vi "AgingControl.vi"(0 "IP adress":string="10.0.0.2", 2 "First Channel":u8(ring) items=["1", "2", "3", "4", "5", "6", "7", "8", "9", "10", "11", "12", "13", "14", "15", "16"], 4 "Exit":bool, 6 "Draw 2":enum16{"J(V)", "P(V)", "V(t)", "I(t)"}(ring) caption="Draw") -> (7 "XY Graph":T8(graph)={"ExchangeJVData"=[0.6447156, 0.5940376, 0.5406553, 0.48496604, 0.43833676, 0.39644372, 0.35270205, 0.30110732, 0.2324926, 0.19632894, 0.14613982, 0.08873936, 0.043943465, -0.010401342, -0.04554136, -0.10945036, -0.15922697, -0.20972164, -0.14604181, -0.097304136, -0.048933137, 0.00041567357, 0.047228295, 0.0906797, 0.15038718, 0.20405975, 0.25212517, 0.29427794, 0.3574383, 0.4079635, 0.45813736, 0.5003818, 0.55277103, 0.6010656, 0.64738935, 0.0833232, 0.032125723, -0.00891171, -0.06629689, -0.11847218, -0.16681261, -0.2017693, -0.1451022, -0.09281997, -0.05254645, 0.0022414266, 0.055532034, 0.08567607, 0.35597858, 0.3490164, 0.33783153, 0.32564417, 0.31237674, 0.30614087, 0.2953826, 0.28514028, 0.27568892, 0.2651622, 0.25504795, 0.24763331, 0.23487948, 0.22360058, 0.21352632, 0.20324053, 0.195364, 0.18436247, 0.1724654, 0.1645395, 0.15484014, 0.14352247, 0.13540854, 0.12296967, 0.24092051, 0.2318652, 0.22103643, 0.20964117, 0.20214543, 0.19041994, 0.18028222, 0.1693994, 0.15982696, 0.14702262, 0.14099239, 0.90037847, 0.8003987, 0.700059, 0.6002757, 0.4998595, 0.39971617, 0.299911, 0.19984399, 0.09990792, -0.00039909285, -0.100826114, -0.199933, -0.10054245, -0.0001699818, 0.10008249, 0.19999674, 0.30009645, 0.400098, 0.5005905, 0.59995925, 0.7005827, 0.79998416, 0.9002584, 1.1008824, 1.0004772, 0.9002902, 0.80020136, 0.6998943, 0.59989285, 0.49989128, 0.3998461, 0.2995609, 0.19967936, 0.09944872, -0.00043280495, -0.100914374, -0.1998249, -0.10005248, 3.5971088e-06, 0.100179695, 0.20012668, 0.30028096, 0.40050068, 0.5003604, 0.6004274, 0.700669, 0.8007905, 0.90092295, 1.0009027, 1.1013625], "ExchangeJVData"=[-0.0006814758307882585, -0.0016850824977154844, -0.003464073233772069, -0.004132507456233725, -0.006865448813186958, -0.009688151476439089, -0.010450167610542849, -0.012205285020172596, -0.01281928998650983, -0.01538607757538557, -0.01734554534777999, -0.01874734734883532, -0.02091021160595119, -0.023065433197189122, -0.025690472102724016, -0.027107552159577608, -0.029473809991031885, -0.030340865487232804, -0.02554819220677018, -0.020245595078449696, -0.017617693811189383, -0.014932497288100421, -0.011915947106899694, -0.010568575089564547, -0.00908369620447047, -0.008211866952478886, -0.007987464050529525, -0.005277439777273685, -0.005400622831075452, -0.004535477637546137, -0.0030124019758659415, -0.0015179738511506002, -0.0005382399194786558, 0.0027600066459854133, 0.0038887061236891896, 0.00010727677590693929, -0.00026513666853134055, -0.0005678420166077558, -0.0004885847829427803, -0.0005115025942359352, -0.0008065685506153386, -0.0004981338861398399, -0.0009154278814094141, -0.00034630377285793656, 0.0002839344460880966, -0.00023266989046533126, -0.0003959589321311796, 0.0006277007742028218, 0.0003016369646502426, 0.00021885389287490398, -0.0001957958147613681, 0.00045596452764584683, 0.00025638905754021835, 3.7788979057040706e-05, 0.0003583436637200066, -0.00014885848713674932, 0.00024169821699615568, -4.7932229563230067e-05, 5.387545911617053e-05, 0.000101914599781594, -0.00013739961559622316, 0.0004619877927325433, 3.73482350823906e-05, 7.290014423233515e-05, 3.338896092941468e-06, -0.0003274994242019602, 0.00024382839001191314, -0.0002237818989669904, -4.403914317663293e-05, 4.748494859541097e-05, -0.0005247977696853923, 0.00014040466567166732, 0.0003158870640618261, -0.00019440019514149753, -2.9047253491398806e-06, 0.00012850507573602954, -0.00042629549170669634, 0.000347986610904627, -0.0001858060272752482, 0.00010815821269716253, 9.662588809078443e-05, -0.0001724373305478366, 0.00013225123893789714, 0.028723286231979728, 0.013472377031575888, 0.0038900074287084863, 0.0005599445103143808, -0.00025432843813177897, -0.001567121762491297, -0.00263713354797801, -0.0038046669942559674, -0.004844672366743907, -0.005407297794590704, -0.0060606253100559115, -0.006378423859132454, -0.00500084352097474, -0.004116327909287065, -0.0034220814995933324, -0.002759206108748913, -0.0017260208551306278, -0.0011736246960936114, 0.00019440819869487314, 0.0023596650862600654, 0.005811800292576663, 0.011875201016664505, 0.02630160888656974, 0.25784142781049013, 0.1455090008676052, 0.06033926038071513, 0.018355286738369614, 0.0047029163397382945, 0.0004249142875778489, -0.0016735091776354238, -0.0026023530153906904, -0.003679184737848118, -0.004129284570808522, -0.004831714613828808, -0.0055211869039339945, -0.006160193879622966, -0.006821022543590516, -0.005202024840400554, -0.004168157101958059, -0.0032911433663684875, -0.002357525590923615, -0.0013100188880343921, -0.00010838676871571806, 0.0008879723282007035, 0.0023180647986009717, 0.0050629969337023795, 0.01595134090166539, 0.0550459953956306, 0.13187992153689265, 0.2366785192862153]}, 8 "Number of points":i32=133)   [LabVIEW 2020]
doc: "The VSCAN ( Potentiodynamic Technique) consists of scanning linearly the potential of a stationary working electrode with different scan rates.\nIn general, in this VI, the first thing to do is to start by establishing the connection with the instrument defined by its IP adress, then load the firmware in the channel selected, get the information on the plugged channels, load protocol on a channel, start/stop the protocol, retreive data and draw the graph."
uses:
  ActiveArray.vi
  <vilib>/Utility/file.llb/Write Delimited Spreadsheet (DBL).vi
  <vilib>/Utility/file.llb/Write Delimited Spreadsheet (string).vi
  AgingStatus.vi
  IntensityTemperature.vi
  StartStopPause.vi
panel:
  out "Array 2":string[](array[string])
  out "Array":string[](array[string])
  out "JVData 2":sgl[][](array[numeric])
  in  "DataForAnalysisE":T1 {"Eff" scale=0.0..30.0}
  out "AllPaused":bool
  out "WriteConfigTable":bool
  out "Boolean":bool=TRUE
  out "WriteAll":i32=-1
  out "output array":cluster{"JVData":sgl[][], "AgingData":sgl[][]}[](array[cluster])=[{"JVData"=array133x5[665 elements], "AgingData"=[[0.0, 0.25132346, 0.0, 1.0]]}, {"JVData"=array89x5[445 elements], "AgingData"=array682x3[2046 elements]}, {"JVData"=[[3.07914, 1.0002275, 9.958126e-09, 0.9997951, 1.0], [3.2463598, 0.95003825, 2.1757216e-08, 0.9520022, 1.0], [3.4136999, 0.89984906, 3.7805787e-08, 0.90010446, 1.0], [3.5809798, 0.8496599, -3.234939e-08, 0.8519322, 1.0], [3.74826, 0.7994708, 9.835428e-09, 0.79722506, 1.0], [3.91554, 0.74928164, -5.833279e-08, 0.7560611, 1.0], [4.08288, 0.6990925, -1.44667e-08, 0.6984071, 1.0], [4.2501597, 0.6489033, 1.3045136e-08, 0.64890647, 1.0], [4.41744, 0.5987142, 3.444323e-08, 0.6010701, 1.0], [4.5847797, 0.54852504, -3.4030673e-08, 0.5464241, 1.0], [4.75206, 0.49833587, 5.2020237e-08, 0.49976334, 1.0], [4.9193397, 0.44814673, 5.7064067e-08, 0.4450562, 1.0], [5.08662, 0.39795756, -9.57571e-09, 0.40031934, 1.0], [5.2539597, 0.34776843, 3.5207446e-08, 0.34518468, 1.0], [5.42124, 0.29757926, -2.0274754e-08, 0.30434132, 1.0], [5.58852, 0.2473901, -7.58874e-09, 0.24774085, 1.0], [5.75586, 0.19720097, 4.972759e-08, 0.19575147, 1.0], [5.92314, 0.14701182, -5.5581605e-08, 0.15440427, 1.0], [6.09042, 0.096822664, -3.1738015e-08, 0.099987194, 1.0], [6.2577, 0.046633508, -1.24797355e-08, 0.049051344, 1.0], [6.42504, -0.0035556422, -3.69347e-08, -0.0022356801, 1.0], [6.59232, -0.05374479, -2.699987e-08, -0.04924751, 1.0], [6.7595997, -0.10393394, -3.4336352e-08, -0.100366585, 1.0], [6.92694, -0.15412308, 2.7259583e-08, -0.15919624, 1.0], [7.0798197, -0.20000151, -7.9578044e-08, -0.1976577, 1.0], [7.2471, -0.14981236, -6.108396e-08, -0.1461722, 1.0], [7.4144397, -0.09962321, 4.926905e-08, -0.10051926, 1.0], [7.58172, -0.049434066, -4.2131372e-08, -0.046911426, 1.0], [7.7489996, 0.0007550822, -3.510057e-08, -0.00041872347, 1.0], [7.91628, 0.050944235, 1.0643253e-07, 0.044424977, 1.0], [8.08362, 0.101133384, -2.8528309e-08, 0.10162093, 1.0], [8.250899, 0.15132254, -2.2414564e-08, 0.15435848, 1.0], [8.4181795, 0.20151168, -4.0602938e-08, 0.20494314, 1.0], [8.58552, 0.25170085, -3.418351e-08, 0.25502396, 1.0], [8.7528, 0.30189, -1.1715516e-08, 0.30941048, 1.0], [8.92008, 0.35207915, 4.3308155e-08, 0.3432456, 1.0], [9.087359, 0.4022683, 2.2062904e-08, 0.39781532, 1.0], [9.2547, 0.45245743, -2.3178778e-08, 0.45491967, 1.0], [9.42198, 0.5026466, -6.016691e-08, 0.5006184, 1.0], [9.58926, 0.55283576, -1.1442636e-07, 0.56295985, 1.0]], "AgingData"=array326x3[978 elements]}, {"JVData"=[[3.0790799, 1.0001799, 5.3355116e-09, 0.9998571, 1.0], [3.2463, 0.9499914, -9.22995e-12, 0.9462215, 1.0], [3.41358, 0.8998029, -5.361627e-09, 0.9083466, 1.0], [3.58092, 0.8496145, -2.2642176e-08, 0.84980154, 1.0], [3.7482, 0.799426, 1.0688549e-07, 0.7932258, 1.0], [3.91548, 0.74923754, -1.759565e-08, 0.75158024, 1.0], [4.08276, 0.6990491, -2.914825e-09, 0.70146203, 1.0], [4.2500997, 0.64886063, 4.785635e-08, 0.6504126, 1.0], [4.41738, 0.59867215, 9.625048e-09, 0.5979435, 1.0], [4.58466, 0.54848367, -1.2396183e-08, 0.5513975, 1.0], [4.75194, 0.49829522, 6.345473e-08, 0.491906, 1.0], [4.91928, 0.44810674, 2.2011998e-08, 0.4528098, 1.0], [5.08656, 0.39791828, 4.0515943e-08, 0.3955777, 1.0], [5.25384, 0.3477298, 5.6878946e-08, 0.34668076, 1.0], [5.4211197, 0.29754135, -9.604628e-08, 0.30590534, 1.0], [5.58846, 0.24735287, 9.013345e-09, 0.24722293, 1.0], [5.7557397, 0.1971644, 5.9325743e-08, 0.19342564, 1.0], [5.92302, 0.14697593, -3.028844e-08, 0.15090989, 1.0], [6.0903, 0.09678746, -4.9251167e-08, 0.10161606, 1.0], [6.25764, 0.046598993, 1.4369164e-10, 0.04584945, 1.0], [6.4249196, -0.0035894734, -4.435756e-08, -0.00521524, 1.0], [6.5922, -0.053777937, 2.1317061e-09, -0.05450907, 1.0], [0.5082, -0.6647468, -1.2796141e-08, -0.6640006, 1.0], [1.0162799, -0.6545854, 3.784564e-08, -0.6567539, 1.0]], "AgingData"=array474x3[1422 elements]}, {"JVData"=[[3.0792599, 1.0001653, 5.946803e-09, 1.0001053, 1.0], [3.24648, 0.949974, -6.6066896e-08, 0.95460665, 1.0], [3.41382, 0.89978266, -6.530285e-08, 0.90336657, 1.0], [3.5811, 0.8495914, 8.6590035e-08, 0.84367305, 1.0], [3.7484398, 0.79940003, -2.1140826e-08, 0.7968202, 1.0], [3.91572, 0.7492087, -2.1446452e-08, 0.7541558, 1.0], [4.0829997, 0.6990174, -4.8188134e-08, 0.7052545, 1.0], [4.25034, 0.64882606, 1.1254829e-08, 0.65178263, 1.0], [4.4176197, 0.5986348, -5.8884844e-08, 0.6038444, 1.0], [4.58496, 0.54844344, 4.594265e-08, 0.54645914, 1.0], [4.7522397, 0.4982521, 2.1645896e-08, 0.5013795, 1.0], [4.91952, 0.44806078, 1.5046452e-07, 0.43668732, 1.0], [5.0868597, 0.39786944, -1.6707412e-07, 0.40697056, 1.0], [5.25414, 0.34767812, -4.331764e-09, 0.3509611, 1.0], [5.4214797, 0.2974868, 2.3938037e-08, 0.29353002, 1.0], [5.58876, 0.24729547, -2.5419501e-08, 0.2470593, 1.0], [5.7560396, 0.19710416, 6.9761557e-09, 0.19588034, 1.0], [5.92338, 0.14691283, -6.912309e-08, 0.15127456, 1.0], [6.0906596, 0.0967215, -1.7473404e-08, 0.09949945, 1.0], [6.258, 0.04653018, 1.4005404e-08, 0.04480463, 1.0], [6.4252796, -0.0036611457, -3.703305e-08, -0.0013145087, 1.0], [6.59256, -0.053852465, -5.5675827e-08, -0.051820844, 1.0], [6.7598996, -0.10404379, 5.2207838e-08, -0.10769272, 1.0], [6.92718, -0.15423511, -9.0688665e-09, -0.15569209, 1.0], [7.0801196, -0.20011552, -1.8868072e-09, -0.20259082, 1.0], [7.2474, -0.14992419, 3.1731343e-08, -0.151259, 1.0], [7.4147396, -0.099732876, -1.5792498e-08, -0.098383285, 1.0], [7.58202, -0.049541555, 8.9646235e-08, -0.056819506, 1.0], [7.7493596, 0.00064976525, 2.2409939e-08, -0.0017731013, 1.0], [7.91664, 0.05084109, -3.1073473e-08, 0.055077106, 1.0], [8.08392, 0.10103241, 7.497649e-08, 0.09262056, 1.0], [8.25126, 0.15122373, 2.7147042e-08, 0.15106057, 1.0], [8.41854, 0.20141506, -4.085329e-08, 0.206856, 1.0], [8.585879, 0.2516064, -2.7558846e-08, 0.25670502, 1.0], [8.7531595, 0.30179772, 2.5466141e-08, 0.30317575, 1.0], [8.92044, 0.35198903, -5.1702784e-08, 0.36140174, 1.0], [9.08778, 0.40218034, -4.6354437e-08, 0.40365338, 1.0], [9.25506, 0.4523717, -9.374485e-09, 0.4568654, 1.0], [9.4223995, 0.502563, 9.0104656e-08, 0.49687, 1.0], [9.58968, 0.55275434, 6.764162e-08, 0.5450987, 1.0], [9.75696, 0.6029457, 5.2952487e-09, 0.60003805, 1.0], [9.9243, 0.65313697, -2.9239741e-08, 0.65580297, 1.0], [10.091579, 0.7033283, 9.971579e-11, 0.70409274, 1.0], [3.0948598, -0.5967237, 1.23362565e-08, -0.5965496, 1.0]], "AgingData"=array342x3[1026 elements]}, {"JVData"=[[0.16746, 0.9498421, -3.7238106e-08, 0.9521123, 1.0], [0.3348, 0.899643, -6.0527117e-09, 0.9032217, 1.0], [0.50207996, 0.849444, -6.093289e-08, 0.85836333, 1.0], [0.66942, 0.79924494, -7.89715e-08, 0.80652505, 1.0], [0.83676, 0.7490459, 3.30819e-08, 0.752304, 1.0], [1.0041, 0.6988469, 7.552681e-09, 0.6958531, 1.0]], "AgingData"=[[0.0, -0.27385262, -0.00088946975], [0.0, -0.5112182, 0.0004154984], [2.0, -0.06918946, 7.042664e-05], [4.0, -0.093550734, -8.228485e-05], [0.0, -0.61836976, 5.6613615e-05], [2.0, -0.5800316, -0.00027317417], [4.0, -0.5014493, -4.4106928e-05], [6.0, -0.36604953, -0.00019681842], [8.0, -0.23225343, 3.224882e-05], [10.0, -0.2007136, -4.4106928e-05], [12.0, -0.2059066, 0.00010860457], [14.0, -0.20323373, 0.00010860457], [16.0, -0.21033593, -0.00027317417], [18.0, -0.21904184, 3.224882e-05], [20.0, -0.23691186, 0.00010860457], [22.0, -0.2476797, 3.224882e-05], [0.0, -0.27289036, 7.493925e-05], [2.0, -0.28011072, -2.5781526e-05], [4.0, -0.28629652, -0.000102137274], [6.0, -0.2959952, -2.5781526e-05], [8.0, -0.3174545, -0.000102137274], [10.0, -0.33226982, 0.00020328572], [12.0, -0.37259194, 0.00012692997], [14.0, -0.51142824, 0.00020328572]]}, {"JVData"=[[0.50838, -0.7533297, 3.3713125e-08, -0.754186, 1.0], [1.01658, -0.74316514, -1.8526524e-08, -0.7415677, 1.0], [1.52484, -0.7330006, -1.3213221e-08, -0.730666, 1.0], [2.03304, -0.7228361, -2.0536646e-08, -0.7224946, 1.0], [2.54124, -0.7126715, -4.6319983e-09, -0.7157485, 1.0], [3.0495, -0.70250696, 2.0711987e-08, -0.70280004, 1.0], [3.5577, -0.69234246, -1.360114e-08, -0.69154114, 1.0], [4.06596, -0.6821779, 1.00148485e-08, -0.68209034, 1.0]], "AgingData"=[[0.0, -0.10874961, -0.0005815154], [2.0, -0.37434164, -4.2873908e-05], [4.0, -0.5594564, -0.00011923032], [0.0, -1.571388, -0.0021865703], [2.0, -0.9579511, 0.00010831172], [4.0, -0.8996827, -0.00019711393], [0.0, -0.81472254, -0.0005532635], [2.0, -0.7945132, -0.00024369123], [4.0, -0.7643481, -9.0978414e-05], [6.0, -0.67538, -1.46220045e-05], [8.0, -0.58190614, -9.0978414e-05], [10.0, -0.5370021, -9.0978414e-05], [12.0, -0.53486377, 0.00021444722], [14.0, -0.5418896, -0.00032004766], [16.0, -0.5460135, -9.0978414e-05], [18.0, -0.5487627, -1.46220045e-05], [20.0, -0.5612869, 6.1734405e-05], [22.0, -0.5698401, -1.46220045e-05], [0.0, -0.7470461, -0.0005593721], [2.0, -0.81696755, 0.0001319822], [4.0, -0.88157445, -9.708702e-05], [6.0, -0.9173908, 5.5625802e-05], [8.0, -0.94289756, -0.00017344343], [10.0, -0.9694734, -2.0730608e-05], [12.0, -0.9618367, -9.708702e-05], [14.0, -0.94824326, 0.000284695]]}, {"JVData"=[[0.1674, 0.94984764, -2.53673e-08, 0.95032424, 1.0], [0.33468, 0.89965886, 2.5059206e-08, 0.90274954, 1.0], [0.50202, 0.84947014, 4.599384e-08, 0.8470317, 1.0], [0.66929996, 0.7992814, 2.8115352e-08, 0.80051106, 1.0], [0.83658, 0.7490927, 7.716658e-08, 0.74543494, 1.0], [1.00392, 0.698904, 1.527952e-08, 0.69605744, 1.0], [1.1711999, 0.64871526, -8.1294864e-08, 0.65673256, 1.0], [1.33848, 0.59852654, -2.446165e-09, 0.5987537, 1.0], [1.50576, 0.5483378, 1.2223366e-08, 0.54815394, 1.0], [1.6731, 0.49814907, -1.2237014e-09, 0.4994944, 1.0], [1.84038, 0.44796032, -4.5385075e-08, 0.45431826, 1.0], [2.00766, 0.3977716, 7.518008e-08, 0.39097688, 1.0], [2.1749399, 0.34758288, -7.029272e-08, 0.3521104, 1.0], [2.34228, 0.29739416, -8.037802e-08, 0.30120507, 1.0], [2.5095599, 0.2472054, 1.1764944e-08, 0.25023863, 1.0], [2.6768398, 0.19701669, -3.5605403e-08, 0.2051541, 1.0], [2.84412, 0.14682795, -6.295796e-08, 0.14795439, 1.0], [3.0114598, 0.09663922, -1.0708939e-09, 0.095765725, 1.0], [3.17874, 0.046450496, 3.590854e-08, 0.046586785, 1.0], [3.34602, -0.003738234, 2.9490622e-08, -0.0043338123, 1.0], [3.5133, -0.05392696, -3.8355942e-08, -0.042894743, 1.0], [3.68064, -0.10411569, 2.4600778e-08, -0.10817639, 1.0], [3.84792, -0.15430441, -1.6821268e-09, -0.15341367, 1.0], [3.9998398, -0.19987454, -4.4315435e-08, -0.19512181, 1.0], [4.16712, -0.14968581, -1.1920225e-08, -0.1442165, 1.0], [4.3343997, -0.09949709, 1.1827183e-07, -0.11188886, 1.0], [4.50174, -0.049308363, 3.207719e-09, -0.047019724, 1.0], [4.6690197, 0.00088036037, 1.2209202e-07, -0.00674769, 1.0], [4.8363, 0.05106909, 6.569485e-09, 0.054225642, 1.0], [5.0036397, 0.101257816, 3.5133425e-09, 0.10215181, 1.0], [5.17092, 0.15144655, 1.0848095e-08, 0.15154463, 1.0], [5.3382, 0.20163527, 1.1459326e-08, 0.20368746, 1.0], [5.50548, 0.25182402, -1.7115688e-08, 0.25315666, 1.0], [5.67282, 0.30201274, 6.264987e-08, 0.29463565, 1.0], [5.8401, 0.35220146, 1.7877248e-08, 0.350934, 1.0], [6.00738, 0.40239018, -3.224364e-08, 0.40428376, 1.0], [6.1746597, 0.45257893, 4.8886095e-09, 0.4554946, 1.0], [6.342, 0.5027677, -4.0648054e-08, 0.5062319, 1.0], [6.5092797, 0.5529564, 1.4821096e-08, 0.55712193, 1.0], [6.67656, 0.6031451, -1.3448305e-08, 0.60238975, 1.0], [6.8438396, 0.65333384, -1.1920232e-08, 0.6556937, 1.0], [7.01118, 0.70352256, 1.1764944e-08, 0.7035129, 1.0], [7.1784596, 0.7537113, 7.73194e-08, 0.74700856, 1.0]], "AgingData"=array258x4[1032 elements]}, {"JVData"=[[1.0013499, 1.210579e-05, 1.1001669, 1.0], [2.00265, 5.280055e-06, 1.0000192, 1.0], [3.0038998, 7.4926476e-07, 0.8999563, 1.0], [4.00515, 5.459907e-08, 0.7997196, 1.0], [5.0064, -1.6849775e-07, 0.6995634, 1.0], [6.0077, -3.4968886e-07, 0.5993691, 1.0], [7.0089498, -5.469176e-07, 0.49931043, 1.0], [8.0102, -7.4393e-07, 0.39910764, 1.0], [9.01145, -9.556986e-07, 0.29895997, 1.0], [10.01275, -1.2210978e-06, 0.19898194, 1.0], [11.014, -1.4915547e-06, 0.098842725, 1.0], [12.015249, -1.7013582e-06, -0.0013897662, 1.0], [13.0164995, -1.8637089e-06, -0.101503514, 1.0]], "AgingData"=[[0.2513, 5.4381195e-05, 1.0503782, 1.0], [0.5025, 2.778111e-05, 1.0002986, 1.0], [0.75369996, 3.9110714e-06, 0.94982845, 1.0], [1.0049, -2.2766604e-05, 0.8997149, 1.0], [1.2560999, -5.2547082e-05, 0.8493892, 1.0], [1.5073, -8.9432746e-05, 0.7991992, 1.0], [1.7585, -0.00013286466, 0.74895835, 1.0], [2.0097, -0.00018626524, 0.6987514, 1.0], [2.2609, -0.00024645546, 0.6484681, 1.0], [2.5121, -0.0003150903, 0.5982187, 1.0], [2.7633, -0.0003903196, 0.5479184, 1.0], [3.0144498, -0.00046932563, 0.49767745, 1.0], [3.26565, -0.0005563859, 0.44752148, 1.0], [3.51685, -0.00064487197, 0.397323, 1.0], [3.76805, -0.00073117693, 0.34696326, 1.0], [4.01925, -0.0008170999, 0.29672235, 1.0], [4.27045, -0.0009031756, 0.24646449, 1.0], [4.52165, -0.0009820798, 0.19614716, 1.0], [4.77285, -0.0010612556, 0.14594024, 1.0], [5.0240498, -0.0011366602, 0.0958352, 1.0], [5.27525, -0.0012121152, 0.04556884, 1.0], [5.5264497, -0.0012991133, -0.0047399844, 1.0], [5.77765, -0.0013793214, -0.05493842, 1.0], [6.02885, -0.0014648766, -0.10519629, 1.0], [6.28005, -0.001559259, -0.15536925, 1.0], [6.53125, -0.001651095, -0.20566109, 1.0], [6.7824497, -0.0017487028, -0.255885, 1.0]]}, {"JVData"=[[1.0013499, 1.210579e-05, 1.1001669, 1.0], [2.00265, 5.280055e-06, 1.0000192, 1.0], [3.0038998, 7.4926476e-07, 0.8999563, 1.0], [4.00515, 5.459907e-08, 0.7997196, 1.0], [5.0064, -1.6849775e-07, 0.6995634, 1.0], [6.0077, -3.4968886e-07, 0.5993691, 1.0], [7.0089498, -5.469176e-07, 0.49931043, 1.0], [8.0102, -7.4393e-07, 0.39910764, 1.0], [9.01145, -9.556986e-07, 0.29895997, 1.0], [10.01275, -1.2210978e-06, 0.19898194, 1.0], [11.014, -1.4915547e-06, 0.098842725, 1.0], [12.015249, -1.7013582e-06, -0.0013897662, 1.0], [13.0164995, -1.8637089e-06, -0.101503514, 1.0]], "AgingData"=[[0.2513, 5.4381195e-05, 1.0503782, 1.0], [0.5025, 2.778111e-05, 1.0002986, 1.0], [0.75369996, 3.9110714e-06, 0.94982845, 1.0], [1.0049, -2.2766604e-05, 0.8997149, 1.0], [1.2560999, -5.2547082e-05, 0.8493892, 1.0], [1.5073, -8.9432746e-05, 0.7991992, 1.0], [1.7585, -0.00013286466, 0.74895835, 1.0], [2.0097, -0.00018626524, 0.6987514, 1.0], [2.2609, -0.00024645546, 0.6484681, 1.0], [2.5121, -0.0003150903, 0.5982187, 1.0], [2.7633, -0.0003903196, 0.5479184, 1.0], [3.0144498, -0.00046932563, 0.49767745, 1.0], [3.26565, -0.0005563859, 0.44752148, 1.0], [3.51685, -0.00064487197, 0.397323, 1.0], [3.76805, -0.00073117693, 0.34696326, 1.0], [4.01925, -0.0008170999, 0.29672235, 1.0], [4.27045, -0.0009031756, 0.24646449, 1.0], [4.52165, -0.0009820798, 0.19614716, 1.0], [4.77285, -0.0010612556, 0.14594024, 1.0], [5.0240498, -0.0011366602, 0.0958352, 1.0], [5.27525, -0.0012121152, 0.04556884, 1.0], [5.5264497, -0.0012991133, -0.0047399844, 1.0], [5.77765, -0.0013793214, -0.05493842, 1.0], [6.02885, -0.0014648766, -0.10519629, 1.0], [6.28005, -0.001559259, -0.15536925, 1.0], [6.53125, -0.001651095, -0.20566109, 1.0], [6.7824497, -0.0017487028, -0.255885, 1.0]]}, {"JVData"=[[1.0013499, 1.210579e-05, 1.1001669, 1.0], [2.00265, 5.280055e-06, 1.0000192, 1.0], [3.0038998, 7.4926476e-07, 0.8999563, 1.0], [4.00515, 5.459907e-08, 0.7997196, 1.0], [5.0064, -1.6849775e-07, 0.6995634, 1.0], [6.0077, -3.4968886e-07, 0.5993691, 1.0], [7.0089498, -5.469176e-07, 0.49931043, 1.0], [8.0102, -7.4393e-07, 0.39910764, 1.0], [9.01145, -9.556986e-07, 0.29895997, 1.0], [10.01275, -1.2210978e-06, 0.19898194, 1.0], [11.014, -1.4915547e-06, 0.098842725, 1.0], [12.015249, -1.7013582e-06, -0.0013897662, 1.0], [13.0164995, -1.8637089e-06, -0.101503514, 1.0]], "AgingData"=[[0.2513, 5.4381195e-05, 1.0503782, 1.0], [0.5025, 2.778111e-05, 1.0002986, 1.0], [0.75369996, 3.9110714e-06, 0.94982845, 1.0], [1.0049, -2.2766604e-05, 0.8997149, 1.0], [1.2560999, -5.2547082e-05, 0.8493892, 1.0], [1.5073, -8.9432746e-05, 0.7991992, 1.0], [1.7585, -0.00013286466, 0.74895835, 1.0], [2.0097, -0.00018626524, 0.6987514, 1.0], [2.2609, -0.00024645546, 0.6484681, 1.0], [2.5121, -0.0003150903, 0.5982187, 1.0], [2.7633, -0.0003903196, 0.5479184, 1.0], [3.0144498, -0.00046932563, 0.49767745, 1.0], [3.26565, -0.0005563859, 0.44752148, 1.0], [3.51685, -0.00064487197, 0.397323, 1.0], [3.76805, -0.00073117693, 0.34696326, 1.0], [4.01925, -0.0008170999, 0.29672235, 1.0], [4.27045, -0.0009031756, 0.24646449, 1.0], [4.52165, -0.0009820798, 0.19614716, 1.0], [4.77285, -0.0010612556, 0.14594024, 1.0], [5.0240498, -0.0011366602, 0.0958352, 1.0], [5.27525, -0.0012121152, 0.04556884, 1.0], [5.5264497, -0.0012991133, -0.0047399844, 1.0], [5.77765, -0.0013793214, -0.05493842, 1.0], [6.02885, -0.0014648766, -0.10519629, 1.0], [6.28005, -0.001559259, -0.15536925, 1.0], [6.53125, -0.001651095, -0.20566109, 1.0], [6.7824497, -0.0017487028, -0.255885, 1.0]]}, {"JVData"=[[1.0013499, 1.210579e-05, 1.1001669, 1.0], [2.00265, 5.280055e-06, 1.0000192, 1.0], [3.0038998, 7.4926476e-07, 0.8999563, 1.0], [4.00515, 5.459907e-08, 0.7997196, 1.0], [5.0064, -1.6849775e-07, 0.6995634, 1.0], [6.0077, -3.4968886e-07, 0.5993691, 1.0], [7.0089498, -5.469176e-07, 0.49931043, 1.0], [8.0102, -7.4393e-07, 0.39910764, 1.0], [9.01145, -9.556986e-07, 0.29895997, 1.0], [10.01275, -1.2210978e-06, 0.19898194, 1.0], [11.014, -1.4915547e-06, 0.098842725, 1.0], [12.015249, -1.7013582e-06, -0.0013897662, 1.0], [13.0164995, -1.8637089e-06, -0.101503514, 1.0]], "AgingData"=[[0.2513, 5.4381195e-05, 1.0503782, 1.0], [0.5025, 2.778111e-05, 1.0002986, 1.0], [0.75369996, 3.9110714e-06, 0.94982845, 1.0], [1.0049, -2.2766604e-05, 0.8997149, 1.0], [1.2560999, -5.2547082e-05, 0.8493892, 1.0], [1.5073, -8.9432746e-05, 0.7991992, 1.0], [1.7585, -0.00013286466, 0.74895835, 1.0], [2.0097, -0.00018626524, 0.6987514, 1.0], [2.2609, -0.00024645546, 0.6484681, 1.0], [2.5121, -0.0003150903, 0.5982187, 1.0], [2.7633, -0.0003903196, 0.5479184, 1.0], [3.0144498, -0.00046932563, 0.49767745, 1.0], [3.26565, -0.0005563859, 0.44752148, 1.0], [3.51685, -0.00064487197, 0.397323, 1.0], [3.76805, -0.00073117693, 0.34696326, 1.0], [4.01925, -0.0008170999, 0.29672235, 1.0], [4.27045, -0.0009031756, 0.24646449, 1.0], [4.52165, -0.0009820798, 0.19614716, 1.0], [4.77285, -0.0010612556, 0.14594024, 1.0], [5.0240498, -0.0011366602, 0.0958352, 1.0], [5.27525, -0.0012121152, 0.04556884, 1.0], [5.5264497, -0.0012991133, -0.0047399844, 1.0], [5.77765, -0.0013793214, -0.05493842, 1.0], [6.02885, -0.0014648766, -0.10519629, 1.0], [6.28005, -0.001559259, -0.15536925, 1.0], [6.53125, -0.001651095, -0.20566109, 1.0], [6.7824497, -0.0017487028, -0.255885, 1.0]]}, {"JVData"=[[1.0013499, 1.210579e-05, 1.1001669, 1.0], [2.00265, 5.280055e-06, 1.0000192, 1.0], [3.0038998, 7.4926476e-07, 0.8999563, 1.0], [4.00515, 5.459907e-08, 0.7997196, 1.0], [5.0064, -1.6849775e-07, 0.6995634, 1.0], [6.0077, -3.4968886e-07, 0.5993691, 1.0], [7.0089498, -5.469176e-07, 0.49931043, 1.0], [8.0102, -7.4393e-07, 0.39910764, 1.0], [9.01145, -9.556986e-07, 0.29895997, 1.0], [10.01275, -1.2210978e-06, 0.19898194, 1.0], [11.014, -1.4915547e-06, 0.098842725, 1.0], [12.015249, -1.7013582e-06, -0.0013897662, 1.0], [13.0164995, -1.8637089e-06, -0.101503514, 1.0]], "AgingData"=[[0.2513, 5.4381195e-05, 1.0503782, 1.0], [0.5025, 2.778111e-05, 1.0002986, 1.0], [0.75369996, 3.9110714e-06, 0.94982845, 1.0], [1.0049, -2.2766604e-05, 0.8997149, 1.0], [1.2560999, -5.2547082e-05, 0.8493892, 1.0], [1.5073, -8.9432746e-05, 0.7991992, 1.0], [1.7585, -0.00013286466, 0.74895835, 1.0], [2.0097, -0.00018626524, 0.6987514, 1.0], [2.2609, -0.00024645546, 0.6484681, 1.0], [2.5121, -0.0003150903, 0.5982187, 1.0], [2.7633, -0.0003903196, 0.5479184, 1.0], [3.0144498, -0.00046932563, 0.49767745, 1.0], [3.26565, -0.0005563859, 0.44752148, 1.0], [3.51685, -0.00064487197, 0.397323, 1.0], [3.76805, -0.00073117693, 0.34696326, 1.0], [4.01925, -0.0008170999, 0.29672235, 1.0], [4.27045, -0.0009031756, 0.24646449, 1.0], [4.52165, -0.0009820798, 0.19614716, 1.0], [4.77285, -0.0010612556, 0.14594024, 1.0], [5.0240498, -0.0011366602, 0.0958352, 1.0], [5.27525, -0.0012121152, 0.04556884, 1.0], [5.5264497, -0.0012991133, -0.0047399844, 1.0], [5.77765, -0.0013793214, -0.05493842, 1.0], [6.02885, -0.0014648766, -0.10519629, 1.0], [6.28005, -0.001559259, -0.15536925, 1.0], [6.53125, -0.001651095, -0.20566109, 1.0], [6.7824497, -0.0017487028, -0.255885, 1.0]]}, {"JVData"=[[1.0013499, 1.210579e-05, 1.1001669, 1.0], [2.00265, 5.280055e-06, 1.0000192, 1.0], [3.0038998, 7.4926476e-07, 0.8999563, 1.0], [4.00515, 5.459907e-08, 0.7997196, 1.0], [5.0064, -1.6849775e-07, 0.6995634, 1.0], [6.0077, -3.4968886e-07, 0.5993691, 1.0], [7.0089498, -5.469176e-07, 0.49931043, 1.0], [8.0102, -7.4393e-07, 0.39910764, 1.0], [9.01145, -9.556986e-07, 0.29895997, 1.0], [10.01275, -1.2210978e-06, 0.19898194, 1.0], [11.014, -1.4915547e-06, 0.098842725, 1.0], [12.015249, -1.7013582e-06, -0.0013897662, 1.0], [13.0164995, -1.8637089e-06, -0.101503514, 1.0]], "AgingData"=[[0.2513, 5.4381195e-05, 1.0503782, 1.0], [0.5025, 2.778111e-05, 1.0002986, 1.0], [0.75369996, 3.9110714e-06, 0.94982845, 1.0], [1.0049, -2.2766604e-05, 0.8997149, 1.0], [1.2560999, -5.2547082e-05, 0.8493892, 1.0], [1.5073, -8.9432746e-05, 0.7991992, 1.0], [1.7585, -0.00013286466, 0.74895835, 1.0], [2.0097, -0.00018626524, 0.6987514, 1.0], [2.2609, -0.00024645546, 0.6484681, 1.0], [2.5121, -0.0003150903, 0.5982187, 1.0], [2.7633, -0.0003903196, 0.5479184, 1.0], [3.0144498, -0.00046932563, 0.49767745, 1.0], [3.26565, -0.0005563859, 0.44752148, 1.0], [3.51685, -0.00064487197, 0.397323, 1.0], [3.76805, -0.00073117693, 0.34696326, 1.0], [4.01925, -0.0008170999, 0.29672235, 1.0], [4.27045, -0.0009031756, 0.24646449, 1.0], [4.52165, -0.0009820798, 0.19614716, 1.0], [4.77285, -0.0010612556, 0.14594024, 1.0], [5.0240498, -0.0011366602, 0.0958352, 1.0], [5.27525, -0.0012121152, 0.04556884, 1.0], [5.5264497, -0.0012991133, -0.0047399844, 1.0], [5.77765, -0.0013793214, -0.05493842, 1.0], [6.02885, -0.0014648766, -0.10519629, 1.0], [6.28005, -0.001559259, -0.15536925, 1.0], [6.53125, -0.001651095, -0.20566109, 1.0], [6.7824497, -0.0017487028, -0.255885, 1.0]]}, {"JVData"=[[1.0013499, 1.210579e-05, 1.1001669, 1.0], [2.00265, 5.280055e-06, 1.0000192, 1.0], [3.0038998, 7.4926476e-07, 0.8999563, 1.0], [4.00515, 5.459907e-08, 0.7997196, 1.0], [5.0064, -1.6849775e-07, 0.6995634, 1.0], [6.0077, -3.4968886e-07, 0.5993691, 1.0], [7.0089498, -5.469176e-07, 0.49931043, 1.0], [8.0102, -7.4393e-07, 0.39910764, 1.0], [9.01145, -9.556986e-07, 0.29895997, 1.0], [10.01275, -1.2210978e-06, 0.19898194, 1.0], [11.014, -1.4915547e-06, 0.098842725, 1.0], [12.015249, -1.7013582e-06, -0.0013897662, 1.0], [13.0164995, -1.8637089e-06, -0.101503514, 1.0]], "AgingData"=[[0.2513, 5.4381195e-05, 1.0503782, 1.0], [0.5025, 2.778111e-05, 1.0002986, 1.0], [0.75369996, 3.9110714e-06, 0.94982845, 1.0], [1.0049, -2.2766604e-05, 0.8997149, 1.0], [1.2560999, -5.2547082e-05, 0.8493892, 1.0], [1.5073, -8.9432746e-05, 0.7991992, 1.0], [1.7585, -0.00013286466, 0.74895835, 1.0], [2.0097, -0.00018626524, 0.6987514, 1.0], [2.2609, -0.00024645546, 0.6484681, 1.0], [2.5121, -0.0003150903, 0.5982187, 1.0], [2.7633, -0.0003903196, 0.5479184, 1.0], [3.0144498, -0.00046932563, 0.49767745, 1.0], [3.26565, -0.0005563859, 0.44752148, 1.0], [3.51685, -0.00064487197, 0.397323, 1.0], [3.76805, -0.00073117693, 0.34696326, 1.0], [4.01925, -0.0008170999, 0.29672235, 1.0], [4.27045, -0.0009031756, 0.24646449, 1.0], [4.52165, -0.0009820798, 0.19614716, 1.0], [4.77285, -0.0010612556, 0.14594024, 1.0], [5.0240498, -0.0011366602, 0.0958352, 1.0], [5.27525, -0.0012121152, 0.04556884, 1.0], [5.5264497, -0.0012991133, -0.0047399844, 1.0], [5.77765, -0.0013793214, -0.05493842, 1.0], [6.02885, -0.0014648766, -0.10519629, 1.0], [6.28005, -0.001559259, -0.15536925, 1.0], [6.53125, -0.001651095, -0.20566109, 1.0], [6.7824497, -0.0017487028, -0.255885, 1.0]]}, {"JVData"=[[1.0013499, 1.210579e-05, 1.1001669, 1.0], [2.00265, 5.280055e-06, 1.0000192, 1.0], [3.0038998, 7.4926476e-07, 0.8999563, 1.0], [4.00515, 5.459907e-08, 0.7997196, 1.0], [5.0064, -1.6849775e-07, 0.6995634, 1.0], [6.0077, -3.4968886e-07, 0.5993691, 1.0], [7.0089498, -5.469176e-07, 0.49931043, 1.0], [8.0102, -7.4393e-07, 0.39910764, 1.0], [9.01145, -9.556986e-07, 0.29895997, 1.0], [10.01275, -1.2210978e-06, 0.19898194, 1.0], [11.014, -1.4915547e-06, 0.098842725, 1.0], [12.015249, -1.7013582e-06, -0.0013897662, 1.0], [13.0164995, -1.8637089e-06, -0.101503514, 1.0]], "AgingData"=[[0.2513, 5.4381195e-05, 1.0503782, 1.0], [0.5025, 2.778111e-05, 1.0002986, 1.0], [0.75369996, 3.9110714e-06, 0.94982845, 1.0], [1.0049, -2.2766604e-05, 0.8997149, 1.0], [1.2560999, -5.2547082e-05, 0.8493892, 1.0], [1.5073, -8.9432746e-05, 0.7991992, 1.0], [1.7585, -0.00013286466, 0.74895835, 1.0], [2.0097, -0.00018626524, 0.6987514, 1.0], [2.2609, -0.00024645546, 0.6484681, 1.0], [2.5121, -0.0003150903, 0.5982187, 1.0], [2.7633, -0.0003903196, 0.5479184, 1.0], [3.0144498, -0.00046932563, 0.49767745, 1.0], [3.26565, -0.0005563859, 0.44752148, 1.0], [3.51685, -0.00064487197, 0.397323, 1.0], [3.76805, -0.00073117693, 0.34696326, 1.0], [4.01925, -0.0008170999, 0.29672235, 1.0], [4.27045, -0.0009031756, 0.24646449, 1.0], [4.52165, -0.0009820798, 0.19614716, 1.0], [4.77285, -0.0010612556, 0.14594024, 1.0], [5.0240498, -0.0011366602, 0.0958352, 1.0], [5.27525, -0.0012121152, 0.04556884, 1.0], [5.5264497, -0.0012991133, -0.0047399844, 1.0], [5.77765, -0.0013793214, -0.05493842, 1.0], [6.02885, -0.0014648766, -0.10519629, 1.0], [6.28005, -0.001559259, -0.15536925, 1.0], [6.53125, -0.001651095, -0.20566109, 1.0], [6.7824497, -0.0017487028, -0.255885, 1.0]]}]
  in  "Channel Names":string[](array[string])=["Ch2_Device1", "Ch2_Device2", "Ch3_Device3", "Ch4_Device4", "Ch5_Device5", "Ch6_Device6", "Ch7_Device7", "Ch8_Device8", "", "", "", "", "", "", "", "", " "]
  in  "ChannelAgingData":cluster{"AgingData":sgl[][]}[](array[cluster])=[{"AgingData"=[]}, {"AgingData"=[]}, {"AgingData"=[]}, {"AgingData"=[]}, {"AgingData"=[]}, {"AgingData"=[]}, {"AgingData"=[]}, {"AgingData"=[]}, {"AgingData"=[]}, {"AgingData"=[]}, {"AgingData"=[]}, {"AgingData"=[]}, {"AgingData"=[]}, {"AgingData"=[]}, {"AgingData"=[]}, {"AgingData"=[[0.0, 0.0, 0.0, 0.0, 0.0, 0.0]]}]
  in  "ChannelData":T2(array[cluster])=[{"JV metrics"=[[0.0001389722, 0.5796433, 0.0055181994, 0.34457082, 0.0011021399, 0.2995609, 0.0036791847, 0.41136372, 0.0041681943, 0.2751614, 0.00047180377, 0.20012668, 0.0023575255, 2.3360133, 200.0, 100.0, -300.0]], "JVData"=[[0.50064, 1.1008824, 0.25784144], [1.00104, 1.0004772, 0.145509], [1.5015, 0.9002902, 0.06033926], [2.00196, 0.80020136, 0.018355288], [2.50242, 0.6998943, 0.0047029164], [3.0028799, 0.59989285, 0.0004249143], [3.50334, 0.49989128, -0.0016735091], [4.0038, 0.3998461, -0.002602353], [4.50426, 0.2995609, -0.0036791847], [5.0047197, 0.19967936, -0.0041292845], [5.50518, 0.09944872, -0.004831715], [6.00558, -0.00043280495, -0.005521187], [6.5060396, -0.100914374, -0.006160194], [7.00032, -0.1998249, -0.006821023], [7.5008397, -0.10005248, -0.0052020247], [8.00124, 3.5971088e-06, -0.004168157], [8.501699, 0.100179695, -0.0032911433], [9.00216, 0.20012668, -0.0023575255], [9.50262, 0.30028096, -0.0013100188], [10.003079, 0.40050068, -0.00010838677], [10.50354, 0.5003604, 0.00088797236], [11.004, 0.6004274, 0.002318065], [11.504459, 0.700669, 0.005062997], [12.00492, 0.8007905, 0.015951341], [12.50538, 0.90092295, 0.055045996], [13.005779, 1.0009027, 0.13187993], [13.50624, 1.1013625, 0.23667851]]}, {"JV metrics"=[], "JVData"=[]}, {"JV metrics"=[], "JVData"=[]}, {"JV metrics"=[], "JVData"=[]}, {"JV metrics"=[], "JVData"=[]}, {"JV metrics"=[], "JVData"=[]}, {"JV metrics"=[], "JVData"=[]}, {"JV metrics"=[], "JVData"=[]}, {"JV metrics"=[[0.0, 0.0], [0.0, 0.0]], "JVData"=[[0.2513, 5.4381195e-05, 1.0503782, 1.0], [0.5025, 2.778111e-05, 1.0002986, 1.0], [0.75369996, 3.9110714e-06, 0.94982845, 1.0], [1.0049, -2.2766604e-05, 0.8997149, 1.0], [1.2560999, -5.2547082e-05, 0.8493892, 1.0], [1.5073, -8.9432746e-05, 0.7991992, 1.0], [1.7585, -0.00013286466, 0.74895835, 1.0], [2.0097, -0.00018626524, 0.6987514, 1.0], [2.2609, -0.00024645546, 0.6484681, 1.0], [2.5121, -0.0003150903, 0.5982187, 1.0], [2.7633, -0.0003903196, 0.5479184, 1.0], [3.0144498, -0.00046932563, 0.49767745, 1.0], [3.26565, -0.0005563859, 0.44752148, 1.0], [3.51685, -0.00064487197, 0.397323, 1.0], [3.76805, -0.00073117693, 0.34696326, 1.0], [4.01925, -0.0008170999, 0.29672235, 1.0], [4.27045, -0.0009031756, 0.24646449, 1.0], [4.52165, -0.0009820798, 0.19614716, 1.0], [4.77285, -0.0010612556, 0.14594024, 1.0], [5.0240498, -0.0011366602, 0.0958352, 1.0], [5.27525, -0.0012121152, 0.04556884, 1.0], [5.5264497, -0.0012991133, -0.0047399844, 1.0], [5.77765, -0.0013793214, -0.05493842, 1.0], [6.02885, -0.0014648766, -0.10519629, 1.0], [6.28005, -0.001559259, -0.15536925, 1.0], [6.53125, -0.001651095, -0.20566109, 1.0], [6.7824497, -0.0017487028, -0.255885, 1.0]]}, {"JV metrics"=[[0.0, 0.0], [0.0, 0.0]], "JVData"=[[0.2513, 5.4381195e-05, 1.0503782, 1.0], [0.5025, 2.778111e-05, 1.0002986, 1.0], [0.75369996, 3.9110714e-06, 0.94982845, 1.0], [1.0049, -2.2766604e-05, 0.8997149, 1.0], [1.2560999, -5.2547082e-05, 0.8493892, 1.0], [1.5073, -8.9432746e-05, 0.7991992, 1.0], [1.7585, -0.00013286466, 0.74895835, 1.0], [2.0097, -0.00018626524, 0.6987514, 1.0], [2.2609, -0.00024645546, 0.6484681, 1.0], [2.5121, -0.0003150903, 0.5982187, 1.0], [2.7633, -0.0003903196, 0.5479184, 1.0], [3.0144498, -0.00046932563, 0.49767745, 1.0], [3.26565, -0.0005563859, 0.44752148, 1.0], [3.51685, -0.00064487197, 0.397323, 1.0], [3.76805, -0.00073117693, 0.34696326, 1.0], [4.01925, -0.0008170999, 0.29672235, 1.0], [4.27045, -0.0009031756, 0.24646449, 1.0], [4.52165, -0.0009820798, 0.19614716, 1.0], [4.77285, -0.0010612556, 0.14594024, 1.0], [5.0240498, -0.0011366602, 0.0958352, 1.0], [5.27525, -0.0012121152, 0.04556884, 1.0], [5.5264497, -0.0012991133, -0.0047399844, 1.0], [5.77765, -0.0013793214, -0.05493842, 1.0], [6.02885, -0.0014648766, -0.10519629, 1.0], [6.28005, -0.001559259, -0.15536925, 1.0], [6.53125, -0.001651095, -0.20566109, 1.0], [6.7824497, -0.0017487028, -0.255885, 1.0]]}, {"JV metrics"=[[0.0, 0.0], [0.0, 0.0]], "JVData"=[[0.2513, 5.4381195e-05, 1.0503782, 1.0], [0.5025, 2.778111e-05, 1.0002986, 1.0], [0.75369996, 3.9110714e-06, 0.94982845, 1.0], [1.0049, -2.2766604e-05, 0.8997149, 1.0], [1.2560999, -5.2547082e-05, 0.8493892, 1.0], [1.5073, -8.9432746e-05, 0.7991992, 1.0], [1.7585, -0.00013286466, 0.74895835, 1.0], [2.0097, -0.00018626524, 0.6987514, 1.0], [2.2609, -0.00024645546, 0.6484681, 1.0], [2.5121, -0.0003150903, 0.5982187, 1.0], [2.7633, -0.0003903196, 0.5479184, 1.0], [3.0144498, -0.00046932563, 0.49767745, 1.0], [3.26565, -0.0005563859, 0.44752148, 1.0], [3.51685, -0.00064487197, 0.397323, 1.0], [3.76805, -0.00073117693, 0.34696326, 1.0], [4.01925, -0.0008170999, 0.29672235, 1.0], [4.27045, -0.0009031756, 0.24646449, 1.0], [4.52165, -0.0009820798, 0.19614716, 1.0], [4.77285, -0.0010612556, 0.14594024, 1.0], [5.0240498, -0.0011366602, 0.0958352, 1.0], [5.27525, -0.0012121152, 0.04556884, 1.0], [5.5264497, -0.0012991133, -0.0047399844, 1.0], [5.77765, -0.0013793214, -0.05493842, 1.0], [6.02885, -0.0014648766, -0.10519629, 1.0], [6.28005, -0.001559259, -0.15536925, 1.0], [6.53125, -0.001651095, -0.20566109, 1.0], [6.7824497, -0.0017487028, -0.255885, 1.0]]}, {"JV metrics"=[[0.0, 0.0], [0.0, 0.0]], "JVData"=[[0.2513, 5.4381195e-05, 1.0503782, 1.0], [0.5025, 2.778111e-05, 1.0002986, 1.0], [0.75369996, 3.9110714e-06, 0.94982845, 1.0], [1.0049, -2.2766604e-05, 0.8997149, 1.0], [1.2560999, -5.2547082e-05, 0.8493892, 1.0], [1.5073, -8.9432746e-05, 0.7991992, 1.0], [1.7585, -0.00013286466, 0.74895835, 1.0], [2.0097, -0.00018626524, 0.6987514, 1.0], [2.2609, -0.00024645546, 0.6484681, 1.0], [2.5121, -0.0003150903, 0.5982187, 1.0], [2.7633, -0.0003903196, 0.5479184, 1.0], [3.0144498, -0.00046932563, 0.49767745, 1.0], [3.26565, -0.0005563859, 0.44752148, 1.0], [3.51685, -0.00064487197, 0.397323, 1.0], [3.76805, -0.00073117693, 0.34696326, 1.0], [4.01925, -0.0008170999, 0.29672235, 1.0], [4.27045, -0.0009031756, 0.24646449, 1.0], [4.52165, -0.0009820798, 0.19614716, 1.0], [4.77285, -0.0010612556, 0.14594024, 1.0], [5.0240498, -0.0011366602, 0.0958352, 1.0], [5.27525, -0.0012121152, 0.04556884, 1.0], [5.5264497, -0.0012991133, -0.0047399844, 1.0], [5.77765, -0.0013793214, -0.05493842, 1.0], [6.02885, -0.0014648766, -0.10519629, 1.0], [6.28005, -0.001559259, -0.15536925, 1.0], [6.53125, -0.001651095, -0.20566109, 1.0], [6.7824497, -0.0017487028, -0.255885, 1.0]]}, {"JV metrics"=[[0.0, 0.0], [0.0, 0.0]], "JVData"=[[0.2513, 5.4381195e-05, 1.0503782, 1.0], [0.5025, 2.778111e-05, 1.0002986, 1.0], [0.75369996, 3.9110714e-06, 0.94982845, 1.0], [1.0049, -2.2766604e-05, 0.8997149, 1.0], [1.2560999, -5.2547082e-05, 0.8493892, 1.0], [1.5073, -8.9432746e-05, 0.7991992, 1.0], [1.7585, -0.00013286466, 0.74895835, 1.0], [2.0097, -0.00018626524, 0.6987514, 1.0], [2.2609, -0.00024645546, 0.6484681, 1.0], [2.5121, -0.0003150903, 0.5982187, 1.0], [2.7633, -0.0003903196, 0.5479184, 1.0], [3.0144498, -0.00046932563, 0.49767745, 1.0], [3.26565, -0.0005563859, 0.44752148, 1.0], [3.51685, -0.00064487197, 0.397323, 1.0], [3.76805, -0.00073117693, 0.34696326, 1.0], [4.01925, -0.0008170999, 0.29672235, 1.0], [4.27045, -0.0009031756, 0.24646449, 1.0], [4.52165, -0.0009820798, 0.19614716, 1.0], [4.77285, -0.0010612556, 0.14594024, 1.0], [5.0240498, -0.0011366602, 0.0958352, 1.0], [5.27525, -0.0012121152, 0.04556884, 1.0], [5.5264497, -0.0012991133, -0.0047399844, 1.0], [5.77765, -0.0013793214, -0.05493842, 1.0], [6.02885, -0.0014648766, -0.10519629, 1.0], [6.28005, -0.001559259, -0.15536925, 1.0], [6.53125, -0.001651095, -0.20566109, 1.0], [6.7824497, -0.0017487028, -0.255885, 1.0]]}, {"JV metrics"=[[0.0, 0.0], [0.0, 0.0]], "JVData"=[[0.2513, 5.4381195e-05, 1.0503782, 1.0], [0.5025, 2.778111e-05, 1.0002986, 1.0], [0.75369996, 3.9110714e-06, 0.94982845, 1.0], [1.0049, -2.2766604e-05, 0.8997149, 1.0], [1.2560999, -5.2547082e-05, 0.8493892, 1.0], [1.5073, -8.9432746e-05, 0.7991992, 1.0], [1.7585, -0.00013286466, 0.74895835, 1.0], [2.0097, -0.00018626524, 0.6987514, 1.0], [2.2609, -0.00024645546, 0.6484681, 1.0], [2.5121, -0.0003150903, 0.5982187, 1.0], [2.7633, -0.0003903196, 0.5479184, 1.0], [3.0144498, -0.00046932563, 0.49767745, 1.0], [3.26565, -0.0005563859, 0.44752148, 1.0], [3.51685, -0.00064487197, 0.397323, 1.0], [3.76805, -0.00073117693, 0.34696326, 1.0], [4.01925, -0.0008170999, 0.29672235, 1.0], [4.27045, -0.0009031756, 0.24646449, 1.0], [4.52165, -0.0009820798, 0.19614716, 1.0], [4.77285, -0.0010612556, 0.14594024, 1.0], [5.0240498, -0.0011366602, 0.0958352, 1.0], [5.27525, -0.0012121152, 0.04556884, 1.0], [5.5264497, -0.0012991133, -0.0047399844, 1.0], [5.77765, -0.0013793214, -0.05493842, 1.0], [6.02885, -0.0014648766, -0.10519629, 1.0], [6.28005, -0.001559259, -0.15536925, 1.0], [6.53125, -0.001651095, -0.20566109, 1.0], [6.7824497, -0.0017487028, -0.255885, 1.0]]}, {"JV metrics"=[[0.0, 0.0], [0.0, 0.0]], "JVData"=[[0.2513, 5.4381195e-05, 1.0503782, 1.0], [0.5025, 2.778111e-05, 1.0002986, 1.0], [0.75369996, 3.9110714e-06, 0.94982845, 1.0], [1.0049, -2.2766604e-05, 0.8997149, 1.0], [1.2560999, -5.2547082e-05, 0.8493892, 1.0], [1.5073, -8.9432746e-05, 0.7991992, 1.0], [1.7585, -0.00013286466, 0.74895835, 1.0], [2.0097, -0.00018626524, 0.6987514, 1.0], [2.2609, -0.00024645546, 0.6484681, 1.0], [2.5121, -0.0003150903, 0.5982187, 1.0], [2.7633, -0.0003903196, 0.5479184, 1.0], [3.0144498, -0.00046932563, 0.49767745, 1.0], [3.26565, -0.0005563859, 0.44752148, 1.0], [3.51685, -0.00064487197, 0.397323, 1.0], [3.76805, -0.00073117693, 0.34696326, 1.0], [4.01925, -0.0008170999, 0.29672235, 1.0], [4.27045, -0.0009031756, 0.24646449, 1.0], [4.52165, -0.0009820798, 0.19614716, 1.0], [4.77285, -0.0010612556, 0.14594024, 1.0], [5.0240498, -0.0011366602, 0.0958352, 1.0], [5.27525, -0.0012121152, 0.04556884, 1.0], [5.5264497, -0.0012991133, -0.0047399844, 1.0], [5.77765, -0.0013793214, -0.05493842, 1.0], [6.02885, -0.0014648766, -0.10519629, 1.0], [6.28005, -0.001559259, -0.15536925, 1.0], [6.53125, -0.001651095, -0.20566109, 1.0], [6.7824497, -0.0017487028, -0.255885, 1.0]]}, {"JV metrics"=[[0.0, 0.0], [0.0, 0.0]], "JVData"=[[0.2513, 5.4381195e-05, 1.0503782, 1.0], [0.5025, 2.778111e-05, 1.0002986, 1.0], [0.75369996, 3.9110714e-06, 0.94982845, 1.0], [1.0049, -2.2766604e-05, 0.8997149, 1.0], [1.2560999, -5.2547082e-05, 0.8493892, 1.0], [1.5073, -8.9432746e-05, 0.7991992, 1.0], [1.7585, -0.00013286466, 0.74895835, 1.0], [2.0097, -0.00018626524, 0.6987514, 1.0], [2.2609, -0.00024645546, 0.6484681, 1.0], [2.5121, -0.0003150903, 0.5982187, 1.0], [2.7633, -0.0003903196, 0.5479184, 1.0], [3.0144498, -0.00046932563, 0.49767745, 1.0], [3.26565, -0.0005563859, 0.44752148, 1.0], [3.51685, -0.00064487197, 0.397323, 1.0], [3.76805, -0.00073117693, 0.34696326, 1.0], [4.01925, -0.0008170999, 0.29672235, 1.0], [4.27045, -0.0009031756, 0.24646449, 1.0], [4.52165, -0.0009820798, 0.19614716, 1.0], [4.77285, -0.0010612556, 0.14594024, 1.0], [5.0240498, -0.0011366602, 0.0958352, 1.0], [5.27525, -0.0012121152, 0.04556884, 1.0], [5.5264497, -0.0012991133, -0.0047399844, 1.0], [5.77765, -0.0013793214, -0.05493842, 1.0], [6.02885, -0.0014648766, -0.10519629, 1.0], [6.28005, -0.001559259, -0.15536925, 1.0], [6.53125, -0.001651095, -0.20566109, 1.0], [6.7824497, -0.0017487028, -0.255885, 1.0]]}] {"JVData" format="%.2f"}
  out "ResetJVLiveView":bool[](array[boolean])
  out "ResetAgingLiveView":bool[](array[boolean])
  out "ExchangeJVData":sgl[][](array[numeric])=[[0.16746, 0.64255065, -1.0903614e-07, 0.6447156, 1.0], [0.33473998, 0.59235585, -2.696132e-07, 0.5940376, 1.0], [0.50207996, 0.542161, -5.542517e-07, 0.5406553, 1.0], [0.66936, 0.49196616, -6.6120117e-07, 0.48496604, 1.0], [0.83669996, 0.44177133, -1.0984718e-06, 0.43833676, 1.0], [1.00404, 0.3915765, -1.5501042e-06, 0.39644372, 1.0], [1.17132, 0.34138167, -1.6720268e-06, 0.35270205, 1.0], [1.33866, 0.29118684, -1.9528457e-06, 0.30110732, 1.0], [1.50594, 0.240992, -2.0510863e-06, 0.2324926, 1.0], [1.67328, 0.19079718, -2.4617725e-06, 0.19632894, 1.0], [1.8406199, 0.14060235, -2.7752872e-06, 0.14613982, 1.0], [2.0079, 0.09040751, -2.9995756e-06, 0.08873936, 1.0], [2.17524, 0.040212683, -3.3456338e-06, 0.043943465, 1.0], [2.34252, -0.009982145, -3.6904694e-06, -0.010401342, 1.0], [2.50986, -0.060176972, -4.1104754e-06, -0.04554136, 1.0], [2.6771998, -0.1103718, -4.3372083e-06, -0.10945036, 1.0], [2.84448, -0.16056663, -4.7158096e-06, -0.15922697, 1.0], [2.97588, -0.19998342, -4.8545385e-06, -0.20972164, 1.0], [3.14322, -0.14978859, -4.0877107e-06, -0.14604181, 1.0], [3.3105, -0.099593766, -3.2392952e-06, -0.097304136, 1.0], [3.47784, -0.04939894, -2.818831e-06, -0.048933137, 1.0], [3.64512, 0.00079588447, -2.3891996e-06, 0.00041567357, 1.0], [3.81246, 0.050990716, -1.9065516e-06, 0.047228295, 1.0], [3.9798, 0.101185545, -1.690972e-06, 0.0906797, 1.0], [4.14708, 0.15138038, -1.4533914e-06, 0.15038718, 1.0], [4.3144197, 0.2015752, -1.3138987e-06, 0.20405975, 1.0], [4.4817, 0.25177005, -1.2779942e-06, 0.25212517, 1.0], [4.6490397, 0.30196488, -8.4439034e-07, 0.29427794, 1.0], [4.81638, 0.3521597, -8.6409966e-07, 0.3574383, 1.0], [4.9836597, 0.4023545, -7.2567644e-07, 0.4079635, 1.0], [5.151, 0.45254934, -4.8198433e-07, 0.45813736, 1.0], [5.3182797, 0.5027442, -2.428758e-07, 0.5003818, 1.0], [5.48562, 0.552939, -8.611839e-08, 0.55277103, 1.0], [5.65296, 0.60313386, 4.4160106e-07, 0.6010656, 1.0], [5.82024, 0.65332866, 6.22193e-07, 0.64738935, 1.0], [0.16746, 0.08287942, 1.7164284e-08, 0.0833232, 1.0], [0.33473998, 0.032685004, -4.2421867e-08, 0.032125723, 1.0], [0.50207996, -0.017509406, -9.085472e-08, -0.00891171, 1.0], [0.66936, -0.06770381, -7.8173564e-08, -0.06629689, 1.0], [0.83669996, -0.117898226, -8.184041e-08, -0.11847218, 1.0], [1.0039799, -0.16809264, -1.2905097e-07, -0.16681261, 1.0], [1.11078, -0.20011851, -7.970142e-08, -0.2017693, 1.0], [1.2781199, -0.1499241, -1.4646847e-07, -0.1451022, 1.0], [1.4454, -0.099729694, -5.5408602e-08, -0.09281997, 1.0], [1.6127399, -0.04953529, 4.5429513e-08, -0.05254645, 1.0], [1.78002, 0.0006591209, -3.722718e-08, 0.0022414266, 1.0], [1.9473599, 0.05085353, -6.3353426e-08, 0.055532034, 1.0], [2.11464, 0.10104795, 1.00432125e-07, 0.08567607, 1.0], [0.50826, 0.35650185, 4.8261914e-08, 0.35597858, 1.0], [1.01634, 0.34633976, 3.5016622e-08, 0.3490164, 1.0], [1.5244199, 0.33617768, -3.1327332e-08, 0.33783153, 1.0], [2.0325599, 0.3260156, 7.295432e-08, 0.32564417, 1.0], [2.5406399, 0.3158535, 4.102225e-08, 0.31237674, 1.0], [3.04878, 0.30569142, 6.046237e-09, 0.30614087, 1.0], [3.55686, 0.2955293, 5.7334987e-08, 0.2953826, 1.0], [4.06494, 0.28536722, -2.3817359e-08, 0.28514028, 1.0], [4.57308, 0.27520514, 3.8671715e-08, 0.27568892, 1.0], [5.08116, 0.26504305, -7.669157e-09, 0.2651622, 1.0], [5.5892997, 0.25488096, 8.6200735e-09, 0.25504795, 1.0], [6.0973797, 0.24471886, 1.6306336e-08, 0.24763331, 1.0], [6.6054597, 0.23455678, -2.1983938e-08, 0.23487948, 1.0], [7.1136, 0.22439468, 7.3918045e-08, 0.22360058, 1.0], [7.62168, 0.2142326, 5.9757177e-09, 0.21352632, 1.0], [8.12982, 0.20407051, 1.1664023e-08, 0.20324053, 1.0], [8.637899, 0.19390842, 5.342234e-10, 0.195364, 1.0], [9.14604, 0.18374632, -5.239991e-08, 0.18436247, 1.0], [9.6541195, 0.17358424, 3.901254e-08, 0.1724654, 1.0], [10.1622, 0.16342215, -3.5805105e-08, 0.1645395, 1.0], [10.67034, 0.15326007, -7.046263e-09, 0.15484014, 1.0], [11.17842, 0.14309797, 7.597592e-09, 0.14352247, 1.0], [11.68656, 0.13293588, -8.396764e-08, 0.13540854, 1.0], [12.19464, 0.12277379, 2.2464747e-08, 0.12296967, 1.0], [0.50826, 0.24064891, 5.054193e-08, 0.24092051, 1.0], [1.01634, 0.23048687, -3.110403e-08, 0.2318652, 1.0], [1.5244199, 0.22032481, -4.6475607e-10, 0.22103643, 1.0], [2.0325599, 0.21016277, 2.0560812e-08, 0.20964117, 1.0], [2.5406399, 0.20000072, -6.820728e-08, 0.20214543, 1.0], [3.04872, 0.18983868, 5.567786e-08, 0.19041994, 1.0], [3.55686, 0.17967662, -2.9728964e-08, 0.18028222, 1.0], [4.06494, 0.16951458, 1.7305315e-08, 0.1693994, 1.0], [4.57308, 0.15935254, 1.5460142e-08, 0.15982696, 1.0], [5.08116, 0.14919049, -2.7589973e-08, 0.14702262, 1.0], [5.58924, 0.13902844, 2.1160199e-08, 0.14099239, 1.0], [0.50064, 0.8999383, 4.595726e-06, 0.90037847, 1.0], [1.00104, 0.7998477, 2.1555804e-06, 0.8003987, 1.0], [1.5015, 0.6997571, 6.2240116e-07, 0.700059, 1.0], [2.00196, 0.5996665, 8.959112e-08, 0.6002757, 1.0], [2.50242, 0.49957585, -4.069255e-08, 0.4998595, 1.0], [3.0028799, 0.39948523, -2.5073948e-07, 0.39971617, 1.0], [3.50334, 0.2993946, -4.2194137e-07, 0.299911, 1.0], [4.0038, 0.199304, -6.0874675e-07, 0.19984399, 1.0], [4.50426, 0.099213384, -7.7514756e-07, 0.09990792, 1.0], [5.0047197, -0.000877235, -8.6516764e-07, -0.00039909285, 1.0], [5.50512, -0.10096785, -9.697001e-07, -0.100826114, 1.0], [6.00096, -0.20013455, -1.0205479e-06, -0.199933, 1.0], [6.5014796, -0.10004393, -8.0013496e-07, -0.10054245, 1.0], [7.0018797, 4.6678295e-05, -6.5861246e-07, -0.0001699818, 1.0], [7.50234, 0.10013729, -5.4753303e-07, 0.10008249, 1.0], [8.0028, 0.20022792, -4.41473e-07, 0.19999674, 1.0], [8.50326, 0.30031854, -2.7616335e-07, 0.30009645, 1.0], [9.003719, 0.40040913, -1.8777995e-07, 0.400098, 1.0], [9.50418, 0.5004998, 3.1105312e-08, 0.5005905, 1.0], [10.00464, 0.6005904, 3.775464e-07, 0.59995925, 1.0], [10.505099, 0.700681, 9.298881e-07, 0.7005827, 1.0], [11.00556, 0.8007716, 1.9000322e-06, 0.79998416, 1.0], [11.5059595, 0.9008622, 4.2082575e-06, 0.9002584, 1.0], [0.50064, 1.0999515, 4.125463e-05, 1.1008824, 1.0], [1.00104, 0.9998607, 2.328144e-05, 1.0004772, 1.0], [1.5015, 0.8997699, 9.654282e-06, 0.9002902, 1.0], [2.00196, 0.79967904, 2.936846e-06, 0.80020136, 1.0], [2.50242, 0.69958824, 7.5246663e-07, 0.6998943, 1.0], [3.0028799, 0.59949744, 6.7986285e-08, 0.59989285, 1.0], [3.50334, 0.4994066, -2.6776146e-07, 0.49989128, 1.0], [4.0038, 0.39931577, -4.1637648e-07, 0.3998461, 1.0], [4.50426, 0.29922494, -5.8866954e-07, 0.2995609, 1.0], [5.0047197, 0.19913413, -6.6068554e-07, 0.19967936, 1.0], [5.50518, 0.099043295, -7.7307436e-07, 0.09944872, 1.0], [6.00558, -0.0010475283, -8.8338993e-07, -0.00043280495, 1.0], [6.5060396, -0.101138346, -9.85631e-07, -0.100914374, 1.0], [7.00032, -0.19999728, -1.0913636e-06, -0.1998249, 1.0], [7.5008397, -0.09990646, -8.3232396e-07, -0.10005248, 1.0], [8.00124, 0.00018435865, -6.669051e-07, 3.5971088e-06, 1.0], [8.501699, 0.10027518, -5.2658294e-07, 0.100179695, 1.0], [9.00216, 0.200366, -3.772041e-07, 0.20012668, 1.0], [9.50262, 0.30045682, -2.0960302e-07, 0.30028096, 1.0], [10.003079, 0.40054765, -1.7341883e-08, 0.40050068, 1.0], [10.50354, 0.5006385, 1.4207558e-07, 0.5003604, 1.0], [11.004, 0.6007293, 3.7089038e-07, 0.6004274, 1.0], [11.504459, 0.70082015, 8.100795e-07, 0.700669, 1.0], [12.00492, 0.80091095, 2.5522145e-06, 0.8007905, 1.0], [12.50538, 0.90100175, 8.807359e-06, 0.90092295, 1.0], [13.005779, 1.0010927, 2.1100788e-05, 1.0009027, 1.0], [13.50624, 1.1011834, 3.786856e-05, 1.1013625, 1.0]]
  in  "Tab Control":T3(tab)=enum."Advanced Settings"
  out "IntBar A 2":dbl(slide) scale=0.001..1.0
  out "IntBar A 1":dbl(slide) scale=0.001..1.0
  out "Tank 16":dbl(slide) max=-0.4994445741176605 scale=0.0..12.796661376953125 scale format="%#_3g"
  out "Tank 15":dbl(slide) max=-0.4994445741176605 scale=0.0..15.633349418640137 scale format="%#_3g"
  out "Tank 14":dbl(slide) max=-0.4994445741176605 scale=0.0..10.464171409606934 scale format="%#_3g"
  out "Tank 13":dbl(slide) max=-0.4994445741176605 scale=0.0..0.0034484637435525656 scale format="%#_3g"
  out "Tank 12":dbl(slide) max=-0.4994445741176605 scale=0.0..13.11457347869873 scale format="%#_3g"
  out "Tank 11":dbl(slide) max=-0.4994445741176605 scale=0.0..11.280762672424316 scale format="%#_3g"
  out "Tank 10":dbl(slide) max=-0.4994445741176605 scale=0.0..0.6310564875602722 scale format="%#_3g"
  out "Tank 9":dbl(slide)=0.0011021399404853582 max=-0.4994445741176605 scale=0.0..15.408804893493652 scale format="%#_3g"
  out "IntA":dbl caption="suns" format="%#_3g"
  in  "stop":bool
  in  "Activate Magic Control":bool
  out "Tab Control Buttons":enum32{"Page 1"}(tab)
  in  "JVMPPst":bool
  in  "JVstandard":bool
  in  "Agingstandard":bool
  in  "Save As Button":bool
  in  "Open Button":bool
  in  "Monitor OC of non active channels":bool
  out "Tank 8":dbl(slide) max=-0.4994445741176605 scale=0.0..0.0014319480396807194 scale format="%#_3g"
  out "Tank 7":dbl(slide) max=-0.4994445741176605 scale=0.0..26.805625915527344 scale format="%#_3g"
  out "Tank 6":dbl(slide) max=-0.4994445741176605 scale=0.0..1.215698480606079 scale format="%#_3g"
  out "Tank 5":dbl(slide) max=-0.4994445741176605 scale=0.0..0.001173172378912568 scale format="%#_3g"
  out "Tank 4":dbl(slide) max=-0.4994445741176605 scale=0.0..19.24797248840332 scale format="%#_3g"
  out "Tank 3":dbl(slide) max=-0.4994445741176605 scale=0.0..1.1456093788146973 scale format="%#_3g"
  out "Tank 2":dbl(slide) max=-0.4994445741176605 scale=0.0..20.232755661010742 scale format="%#_3g"
  out "Tank 1":dbl(slide)=0.0011021399404853582 max=-0.4994445741176605 scale=0.0..19.442453384399414 scale format="%#_3g"
  in  "RestoreLastAutoSave":bool
  out "Active 8":bool
  out "Active 7":bool
  out "Active 6":bool
  out "Active 5":bool
  out "Active 4":bool
  out "Active 3":bool
  out "Active 2":bool
  out "Active 1":bool
  out "T78":dbl format="%#_3g"
  out "T56":dbl format="%#_3g"
  out "T34":dbl format="%#_3g"
  out "T12":dbl format="%#_3g"
  out "Voc 8":dbl=-0.7008459568023682 format="%#_4g"
  out "Voc 7":dbl=-0.948243260383606 format="%#_4g"
  out "Voc 6":dbl=-0.5114282369613647 format="%#_4g"
  out "Voc 5":dbl=-0.7734385132789612 format="%#_4g"
  out "Voc 4":dbl=-0.6023858189582825 format="%#_4g"
  out "Voc 3":dbl=-0.5110825896263123 format="%#_4g"
  out "Voc 2":dbl=0.19164180755615234 format="%#_4g"
  out "Voc 1":dbl=0.2513234615325928 format="%#_4g"
  in  "StopCh":bool
  in  "PauseCh":bool
  in  "StartCh":bool
  in  "ConfigTable":T4(array[cluster])=[{"name"="Device1", "Channel"=0, "StartCh"=FALSE, "PauseCh"=FALSE, "StopCh"=FALSE, "ActiveArea cm2"=0.16, "AgingMode"=enum."MPP", "JVParameters"={"Hyst"=TRUE, "Start"=1.2, "End"=0.0, "rate"=100.0, "record dE"=10.0, "equ t1"=3.0, "equ t2"=0.0, "vsInitEnd 2"=FALSE, "vsInitSt 3"=FALSE}, "AgingParams"={"Time"=15.0, "StepV"=0.01, "timetocheck"=1.0, "average over"=10.0}, "start time"=timestamp(3545987186.527957 s since 1904-01-01), "AgingFile"=path "C:/EC-Lab Development Package/Examples/Labview/V12/DefaultAging/Ch1_Device1_160513_14h_26m26s_aging.txt", "JVFile"=path "C:/EC-Lab Development Package/Examples/Labview/V12/DefaultAging/Ch1_Device1_160513_14h_26m26s_JVs.txt", "JVMetricsFile"=path "C:/EC-Lab Development Package/Examples/Labview/V12/DefaultAging/Ch1_Device1_160513_14h_26m26s_JVmetrics.txt", "Status"=0.0, "ColorInd"=FALSE, "RunCont"=TRUE, "StatusStr"="stopped", "CopyToAll"=FALSE}, {"name"="Device2", "Channel"=1, "StartCh"=FALSE, "PauseCh"=FALSE, "StopCh"=FALSE, "ActiveArea cm2"=0.16, "AgingMode"=enum."MPP", "JVParameters"={"Hyst"=TRUE, "Start"=1.2, "End"=0.0, "rate"=100.0, "record dE"=10.0, "equ t1"=3.0, "equ t2"=0.0, "vsInitEnd 2"=FALSE, "vsInitSt 3"=FALSE}, "AgingParams"={"Time"=15.0, "StepV"=0.01, "timetocheck"=1.0, "average over"=10.0}, "start time"=timestamp(3545987186.527957 s since 1904-01-01), "AgingFile"=path "C:/EC-Lab Development Package/Examples/Labview/V12/DefaultAging/Ch1_Device1_160513_14h_26m26s_aging.txt", "JVFile"=path "C:/EC-Lab Development Package/Examples/Labview/V12/DefaultAging/Ch1_Device1_160513_14h_26m26s_JVs.txt", "JVMetricsFile"=path "C:/EC-Lab Development Package/Examples/Labview/V12/DefaultAging/Ch1_Device1_160513_14h_26m26s_JVmetrics.txt", "Status"=0.0, "ColorInd"=FALSE, "RunCont"=TRUE, "StatusStr"="stopped", "CopyToAll"=FALSE}, {"name"="Device3", "Channel"=2, "StartCh"=FALSE, "PauseCh"=FALSE, "StopCh"=FALSE, "ActiveArea cm2"=0.16, "AgingMode"=enum."MPP", "JVParameters"={"Hyst"=TRUE, "Start"=1.2, "End"=0.0, "rate"=100.0, "record dE"=10.0, "equ t1"=3.0, "equ t2"=0.0, "vsInitEnd 2"=FALSE, "vsInitSt 3"=FALSE}, "AgingParams"={"Time"=15.0, "StepV"=0.01, "timetocheck"=1.0, "average over"=10.0}, "start time"=timestamp(3545987186.527957 s since 1904-01-01), "AgingFile"=path "C:/EC-Lab Development Package/Examples/Labview/V12/DefaultAging/Ch1_Device1_160513_14h_26m26s_aging.txt", "JVFile"=path "C:/EC-Lab Development Package/Examples/Labview/V12/DefaultAging/Ch1_Device1_160513_14h_26m26s_JVs.txt", "JVMetricsFile"=path "C:/EC-Lab Development Package/Examples/Labview/V12/DefaultAging/Ch1_Device1_160513_14h_26m26s_JVmetrics.txt", "Status"=0.0, "ColorInd"=FALSE, "RunCont"=TRUE, "StatusStr"="stopped", "CopyToAll"=FALSE}, {"name"="Device4", "Channel"=3, "StartCh"=FALSE, "PauseCh"=FALSE, "StopCh"=FALSE, "ActiveArea cm2"=0.16, "AgingMode"=enum."MPP", "JVParameters"={"Hyst"=TRUE, "Start"=1.2, "End"=0.0, "rate"=100.0, "record dE"=10.0, "equ t1"=3.0, "equ t2"=0.0, "vsInitEnd 2"=FALSE, "vsInitSt 3"=FALSE}, "AgingParams"={"Time"=15.0, "StepV"=0.01, "timetocheck"=1.0, "average over"=10.0}, "start time"=timestamp(3545987186.527957 s since 1904-01-01), "AgingFile"=path "C:/EC-Lab Development Package/Examples/Labview/V12/DefaultAging/Ch1_Device1_160513_14h_26m26s_aging.txt", "JVFile"=path "C:/EC-Lab Development Package/Examples/Labview/V12/DefaultAging/Ch1_Device1_160513_14h_26m26s_JVs.txt", "JVMetricsFile"=path "C:/EC-Lab Development Package/Examples/Labview/V12/DefaultAging/Ch1_Device1_160513_14h_26m26s_JVmetrics.txt", "Status"=0.0, "ColorInd"=FALSE, "RunCont"=TRUE, "StatusStr"="stopped", "CopyToAll"=FALSE}, {"name"="Device5", "Channel"=4, "StartCh"=FALSE, "PauseCh"=FALSE, "StopCh"=FALSE, "ActiveArea cm2"=0.16, "AgingMode"=enum."MPP", "JVParameters"={"Hyst"=TRUE, "Start"=1.2, "End"=0.0, "rate"=100.0, "record dE"=10.0, "equ t1"=3.0, "equ t2"=0.0, "vsInitEnd 2"=FALSE, "vsInitSt 3"=FALSE}, "AgingParams"={"Time"=15.0, "StepV"=0.01, "timetocheck"=1.0, "average over"=10.0}, "start time"=timestamp(3545987186.527957 s since 1904-01-01), "AgingFile"=path "C:/EC-Lab Development Package/Examples/Labview/V12/DefaultAging/Ch1_Device1_160513_14h_26m26s_aging.txt", "JVFile"=path "C:/EC-Lab Development Package/Examples/Labview/V12/DefaultAging/Ch1_Device1_160513_14h_26m26s_JVs.txt", "JVMetricsFile"=path "C:/EC-Lab Development Package/Examples/Labview/V12/DefaultAging/Ch1_Device1_160513_14h_26m26s_JVmetrics.txt", "Status"=0.0, "ColorInd"=FALSE, "RunCont"=TRUE, "StatusStr"="stopped", "CopyToAll"=FALSE}, {"name"="Device6", "Channel"=5, "StartCh"=FALSE, "PauseCh"=FALSE, "StopCh"=FALSE, "ActiveArea cm2"=0.16, "AgingMode"=enum."MPP", "JVParameters"={"Hyst"=TRUE, "Start"=1.2, "End"=0.0, "rate"=100.0, "record dE"=10.0, "equ t1"=3.0, "equ t2"=0.0, "vsInitEnd 2"=FALSE, "vsInitSt 3"=FALSE}, "AgingParams"={"Time"=15.0, "StepV"=0.01, "timetocheck"=1.0, "average over"=10.0}, "start time"=timestamp(3545987186.527957 s since 1904-01-01), "AgingFile"=path "C:/EC-Lab Development Package/Examples/Labview/V12/DefaultAging/Ch1_Device1_160513_14h_26m26s_aging.txt", "JVFile"=path "C:/EC-Lab Development Package/Examples/Labview/V12/DefaultAging/Ch1_Device1_160513_14h_26m26s_JVs.txt", "JVMetricsFile"=path "C:/EC-Lab Development Package/Examples/Labview/V12/DefaultAging/Ch1_Device1_160513_14h_26m26s_JVmetrics.txt", "Status"=0.0, "ColorInd"=FALSE, "RunCont"=TRUE, "StatusStr"="stopped", "CopyToAll"=FALSE}, {"name"="Device7", "Channel"=6, "StartCh"=FALSE, "PauseCh"=FALSE, "StopCh"=FALSE, "ActiveArea cm2"=0.16, "AgingMode"=enum."MPP", "JVParameters"={"Hyst"=TRUE, "Start"=1.2, "End"=0.0, "rate"=100.0, "record dE"=10.0, "equ t1"=3.0, "equ t2"=0.0, "vsInitEnd 2"=FALSE, "vsInitSt 3"=FALSE}, "AgingParams"={"Time"=15.0, "StepV"=0.01, "timetocheck"=1.0, "average over"=10.0}, "start time"=timestamp(3545987186.527957 s since 1904-01-01), "AgingFile"=path "C:/EC-Lab Development Package/Examples/Labview/V12/DefaultAging/Ch1_Device1_160513_14h_26m26s_aging.txt", "JVFile"=path "C:/EC-Lab Development Package/Examples/Labview/V12/DefaultAging/Ch1_Device1_160513_14h_26m26s_JVs.txt", "JVMetricsFile"=path "C:/EC-Lab Development Package/Examples/Labview/V12/DefaultAging/Ch1_Device1_160513_14h_26m26s_JVmetrics.txt", "Status"=0.0, "ColorInd"=FALSE, "RunCont"=TRUE, "StatusStr"="stopped", "CopyToAll"=FALSE}, {"name"="Device8", "Channel"=7, "StartCh"=FALSE, "PauseCh"=FALSE, "StopCh"=FALSE, "ActiveArea cm2"=0.16, "AgingMode"=enum."MPP", "JVParameters"={"Hyst"=TRUE, "Start"=1.2, "End"=0.0, "rate"=100.0, "record dE"=10.0, "equ t1"=3.0, "equ t2"=0.0, "vsInitEnd 2"=FALSE, "vsInitSt 3"=FALSE}, "AgingParams"={"Time"=15.0, "StepV"=0.01, "timetocheck"=1.0, "average over"=10.0}, "start time"=timestamp(3545987186.527957 s since 1904-01-01), "AgingFile"=path "C:/EC-Lab Development Package/Examples/Labview/V12/DefaultAging/Ch1_Device1_160513_14h_26m26s_aging.txt", "JVFile"=path "C:/EC-Lab Development Package/Examples/Labview/V12/DefaultAging/Ch1_Device1_160513_14h_26m26s_JVs.txt", "JVMetricsFile"=path "C:/EC-Lab Development Package/Examples/Labview/V12/DefaultAging/Ch1_Device1_160513_14h_26m26s_JVmetrics.txt", "Status"=0.0, "ColorInd"=FALSE, "RunCont"=TRUE, "StatusStr"="stopped", "CopyToAll"=FALSE}, {"name"="Device9", "Channel"=8, "StartCh"=FALSE, "PauseCh"=FALSE, "StopCh"=FALSE, "ActiveArea cm2"=0.16, "AgingMode"=enum."MPP", "JVParameters"={"Hyst"=TRUE, "Start"=1.2, "End"=0.0, "rate"=100.0, "record dE"=10.0, "equ t1"=3.0, "equ t2"=0.0, "vsInitEnd 2"=FALSE, "vsInitSt 3"=FALSE}, "AgingParams"={"Time"=15.0, "StepV"=0.01, "timetocheck"=1.0, "average over"=10.0}, "start time"=timestamp(3545987186.527957 s since 1904-01-01), "AgingFile"=path "C:/EC-Lab Development Package/Examples/Labview/V12/DefaultAging/Ch1_Device1_160513_14h_26m26s_aging.txt", "JVFile"=path "C:/EC-Lab Development Package/Examples/Labview/V12/DefaultAging/Ch1_Device1_160513_14h_26m26s_JVs.txt", "JVMetricsFile"=path "C:/EC-Lab Development Package/Examples/Labview/V12/DefaultAging/Ch1_Device1_160513_14h_26m26s_JVmetrics.txt", "Status"=0.0, "ColorInd"=FALSE, "RunCont"=TRUE, "StatusStr"="stopped", "CopyToAll"=FALSE}, {"name"="Device10", "Channel"=9, "StartCh"=FALSE, "PauseCh"=FALSE, "StopCh"=FALSE, "ActiveArea cm2"=0.16, "AgingMode"=enum."MPP", "JVParameters"={"Hyst"=TRUE, "Start"=1.2, "End"=0.0, "rate"=100.0, "record dE"=10.0, "equ t1"=3.0, "equ t2"=0.0, "vsInitEnd 2"=FALSE, "vsInitSt 3"=FALSE}, "AgingParams"={"Time"=15.0, "StepV"=0.01, "timetocheck"=1.0, "average over"=10.0}, "start time"=timestamp(3545987186.527957 s since 1904-01-01), "AgingFile"=path "C:/EC-Lab Development Package/Examples/Labview/V12/DefaultAging/Ch1_Device1_160513_14h_26m26s_aging.txt", "JVFile"=path "C:/EC-Lab Development Package/Examples/Labview/V12/DefaultAging/Ch1_Device1_160513_14h_26m26s_JVs.txt", "JVMetricsFile"=path "C:/EC-Lab Development Package/Examples/Labview/V12/DefaultAging/Ch1_Device1_160513_14h_26m26s_JVmetrics.txt", "Status"=0.0, "ColorInd"=FALSE, "RunCont"=TRUE, "StatusStr"="stopped", "CopyToAll"=FALSE}, {"name"="Device11", "Channel"=10, "StartCh"=FALSE, "PauseCh"=FALSE, "StopCh"=FALSE, "ActiveArea cm2"=0.16, "AgingMode"=enum."MPP", "JVParameters"={"Hyst"=TRUE, "Start"=1.2, "End"=0.0, "rate"=100.0, "record dE"=10.0, "equ t1"=3.0, "equ t2"=0.0, "vsInitEnd 2"=FALSE, "vsInitSt 3"=FALSE}, "AgingParams"={"Time"=15.0, "StepV"=0.01, "timetocheck"=1.0, "average over"=10.0}, "start time"=timestamp(3545987186.527957 s since 1904-01-01), "AgingFile"=path "C:/EC-Lab Development Package/Examples/Labview/V12/DefaultAging/Ch1_Device1_160513_14h_26m26s_aging.txt", "JVFile"=path "C:/EC-Lab Development Package/Examples/Labview/V12/DefaultAging/Ch1_Device1_160513_14h_26m26s_JVs.txt", "JVMetricsFile"=path "C:/EC-Lab Development Package/Examples/Labview/V12/DefaultAging/Ch1_Device1_160513_14h_26m26s_JVmetrics.txt", "Status"=0.0, "ColorInd"=FALSE, "RunCont"=TRUE, "StatusStr"="stopped", "CopyToAll"=FALSE}, {"name"="Device12", "Channel"=11, "StartCh"=FALSE, "PauseCh"=FALSE, "StopCh"=FALSE, "ActiveArea cm2"=0.16, "AgingMode"=enum."MPP", "JVParameters"={"Hyst"=TRUE, "Start"=1.2, "End"=0.0, "rate"=100.0, "record dE"=10.0, "equ t1"=3.0, "equ t2"=0.0, "vsInitEnd 2"=FALSE, "vsInitSt 3"=FALSE}, "AgingParams"={"Time"=15.0, "StepV"=0.01, "timetocheck"=1.0, "average over"=10.0}, "start time"=timestamp(3545987186.527957 s since 1904-01-01), "AgingFile"=path "C:/EC-Lab Development Package/Examples/Labview/V12/DefaultAging/Ch1_Device1_160513_14h_26m26s_aging.txt", "JVFile"=path "C:/EC-Lab Development Package/Examples/Labview/V12/DefaultAging/Ch1_Device1_160513_14h_26m26s_JVs.txt", "JVMetricsFile"=path "C:/EC-Lab Development Package/Examples/Labview/V12/DefaultAging/Ch1_Device1_160513_14h_26m26s_JVmetrics.txt", "Status"=0.0, "ColorInd"=FALSE, "RunCont"=TRUE, "StatusStr"="stopped", "CopyToAll"=FALSE}, {"name"="Device13", "Channel"=12, "StartCh"=FALSE, "PauseCh"=FALSE, "StopCh"=FALSE, "ActiveArea cm2"=0.16, "AgingMode"=enum."MPP", "JVParameters"={"Hyst"=TRUE, "Start"=1.2, "End"=0.0, "rate"=100.0, "record dE"=10.0, "equ t1"=3.0, "equ t2"=0.0, "vsInitEnd 2"=FALSE, "vsInitSt 3"=FALSE}, "AgingParams"={"Time"=15.0, "StepV"=0.01, "timetocheck"=1.0, "average over"=10.0}, "start time"=timestamp(3545987186.527957 s since 1904-01-01), "AgingFile"=path "C:/EC-Lab Development Package/Examples/Labview/V12/DefaultAging/Ch1_Device1_160513_14h_26m26s_aging.txt", "JVFile"=path "C:/EC-Lab Development Package/Examples/Labview/V12/DefaultAging/Ch1_Device1_160513_14h_26m26s_JVs.txt", "JVMetricsFile"=path "C:/EC-Lab Development Package/Examples/Labview/V12/DefaultAging/Ch1_Device1_160513_14h_26m26s_JVmetrics.txt", "Status"=0.0, "ColorInd"=FALSE, "RunCont"=TRUE, "StatusStr"="stopped", "CopyToAll"=FALSE}, {"name"="Device14", "Channel"=13, "StartCh"=FALSE, "PauseCh"=FALSE, "StopCh"=FALSE, "ActiveArea cm2"=0.16, "AgingMode"=enum."MPP", "JVParameters"={"Hyst"=TRUE, "Start"=1.2, "End"=0.0, "rate"=100.0, "record dE"=10.0, "equ t1"=3.0, "equ t2"=0.0, "vsInitEnd 2"=FALSE, "vsInitSt 3"=FALSE}, "AgingParams"={"Time"=15.0, "StepV"=0.01, "timetocheck"=1.0, "average over"=10.0}, "start time"=timestamp(3545987186.527957 s since 1904-01-01), "AgingFile"=path "C:/EC-Lab Development Package/Examples/Labview/V12/DefaultAging/Ch1_Device1_160513_14h_26m26s_aging.txt", "JVFile"=path "C:/EC-Lab Development Package/Examples/Labview/V12/DefaultAging/Ch1_Device1_160513_14h_26m26s_JVs.txt", "JVMetricsFile"=path "C:/EC-Lab Development Package/Examples/Labview/V12/DefaultAging/Ch1_Device1_160513_14h_26m26s_JVmetrics.txt", "Status"=0.0, "ColorInd"=FALSE, "RunCont"=TRUE, "StatusStr"="stopped", "CopyToAll"=FALSE}, {"name"="Device15", "Channel"=14, "StartCh"=FALSE, "PauseCh"=FALSE, "StopCh"=FALSE, "ActiveArea cm2"=0.16, "AgingMode"=enum."MPP", "JVParameters"={"Hyst"=TRUE, "Start"=1.2, "End"=0.0, "rate"=100.0, "record dE"=10.0, "equ t1"=3.0, "equ t2"=0.0, "vsInitEnd 2"=FALSE, "vsInitSt 3"=FALSE}, "AgingParams"={"Time"=15.0, "StepV"=0.01, "timetocheck"=1.0, "average over"=10.0}, "start time"=timestamp(3545987186.527957 s since 1904-01-01), "AgingFile"=path "C:/EC-Lab Development Package/Examples/Labview/V12/DefaultAging/Ch1_Device1_160513_14h_26m26s_aging.txt", "JVFile"=path "C:/EC-Lab Development Package/Examples/Labview/V12/DefaultAging/Ch1_Device1_160513_14h_26m26s_JVs.txt", "JVMetricsFile"=path "C:/EC-Lab Development Package/Examples/Labview/V12/DefaultAging/Ch1_Device1_160513_14h_26m26s_JVmetrics.txt", "Status"=0.0, "ColorInd"=FALSE, "RunCont"=TRUE, "StatusStr"="stopped", "CopyToAll"=FALSE}, {"name"="Device16", "Channel"=15, "StartCh"=FALSE, "PauseCh"=FALSE, "StopCh"=FALSE, "ActiveArea cm2"=0.16, "AgingMode"=enum."MPP", "JVParameters"={"Hyst"=TRUE, "Start"=1.2, "End"=0.0, "rate"=100.0, "record dE"=10.0, "equ t1"=3.0, "equ t2"=0.0, "vsInitEnd 2"=FALSE, "vsInitSt 3"=FALSE}, "AgingParams"={"Time"=15.0, "StepV"=0.01, "timetocheck"=1.0, "average over"=10.0}, "start time"=timestamp(3545987186.527957 s since 1904-01-01), "AgingFile"=path "C:/EC-Lab Development Package/Examples/Labview/V12/DefaultAging/Ch1_Device1_160513_14h_26m26s_aging.txt", "JVFile"=path "C:/EC-Lab Development Package/Examples/Labview/V12/DefaultAging/Ch1_Device1_160513_14h_26m26s_JVs.txt", "JVMetricsFile"=path "C:/EC-Lab Development Package/Examples/Labview/V12/DefaultAging/Ch1_Device1_160513_14h_26m26s_JVmetrics.txt", "Status"=0.0, "ColorInd"=FALSE, "RunCont"=TRUE, "StatusStr"="stopped", "CopyToAll"=FALSE}] {"AgingParams"."timetocheck" min=1.0; "JVParameters"."End" min=-2.0 max=2.0; "JVParameters"."Start" min=-2.0 max=2.0; "Channel" items=["1", "2", "3", "4", "5", "6", "7", "8", "9", "10", "11", "12", "13", "14", "15", "16"]}
  in  "Directory to save files":path=path "C:/EC-Lab Development Package/Examples/Labview/V12/DefaultAging"
  in  "Autosave":bool
  out "Active 9":bool
  out "Active 10":bool
  out "Active 11":bool
  out "Active 12":bool
  out "Active 13":bool
  out "Active 14":bool
  out "Active 15":bool
  out "Active 16":bool
  out "IntA 2":dbl caption="suns" format="%#_3g"
  out "T78 2":dbl format="%#_3g"
  out "T56 2":dbl format="%#_3g"
  out "T34 2":dbl format="%#_3g"
  out "T12 2":dbl format="%#_3g"
  out "Voc 9":dbl=-0.7008459568023682 format="%#_4g"
  out "Voc 10":dbl=-0.948243260383606 format="%#_4g"
  out "Voc 11":dbl=-0.5114282369613647 format="%#_4g"
  out "Voc 12":dbl=-0.7734385132789612 format="%#_4g"
  out "Voc 14":dbl=-0.5110825896263123 format="%#_4g"
  out "Voc 13":dbl=-0.6023858189582825 format="%#_4g"
  out "Voc 15":dbl=0.19164180755615234 format="%#_4g"
  out "Voc 16":dbl=0.2513234615325928 format="%#_4g"
  in  "FitCurves":bool
  in  "ExportAgingToExcel":bool
  out "JVParametersLastJV":dbl[][](array[numeric]) format="%#_3g"
  out "XY Graph 3":T5(graph) caption="XY Graph"
  out "XY Graph 4":T5(graph) caption="XY Graph"
  out "XY Graph 5":T5(graph) caption="XY Graph"
  out "XY Graph 6":T5(graph) caption="XY Graph"
  out "XY Graph 7":T5(graph) caption="XY Graph"
  out "XY Graph 8":T5(graph) caption="XY Graph"
  in  "Display Data for:":i32[](listbox)=[13]
  in  "Selected to draw":T6(ring) caption="Draw"
  out "XY Graph 9":T5(graph) caption="XY Graph"
  in  "FitCurves 2":bool
  in  "FitCurves 3":bool
  in  "FitCurves 4":bool
  in  "FitCurves 5":bool
  in  "FitCurves 6":bool
  in  "Draw 3":T7(ring)=enum."P mW/cm2" caption="Draw"
  out "Active":bool
  out "P (mW/cm2)":sgl
  out "J (mA/cm2)":sgl
  out "V (V)":sgl=0.25132346
  out "time (s)":sgl
  in  "Draw":enum16{"P(t)", "V(t)", "I(t)"}(ring)=enum."V(t)"
  out "Number of points":i32=1
  out "XY Graph 2":T9(graph)={"ExchangeCAData"=[0.0], "ExchangeCAData"=[0.2513234615325928]} caption="XY Graph"
  in  "Show Instance":u8(ring) items=["1", "2", "3", "4", "5", "6", "7", "8", "9", "10", "11", "12", "13", "14", "15", "16"]
  out "LiveViewData":cluster{"JVData":sgl[][], "AgingData":sgl[][]}[](array[cluster])=[{"JVData"=array133x5[665 elements], "AgingData"=[[0.0, 0.25132346, 0.0, 1.0]]}, {"JVData"=array89x5[445 elements], "AgingData"=array682x3[2046 elements]}, {"JVData"=[[3.07914, 1.0002275, 9.958126e-09, 0.9997951, 1.0], [3.2463598, 0.95003825, 2.1757216e-08, 0.9520022, 1.0], [3.4136999, 0.89984906, 3.7805787e-08, 0.90010446, 1.0], [3.5809798, 0.8496599, -3.234939e-08, 0.8519322, 1.0], [3.74826, 0.7994708, 9.835428e-09, 0.79722506, 1.0], [3.91554, 0.74928164, -5.833279e-08, 0.7560611, 1.0], [4.08288, 0.6990925, -1.44667e-08, 0.6984071, 1.0], [4.2501597, 0.6489033, 1.3045136e-08, 0.64890647, 1.0], [4.41744, 0.5987142, 3.444323e-08, 0.6010701, 1.0], [4.5847797, 0.54852504, -3.4030673e-08, 0.5464241, 1.0], [4.75206, 0.49833587, 5.2020237e-08, 0.49976334, 1.0], [4.9193397, 0.44814673, 5.7064067e-08, 0.4450562, 1.0], [5.08662, 0.39795756, -9.57571e-09, 0.40031934, 1.0], [5.2539597, 0.34776843, 3.5207446e-08, 0.34518468, 1.0], [5.42124, 0.29757926, -2.0274754e-08, 0.30434132, 1.0], [5.58852, 0.2473901, -7.58874e-09, 0.24774085, 1.0], [5.75586, 0.19720097, 4.972759e-08, 0.19575147, 1.0], [5.92314, 0.14701182, -5.5581605e-08, 0.15440427, 1.0], [6.09042, 0.096822664, -3.1738015e-08, 0.099987194, 1.0], [6.2577, 0.046633508, -1.24797355e-08, 0.049051344, 1.0], [6.42504, -0.0035556422, -3.69347e-08, -0.0022356801, 1.0], [6.59232, -0.05374479, -2.699987e-08, -0.04924751, 1.0], [6.7595997, -0.10393394, -3.4336352e-08, -0.100366585, 1.0], [6.92694, -0.15412308, 2.7259583e-08, -0.15919624, 1.0], [7.0798197, -0.20000151, -7.9578044e-08, -0.1976577, 1.0], [7.2471, -0.14981236, -6.108396e-08, -0.1461722, 1.0], [7.4144397, -0.09962321, 4.926905e-08, -0.10051926, 1.0], [7.58172, -0.049434066, -4.2131372e-08, -0.046911426, 1.0], [7.7489996, 0.0007550822, -3.510057e-08, -0.00041872347, 1.0], [7.91628, 0.050944235, 1.0643253e-07, 0.044424977, 1.0], [8.08362, 0.101133384, -2.8528309e-08, 0.10162093, 1.0], [8.250899, 0.15132254, -2.2414564e-08, 0.15435848, 1.0], [8.4181795, 0.20151168, -4.0602938e-08, 0.20494314, 1.0], [8.58552, 0.25170085, -3.418351e-08, 0.25502396, 1.0], [8.7528, 0.30189, -1.1715516e-08, 0.30941048, 1.0], [8.92008, 0.35207915, 4.3308155e-08, 0.3432456, 1.0], [9.087359, 0.4022683, 2.2062904e-08, 0.39781532, 1.0], [9.2547, 0.45245743, -2.3178778e-08, 0.45491967, 1.0], [9.42198, 0.5026466, -6.016691e-08, 0.5006184, 1.0], [9.58926, 0.55283576, -1.1442636e-07, 0.56295985, 1.0]], "AgingData"=array326x3[978 elements]}, {"JVData"=[[3.0790799, 1.0001799, 5.3355116e-09, 0.9998571, 1.0], [3.2463, 0.9499914, -9.22995e-12, 0.9462215, 1.0], [3.41358, 0.8998029, -5.361627e-09, 0.9083466, 1.0], [3.58092, 0.8496145, -2.2642176e-08, 0.84980154, 1.0], [3.7482, 0.799426, 1.0688549e-07, 0.7932258, 1.0], [3.91548, 0.74923754, -1.759565e-08, 0.75158024, 1.0], [4.08276, 0.6990491, -2.914825e-09, 0.70146203, 1.0], [4.2500997, 0.64886063, 4.785635e-08, 0.6504126, 1.0], [4.41738, 0.59867215, 9.625048e-09, 0.5979435, 1.0], [4.58466, 0.54848367, -1.2396183e-08, 0.5513975, 1.0], [4.75194, 0.49829522, 6.345473e-08, 0.491906, 1.0], [4.91928, 0.44810674, 2.2011998e-08, 0.4528098, 1.0], [5.08656, 0.39791828, 4.0515943e-08, 0.3955777, 1.0], [5.25384, 0.3477298, 5.6878946e-08, 0.34668076, 1.0], [5.4211197, 0.29754135, -9.604628e-08, 0.30590534, 1.0], [5.58846, 0.24735287, 9.013345e-09, 0.24722293, 1.0], [5.7557397, 0.1971644, 5.9325743e-08, 0.19342564, 1.0], [5.92302, 0.14697593, -3.028844e-08, 0.15090989, 1.0], [6.0903, 0.09678746, -4.9251167e-08, 0.10161606, 1.0], [6.25764, 0.046598993, 1.4369164e-10, 0.04584945, 1.0], [6.4249196, -0.0035894734, -4.435756e-08, -0.00521524, 1.0], [6.5922, -0.053777937, 2.1317061e-09, -0.05450907, 1.0], [0.5082, -0.6647468, -1.2796141e-08, -0.6640006, 1.0], [1.0162799, -0.6545854, 3.784564e-08, -0.6567539, 1.0]], "AgingData"=array474x3[1422 elements]}, {"JVData"=[[3.0792599, 1.0001653, 5.946803e-09, 1.0001053, 1.0], [3.24648, 0.949974, -6.6066896e-08, 0.95460665, 1.0], [3.41382, 0.89978266, -6.530285e-08, 0.90336657, 1.0], [3.5811, 0.8495914, 8.6590035e-08, 0.84367305, 1.0], [3.7484398, 0.79940003, -2.1140826e-08, 0.7968202, 1.0], [3.91572, 0.7492087, -2.1446452e-08, 0.7541558, 1.0], [4.0829997, 0.6990174, -4.8188134e-08, 0.7052545, 1.0], [4.25034, 0.64882606, 1.1254829e-08, 0.65178263, 1.0], [4.4176197, 0.5986348, -5.8884844e-08, 0.6038444, 1.0], [4.58496, 0.54844344, 4.594265e-08, 0.54645914, 1.0], [4.7522397, 0.4982521, 2.1645896e-08, 0.5013795, 1.0], [4.91952, 0.44806078, 1.5046452e-07, 0.43668732, 1.0], [5.0868597, 0.39786944, -1.6707412e-07, 0.40697056, 1.0], [5.25414, 0.34767812, -4.331764e-09, 0.3509611, 1.0], [5.4214797, 0.2974868, 2.3938037e-08, 0.29353002, 1.0], [5.58876, 0.24729547, -2.5419501e-08, 0.2470593, 1.0], [5.7560396, 0.19710416, 6.9761557e-09, 0.19588034, 1.0], [5.92338, 0.14691283, -6.912309e-08, 0.15127456, 1.0], [6.0906596, 0.0967215, -1.7473404e-08, 0.09949945, 1.0], [6.258, 0.04653018, 1.4005404e-08, 0.04480463, 1.0], [6.4252796, -0.0036611457, -3.703305e-08, -0.0013145087, 1.0], [6.59256, -0.053852465, -5.5675827e-08, -0.051820844, 1.0], [6.7598996, -0.10404379, 5.2207838e-08, -0.10769272, 1.0], [6.92718, -0.15423511, -9.0688665e-09, -0.15569209, 1.0], [7.0801196, -0.20011552, -1.8868072e-09, -0.20259082, 1.0], [7.2474, -0.14992419, 3.1731343e-08, -0.151259, 1.0], [7.4147396, -0.099732876, -1.5792498e-08, -0.098383285, 1.0], [7.58202, -0.049541555, 8.9646235e-08, -0.056819506, 1.0], [7.7493596, 0.00064976525, 2.2409939e-08, -0.0017731013, 1.0], [7.91664, 0.05084109, -3.1073473e-08, 0.055077106, 1.0], [8.08392, 0.10103241, 7.497649e-08, 0.09262056, 1.0], [8.25126, 0.15122373, 2.7147042e-08, 0.15106057, 1.0], [8.41854, 0.20141506, -4.085329e-08, 0.206856, 1.0], [8.585879, 0.2516064, -2.7558846e-08, 0.25670502, 1.0], [8.7531595, 0.30179772, 2.5466141e-08, 0.30317575, 1.0], [8.92044, 0.35198903, -5.1702784e-08, 0.36140174, 1.0], [9.08778, 0.40218034, -4.6354437e-08, 0.40365338, 1.0], [9.25506, 0.4523717, -9.374485e-09, 0.4568654, 1.0], [9.4223995, 0.502563, 9.0104656e-08, 0.49687, 1.0], [9.58968, 0.55275434, 6.764162e-08, 0.5450987, 1.0], [9.75696, 0.6029457, 5.2952487e-09, 0.60003805, 1.0], [9.9243, 0.65313697, -2.9239741e-08, 0.65580297, 1.0], [10.091579, 0.7033283, 9.971579e-11, 0.70409274, 1.0], [3.0948598, -0.5967237, 1.23362565e-08, -0.5965496, 1.0]], "AgingData"=array342x3[1026 elements]}, {"JVData"=[[0.16746, 0.9498421, -3.7238106e-08, 0.9521123, 1.0], [0.3348, 0.899643, -6.0527117e-09, 0.9032217, 1.0], [0.50207996, 0.849444, -6.093289e-08, 0.85836333, 1.0], [0.66942, 0.79924494, -7.89715e-08, 0.80652505, 1.0], [0.83676, 0.7490459, 3.30819e-08, 0.752304, 1.0], [1.0041, 0.6988469, 7.552681e-09, 0.6958531, 1.0]], "AgingData"=[[0.0, -0.27385262, -0.00088946975], [0.0, -0.5112182, 0.0004154984], [2.0, -0.06918946, 7.042664e-05], [4.0, -0.093550734, -8.228485e-05], [0.0, -0.61836976, 5.6613615e-05], [2.0, -0.5800316, -0.00027317417], [4.0, -0.5014493, -4.4106928e-05], [6.0, -0.36604953, -0.00019681842], [8.0, -0.23225343, 3.224882e-05], [10.0, -0.2007136, -4.4106928e-05], [12.0, -0.2059066, 0.00010860457], [14.0, -0.20323373, 0.00010860457], [16.0, -0.21033593, -0.00027317417], [18.0, -0.21904184, 3.224882e-05], [20.0, -0.23691186, 0.00010860457], [22.0, -0.2476797, 3.224882e-05], [0.0, -0.27289036, 7.493925e-05], [2.0, -0.28011072, -2.5781526e-05], [4.0, -0.28629652, -0.000102137274], [6.0, -0.2959952, -2.5781526e-05], [8.0, -0.3174545, -0.000102137274], [10.0, -0.33226982, 0.00020328572], [12.0, -0.37259194, 0.00012692997], [14.0, -0.51142824, 0.00020328572]]}, {"JVData"=[[0.50838, -0.7533297, 3.3713125e-08, -0.754186, 1.0], [1.01658, -0.74316514, -1.8526524e-08, -0.7415677, 1.0], [1.52484, -0.7330006, -1.3213221e-08, -0.730666, 1.0], [2.03304, -0.7228361, -2.0536646e-08, -0.7224946, 1.0], [2.54124, -0.7126715, -4.6319983e-09, -0.7157485, 1.0], [3.0495, -0.70250696, 2.0711987e-08, -0.70280004, 1.0], [3.5577, -0.69234246, -1.360114e-08, -0.69154114, 1.0], [4.06596, -0.6821779, 1.00148485e-08, -0.68209034, 1.0]], "AgingData"=[[0.0, -0.10874961, -0.0005815154], [2.0, -0.37434164, -4.2873908e-05], [4.0, -0.5594564, -0.00011923032], [0.0, -1.571388, -0.0021865703], [2.0, -0.9579511, 0.00010831172], [4.0, -0.8996827, -0.00019711393], [0.0, -0.81472254, -0.0005532635], [2.0, -0.7945132, -0.00024369123], [4.0, -0.7643481, -9.0978414e-05], [6.0, -0.67538, -1.46220045e-05], [8.0, -0.58190614, -9.0978414e-05], [10.0, -0.5370021, -9.0978414e-05], [12.0, -0.53486377, 0.00021444722], [14.0, -0.5418896, -0.00032004766], [16.0, -0.5460135, -9.0978414e-05], [18.0, -0.5487627, -1.46220045e-05], [20.0, -0.5612869, 6.1734405e-05], [22.0, -0.5698401, -1.46220045e-05], [0.0, -0.7470461, -0.0005593721], [2.0, -0.81696755, 0.0001319822], [4.0, -0.88157445, -9.708702e-05], [6.0, -0.9173908, 5.5625802e-05], [8.0, -0.94289756, -0.00017344343], [10.0, -0.9694734, -2.0730608e-05], [12.0, -0.9618367, -9.708702e-05], [14.0, -0.94824326, 0.000284695]]}, {"JVData"=[[0.1674, 0.94984764, -2.53673e-08, 0.95032424, 1.0], [0.33468, 0.89965886, 2.5059206e-08, 0.90274954, 1.0], [0.50202, 0.84947014, 4.599384e-08, 0.8470317, 1.0], [0.66929996, 0.7992814, 2.8115352e-08, 0.80051106, 1.0], [0.83658, 0.7490927, 7.716658e-08, 0.74543494, 1.0], [1.00392, 0.698904, 1.527952e-08, 0.69605744, 1.0], [1.1711999, 0.64871526, -8.1294864e-08, 0.65673256, 1.0], [1.33848, 0.59852654, -2.446165e-09, 0.5987537, 1.0], [1.50576, 0.5483378, 1.2223366e-08, 0.54815394, 1.0], [1.6731, 0.49814907, -1.2237014e-09, 0.4994944, 1.0], [1.84038, 0.44796032, -4.5385075e-08, 0.45431826, 1.0], [2.00766, 0.3977716, 7.518008e-08, 0.39097688, 1.0], [2.1749399, 0.34758288, -7.029272e-08, 0.3521104, 1.0], [2.34228, 0.29739416, -8.037802e-08, 0.30120507, 1.0], [2.5095599, 0.2472054, 1.1764944e-08, 0.25023863, 1.0], [2.6768398, 0.19701669, -3.5605403e-08, 0.2051541, 1.0], [2.84412, 0.14682795, -6.295796e-08, 0.14795439, 1.0], [3.0114598, 0.09663922, -1.0708939e-09, 0.095765725, 1.0], [3.17874, 0.046450496, 3.590854e-08, 0.046586785, 1.0], [3.34602, -0.003738234, 2.9490622e-08, -0.0043338123, 1.0], [3.5133, -0.05392696, -3.8355942e-08, -0.042894743, 1.0], [3.68064, -0.10411569, 2.4600778e-08, -0.10817639, 1.0], [3.84792, -0.15430441, -1.6821268e-09, -0.15341367, 1.0], [3.9998398, -0.19987454, -4.4315435e-08, -0.19512181, 1.0], [4.16712, -0.14968581, -1.1920225e-08, -0.1442165, 1.0], [4.3343997, -0.09949709, 1.1827183e-07, -0.11188886, 1.0], [4.50174, -0.049308363, 3.207719e-09, -0.047019724, 1.0], [4.6690197, 0.00088036037, 1.2209202e-07, -0.00674769, 1.0], [4.8363, 0.05106909, 6.569485e-09, 0.054225642, 1.0], [5.0036397, 0.101257816, 3.5133425e-09, 0.10215181, 1.0], [5.17092, 0.15144655, 1.0848095e-08, 0.15154463, 1.0], [5.3382, 0.20163527, 1.1459326e-08, 0.20368746, 1.0], [5.50548, 0.25182402, -1.7115688e-08, 0.25315666, 1.0], [5.67282, 0.30201274, 6.264987e-08, 0.29463565, 1.0], [5.8401, 0.35220146, 1.7877248e-08, 0.350934, 1.0], [6.00738, 0.40239018, -3.224364e-08, 0.40428376, 1.0], [6.1746597, 0.45257893, 4.8886095e-09, 0.4554946, 1.0], [6.342, 0.5027677, -4.0648054e-08, 0.5062319, 1.0], [6.5092797, 0.5529564, 1.4821096e-08, 0.55712193, 1.0], [6.67656, 0.6031451, -1.3448305e-08, 0.60238975, 1.0], [6.8438396, 0.65333384, -1.1920232e-08, 0.6556937, 1.0], [7.01118, 0.70352256, 1.1764944e-08, 0.7035129, 1.0], [7.1784596, 0.7537113, 7.73194e-08, 0.74700856, 1.0]], "AgingData"=array258x4[1032 elements]}, {"JVData"=[[1.0013499, 1.210579e-05, 1.1001669, 1.0], [2.00265, 5.280055e-06, 1.0000192, 1.0], [3.0038998, 7.4926476e-07, 0.8999563, 1.0], [4.00515, 5.459907e-08, 0.7997196, 1.0], [5.0064, -1.6849775e-07, 0.6995634, 1.0], [6.0077, -3.4968886e-07, 0.5993691, 1.0], [7.0089498, -5.469176e-07, 0.49931043, 1.0], [8.0102, -7.4393e-07, 0.39910764, 1.0], [9.01145, -9.556986e-07, 0.29895997, 1.0], [10.01275, -1.2210978e-06, 0.19898194, 1.0], [11.014, -1.4915547e-06, 0.098842725, 1.0], [12.015249, -1.7013582e-06, -0.0013897662, 1.0], [13.0164995, -1.8637089e-06, -0.101503514, 1.0]], "AgingData"=[[0.2513, 5.4381195e-05, 1.0503782, 1.0], [0.5025, 2.778111e-05, 1.0002986, 1.0], [0.75369996, 3.9110714e-06, 0.94982845, 1.0], [1.0049, -2.2766604e-05, 0.8997149, 1.0], [1.2560999, -5.2547082e-05, 0.8493892, 1.0], [1.5073, -8.9432746e-05, 0.7991992, 1.0], [1.7585, -0.00013286466, 0.74895835, 1.0], [2.0097, -0.00018626524, 0.6987514, 1.0], [2.2609, -0.00024645546, 0.6484681, 1.0], [2.5121, -0.0003150903, 0.5982187, 1.0], [2.7633, -0.0003903196, 0.5479184, 1.0], [3.0144498, -0.00046932563, 0.49767745, 1.0], [3.26565, -0.0005563859, 0.44752148, 1.0], [3.51685, -0.00064487197, 0.397323, 1.0], [3.76805, -0.00073117693, 0.34696326, 1.0], [4.01925, -0.0008170999, 0.29672235, 1.0], [4.27045, -0.0009031756, 0.24646449, 1.0], [4.52165, -0.0009820798, 0.19614716, 1.0], [4.77285, -0.0010612556, 0.14594024, 1.0], [5.0240498, -0.0011366602, 0.0958352, 1.0], [5.27525, -0.0012121152, 0.04556884, 1.0], [5.5264497, -0.0012991133, -0.0047399844, 1.0], [5.77765, -0.0013793214, -0.05493842, 1.0], [6.02885, -0.0014648766, -0.10519629, 1.0], [6.28005, -0.001559259, -0.15536925, 1.0], [6.53125, -0.001651095, -0.20566109, 1.0], [6.7824497, -0.0017487028, -0.255885, 1.0]]}, {"JVData"=[[1.0013499, 1.210579e-05, 1.1001669, 1.0], [2.00265, 5.280055e-06, 1.0000192, 1.0], [3.0038998, 7.4926476e-07, 0.8999563, 1.0], [4.00515, 5.459907e-08, 0.7997196, 1.0], [5.0064, -1.6849775e-07, 0.6995634, 1.0], [6.0077, -3.4968886e-07, 0.5993691, 1.0], [7.0089498, -5.469176e-07, 0.49931043, 1.0], [8.0102, -7.4393e-07, 0.39910764, 1.0], [9.01145, -9.556986e-07, 0.29895997, 1.0], [10.01275, -1.2210978e-06, 0.19898194, 1.0], [11.014, -1.4915547e-06, 0.098842725, 1.0], [12.015249, -1.7013582e-06, -0.0013897662, 1.0], [13.0164995, -1.8637089e-06, -0.101503514, 1.0]], "AgingData"=[[0.2513, 5.4381195e-05, 1.0503782, 1.0], [0.5025, 2.778111e-05, 1.0002986, 1.0], [0.75369996, 3.9110714e-06, 0.94982845, 1.0], [1.0049, -2.2766604e-05, 0.8997149, 1.0], [1.2560999, -5.2547082e-05, 0.8493892, 1.0], [1.5073, -8.9432746e-05, 0.7991992, 1.0], [1.7585, -0.00013286466, 0.74895835, 1.0], [2.0097, -0.00018626524, 0.6987514, 1.0], [2.2609, -0.00024645546, 0.6484681, 1.0], [2.5121, -0.0003150903, 0.5982187, 1.0], [2.7633, -0.0003903196, 0.5479184, 1.0], [3.0144498, -0.00046932563, 0.49767745, 1.0], [3.26565, -0.0005563859, 0.44752148, 1.0], [3.51685, -0.00064487197, 0.397323, 1.0], [3.76805, -0.00073117693, 0.34696326, 1.0], [4.01925, -0.0008170999, 0.29672235, 1.0], [4.27045, -0.0009031756, 0.24646449, 1.0], [4.52165, -0.0009820798, 0.19614716, 1.0], [4.77285, -0.0010612556, 0.14594024, 1.0], [5.0240498, -0.0011366602, 0.0958352, 1.0], [5.27525, -0.0012121152, 0.04556884, 1.0], [5.5264497, -0.0012991133, -0.0047399844, 1.0], [5.77765, -0.0013793214, -0.05493842, 1.0], [6.02885, -0.0014648766, -0.10519629, 1.0], [6.28005, -0.001559259, -0.15536925, 1.0], [6.53125, -0.001651095, -0.20566109, 1.0], [6.7824497, -0.0017487028, -0.255885, 1.0]]}, {"JVData"=[[1.0013499, 1.210579e-05, 1.1001669, 1.0], [2.00265, 5.280055e-06, 1.0000192, 1.0], [3.0038998, 7.4926476e-07, 0.8999563, 1.0], [4.00515, 5.459907e-08, 0.7997196, 1.0], [5.0064, -1.6849775e-07, 0.6995634, 1.0], [6.0077, -3.4968886e-07, 0.5993691, 1.0], [7.0089498, -5.469176e-07, 0.49931043, 1.0], [8.0102, -7.4393e-07, 0.39910764, 1.0], [9.01145, -9.556986e-07, 0.29895997, 1.0], [10.01275, -1.2210978e-06, 0.19898194, 1.0], [11.014, -1.4915547e-06, 0.098842725, 1.0], [12.015249, -1.7013582e-06, -0.0013897662, 1.0], [13.0164995, -1.8637089e-06, -0.101503514, 1.0]], "AgingData"=[[0.2513, 5.4381195e-05, 1.0503782, 1.0], [0.5025, 2.778111e-05, 1.0002986, 1.0], [0.75369996, 3.9110714e-06, 0.94982845, 1.0], [1.0049, -2.2766604e-05, 0.8997149, 1.0], [1.2560999, -5.2547082e-05, 0.8493892, 1.0], [1.5073, -8.9432746e-05, 0.7991992, 1.0], [1.7585, -0.00013286466, 0.74895835, 1.0], [2.0097, -0.00018626524, 0.6987514, 1.0], [2.2609, -0.00024645546, 0.6484681, 1.0], [2.5121, -0.0003150903, 0.5982187, 1.0], [2.7633, -0.0003903196, 0.5479184, 1.0], [3.0144498, -0.00046932563, 0.49767745, 1.0], [3.26565, -0.0005563859, 0.44752148, 1.0], [3.51685, -0.00064487197, 0.397323, 1.0], [3.76805, -0.00073117693, 0.34696326, 1.0], [4.01925, -0.0008170999, 0.29672235, 1.0], [4.27045, -0.0009031756, 0.24646449, 1.0], [4.52165, -0.0009820798, 0.19614716, 1.0], [4.77285, -0.0010612556, 0.14594024, 1.0], [5.0240498, -0.0011366602, 0.0958352, 1.0], [5.27525, -0.0012121152, 0.04556884, 1.0], [5.5264497, -0.0012991133, -0.0047399844, 1.0], [5.77765, -0.0013793214, -0.05493842, 1.0], [6.02885, -0.0014648766, -0.10519629, 1.0], [6.28005, -0.001559259, -0.15536925, 1.0], [6.53125, -0.001651095, -0.20566109, 1.0], [6.7824497, -0.0017487028, -0.255885, 1.0]]}, {"JVData"=[[1.0013499, 1.210579e-05, 1.1001669, 1.0], [2.00265, 5.280055e-06, 1.0000192, 1.0], [3.0038998, 7.4926476e-07, 0.8999563, 1.0], [4.00515, 5.459907e-08, 0.7997196, 1.0], [5.0064, -1.6849775e-07, 0.6995634, 1.0], [6.0077, -3.4968886e-07, 0.5993691, 1.0], [7.0089498, -5.469176e-07, 0.49931043, 1.0], [8.0102, -7.4393e-07, 0.39910764, 1.0], [9.01145, -9.556986e-07, 0.29895997, 1.0], [10.01275, -1.2210978e-06, 0.19898194, 1.0], [11.014, -1.4915547e-06, 0.098842725, 1.0], [12.015249, -1.7013582e-06, -0.0013897662, 1.0], [13.0164995, -1.8637089e-06, -0.101503514, 1.0]], "AgingData"=[[0.2513, 5.4381195e-05, 1.0503782, 1.0], [0.5025, 2.778111e-05, 1.0002986, 1.0], [0.75369996, 3.9110714e-06, 0.94982845, 1.0], [1.0049, -2.2766604e-05, 0.8997149, 1.0], [1.2560999, -5.2547082e-05, 0.8493892, 1.0], [1.5073, -8.9432746e-05, 0.7991992, 1.0], [1.7585, -0.00013286466, 0.74895835, 1.0], [2.0097, -0.00018626524, 0.6987514, 1.0], [2.2609, -0.00024645546, 0.6484681, 1.0], [2.5121, -0.0003150903, 0.5982187, 1.0], [2.7633, -0.0003903196, 0.5479184, 1.0], [3.0144498, -0.00046932563, 0.49767745, 1.0], [3.26565, -0.0005563859, 0.44752148, 1.0], [3.51685, -0.00064487197, 0.397323, 1.0], [3.76805, -0.00073117693, 0.34696326, 1.0], [4.01925, -0.0008170999, 0.29672235, 1.0], [4.27045, -0.0009031756, 0.24646449, 1.0], [4.52165, -0.0009820798, 0.19614716, 1.0], [4.77285, -0.0010612556, 0.14594024, 1.0], [5.0240498, -0.0011366602, 0.0958352, 1.0], [5.27525, -0.0012121152, 0.04556884, 1.0], [5.5264497, -0.0012991133, -0.0047399844, 1.0], [5.77765, -0.0013793214, -0.05493842, 1.0], [6.02885, -0.0014648766, -0.10519629, 1.0], [6.28005, -0.001559259, -0.15536925, 1.0], [6.53125, -0.001651095, -0.20566109, 1.0], [6.7824497, -0.0017487028, -0.255885, 1.0]]}, {"JVData"=[[1.0013499, 1.210579e-05, 1.1001669, 1.0], [2.00265, 5.280055e-06, 1.0000192, 1.0], [3.0038998, 7.4926476e-07, 0.8999563, 1.0], [4.00515, 5.459907e-08, 0.7997196, 1.0], [5.0064, -1.6849775e-07, 0.6995634, 1.0], [6.0077, -3.4968886e-07, 0.5993691, 1.0], [7.0089498, -5.469176e-07, 0.49931043, 1.0], [8.0102, -7.4393e-07, 0.39910764, 1.0], [9.01145, -9.556986e-07, 0.29895997, 1.0], [10.01275, -1.2210978e-06, 0.19898194, 1.0], [11.014, -1.4915547e-06, 0.098842725, 1.0], [12.015249, -1.7013582e-06, -0.0013897662, 1.0], [13.0164995, -1.8637089e-06, -0.101503514, 1.0]], "AgingData"=[[0.2513, 5.4381195e-05, 1.0503782, 1.0], [0.5025, 2.778111e-05, 1.0002986, 1.0], [0.75369996, 3.9110714e-06, 0.94982845, 1.0], [1.0049, -2.2766604e-05, 0.8997149, 1.0], [1.2560999, -5.2547082e-05, 0.8493892, 1.0], [1.5073, -8.9432746e-05, 0.7991992, 1.0], [1.7585, -0.00013286466, 0.74895835, 1.0], [2.0097, -0.00018626524, 0.6987514, 1.0], [2.2609, -0.00024645546, 0.6484681, 1.0], [2.5121, -0.0003150903, 0.5982187, 1.0], [2.7633, -0.0003903196, 0.5479184, 1.0], [3.0144498, -0.00046932563, 0.49767745, 1.0], [3.26565, -0.0005563859, 0.44752148, 1.0], [3.51685, -0.00064487197, 0.397323, 1.0], [3.76805, -0.00073117693, 0.34696326, 1.0], [4.01925, -0.0008170999, 0.29672235, 1.0], [4.27045, -0.0009031756, 0.24646449, 1.0], [4.52165, -0.0009820798, 0.19614716, 1.0], [4.77285, -0.0010612556, 0.14594024, 1.0], [5.0240498, -0.0011366602, 0.0958352, 1.0], [5.27525, -0.0012121152, 0.04556884, 1.0], [5.5264497, -0.0012991133, -0.0047399844, 1.0], [5.77765, -0.0013793214, -0.05493842, 1.0], [6.02885, -0.0014648766, -0.10519629, 1.0], [6.28005, -0.001559259, -0.15536925, 1.0], [6.53125, -0.001651095, -0.20566109, 1.0], [6.7824497, -0.0017487028, -0.255885, 1.0]]}, {"JVData"=[[1.0013499, 1.210579e-05, 1.1001669, 1.0], [2.00265, 5.280055e-06, 1.0000192, 1.0], [3.0038998, 7.4926476e-07, 0.8999563, 1.0], [4.00515, 5.459907e-08, 0.7997196, 1.0], [5.0064, -1.6849775e-07, 0.6995634, 1.0], [6.0077, -3.4968886e-07, 0.5993691, 1.0], [7.0089498, -5.469176e-07, 0.49931043, 1.0], [8.0102, -7.4393e-07, 0.39910764, 1.0], [9.01145, -9.556986e-07, 0.29895997, 1.0], [10.01275, -1.2210978e-06, 0.19898194, 1.0], [11.014, -1.4915547e-06, 0.098842725, 1.0], [12.015249, -1.7013582e-06, -0.0013897662, 1.0], [13.0164995, -1.8637089e-06, -0.101503514, 1.0]], "AgingData"=[[0.2513, 5.4381195e-05, 1.0503782, 1.0], [0.5025, 2.778111e-05, 1.0002986, 1.0], [0.75369996, 3.9110714e-06, 0.94982845, 1.0], [1.0049, -2.2766604e-05, 0.8997149, 1.0], [1.2560999, -5.2547082e-05, 0.8493892, 1.0], [1.5073, -8.9432746e-05, 0.7991992, 1.0], [1.7585, -0.00013286466, 0.74895835, 1.0], [2.0097, -0.00018626524, 0.6987514, 1.0], [2.2609, -0.00024645546, 0.6484681, 1.0], [2.5121, -0.0003150903, 0.5982187, 1.0], [2.7633, -0.0003903196, 0.5479184, 1.0], [3.0144498, -0.00046932563, 0.49767745, 1.0], [3.26565, -0.0005563859, 0.44752148, 1.0], [3.51685, -0.00064487197, 0.397323, 1.0], [3.76805, -0.00073117693, 0.34696326, 1.0], [4.01925, -0.0008170999, 0.29672235, 1.0], [4.27045, -0.0009031756, 0.24646449, 1.0], [4.52165, -0.0009820798, 0.19614716, 1.0], [4.77285, -0.0010612556, 0.14594024, 1.0], [5.0240498, -0.0011366602, 0.0958352, 1.0], [5.27525, -0.0012121152, 0.04556884, 1.0], [5.5264497, -0.0012991133, -0.0047399844, 1.0], [5.77765, -0.0013793214, -0.05493842, 1.0], [6.02885, -0.0014648766, -0.10519629, 1.0], [6.28005, -0.001559259, -0.15536925, 1.0], [6.53125, -0.001651095, -0.20566109, 1.0], [6.7824497, -0.0017487028, -0.255885, 1.0]]}, {"JVData"=[[1.0013499, 1.210579e-05, 1.1001669, 1.0], [2.00265, 5.280055e-06, 1.0000192, 1.0], [3.0038998, 7.4926476e-07, 0.8999563, 1.0], [4.00515, 5.459907e-08, 0.7997196, 1.0], [5.0064, -1.6849775e-07, 0.6995634, 1.0], [6.0077, -3.4968886e-07, 0.5993691, 1.0], [7.0089498, -5.469176e-07, 0.49931043, 1.0], [8.0102, -7.4393e-07, 0.39910764, 1.0], [9.01145, -9.556986e-07, 0.29895997, 1.0], [10.01275, -1.2210978e-06, 0.19898194, 1.0], [11.014, -1.4915547e-06, 0.098842725, 1.0], [12.015249, -1.7013582e-06, -0.0013897662, 1.0], [13.0164995, -1.8637089e-06, -0.101503514, 1.0]], "AgingData"=[[0.2513, 5.4381195e-05, 1.0503782, 1.0], [0.5025, 2.778111e-05, 1.0002986, 1.0], [0.75369996, 3.9110714e-06, 0.94982845, 1.0], [1.0049, -2.2766604e-05, 0.8997149, 1.0], [1.2560999, -5.2547082e-05, 0.8493892, 1.0], [1.5073, -8.9432746e-05, 0.7991992, 1.0], [1.7585, -0.00013286466, 0.74895835, 1.0], [2.0097, -0.00018626524, 0.6987514, 1.0], [2.2609, -0.00024645546, 0.6484681, 1.0], [2.5121, -0.0003150903, 0.5982187, 1.0], [2.7633, -0.0003903196, 0.5479184, 1.0], [3.0144498, -0.00046932563, 0.49767745, 1.0], [3.26565, -0.0005563859, 0.44752148, 1.0], [3.51685, -0.00064487197, 0.397323, 1.0], [3.76805, -0.00073117693, 0.34696326, 1.0], [4.01925, -0.0008170999, 0.29672235, 1.0], [4.27045, -0.0009031756, 0.24646449, 1.0], [4.52165, -0.0009820798, 0.19614716, 1.0], [4.77285, -0.0010612556, 0.14594024, 1.0], [5.0240498, -0.0011366602, 0.0958352, 1.0], [5.27525, -0.0012121152, 0.04556884, 1.0], [5.5264497, -0.0012991133, -0.0047399844, 1.0], [5.77765, -0.0013793214, -0.05493842, 1.0], [6.02885, -0.0014648766, -0.10519629, 1.0], [6.28005, -0.001559259, -0.15536925, 1.0], [6.53125, -0.001651095, -0.20566109, 1.0], [6.7824497, -0.0017487028, -0.255885, 1.0]]}, {"JVData"=[[1.0013499, 1.210579e-05, 1.1001669, 1.0], [2.00265, 5.280055e-06, 1.0000192, 1.0], [3.0038998, 7.4926476e-07, 0.8999563, 1.0], [4.00515, 5.459907e-08, 0.7997196, 1.0], [5.0064, -1.6849775e-07, 0.6995634, 1.0], [6.0077, -3.4968886e-07, 0.5993691, 1.0], [7.0089498, -5.469176e-07, 0.49931043, 1.0], [8.0102, -7.4393e-07, 0.39910764, 1.0], [9.01145, -9.556986e-07, 0.29895997, 1.0], [10.01275, -1.2210978e-06, 0.19898194, 1.0], [11.014, -1.4915547e-06, 0.098842725, 1.0], [12.015249, -1.7013582e-06, -0.0013897662, 1.0], [13.0164995, -1.8637089e-06, -0.101503514, 1.0]], "AgingData"=[[0.2513, 5.4381195e-05, 1.0503782, 1.0], [0.5025, 2.778111e-05, 1.0002986, 1.0], [0.75369996, 3.9110714e-06, 0.94982845, 1.0], [1.0049, -2.2766604e-05, 0.8997149, 1.0], [1.2560999, -5.2547082e-05, 0.8493892, 1.0], [1.5073, -8.9432746e-05, 0.7991992, 1.0], [1.7585, -0.00013286466, 0.74895835, 1.0], [2.0097, -0.00018626524, 0.6987514, 1.0], [2.2609, -0.00024645546, 0.6484681, 1.0], [2.5121, -0.0003150903, 0.5982187, 1.0], [2.7633, -0.0003903196, 0.5479184, 1.0], [3.0144498, -0.00046932563, 0.49767745, 1.0], [3.26565, -0.0005563859, 0.44752148, 1.0], [3.51685, -0.00064487197, 0.397323, 1.0], [3.76805, -0.00073117693, 0.34696326, 1.0], [4.01925, -0.0008170999, 0.29672235, 1.0], [4.27045, -0.0009031756, 0.24646449, 1.0], [4.52165, -0.0009820798, 0.19614716, 1.0], [4.77285, -0.0010612556, 0.14594024, 1.0], [5.0240498, -0.0011366602, 0.0958352, 1.0], [5.27525, -0.0012121152, 0.04556884, 1.0], [5.5264497, -0.0012991133, -0.0047399844, 1.0], [5.77765, -0.0013793214, -0.05493842, 1.0], [6.02885, -0.0014648766, -0.10519629, 1.0], [6.28005, -0.001559259, -0.15536925, 1.0], [6.53125, -0.001651095, -0.20566109, 1.0], [6.7824497, -0.0017487028, -0.255885, 1.0]]}] {"AgingData" format="%.2f"; "JVData" format="%.2f"}
  out "Channel":u8=1
  out "Status":string="stopped"
  in  "DeleteAll Button":bool
  in  "Hide all Button":bool
  in  "Save Button 2":bool
  in  "Project name":string
  in  "Save Button":bool
  in  "Scrollbar":i32(c297)
  in  "DataForAnalysis":T10(array[cluster]) {"Eff" scale=0.0..30.0; "JVmetrics" format="%#_4g"}
  out "XY Graph 10":cluster{"JVData":dbl[], "JVData":dbl[]}[](graph) caption="XY Graph"
  in  "Select how to plot:":T6(ring)=enum."-J(V)" caption="Draw"
  out "XY Graph 11":T11(graph) caption="XY Graph"
  in  "Select how to plot:":enum16{"P(t)", "V(t)", "I(t)"}(ring) caption="Draw"
  out "Final power (mW/cm2)":sgl[](array[numeric])
  in  "Keep latest JV data":i32=200
  in  "Point Style":u8[](array[numeric])=[1, 2, 3, 4, 5, 6, 7, 8, 1, 2, 3, 4, 5, 6, 7, 8]
  in  "Plot Color":u32[](array[colorbox])=[16860, 13172956, 16711708, 16743168, 11838720, 3836160, 29321, 0, 7447295, 16031999, 16746644, 16768136, 2817900, 56063, 9868950]
  in  "JV Stabilized MPP Standard":T12(array[cluster])=[{"name"="Device1", "Channel"=0, "StartCh"=FALSE, "PauseCh"=FALSE, "StopCh"=FALSE, "ActiveArea cm2"=0.16, "AgingMode"=enum."MPP", "JVParameters"={"Hyst"=TRUE, "Start"=0.1, "End"=-0.2, "rate"=20.0, "record dE"=10.0, "equ t1"=1.0, "equ t2"=0.0, "vsInitEnd 2"=FALSE, "vsInitSt 3"=TRUE}, "AgingParams"={"Time"=1.0, "StepV"=0.01, "timetocheck"=1.0, "average over"=1.0}, "start time"=timestamp(3545987186.527957 s since 1904-01-01), "AgingFile"=path "C:/EC-Lab Development Package/Examples/Labview/V12/DefaultAging/Ch1_Device1_160513_14h_26m26s_aging.txt", "JVFile"=path "C:/EC-Lab Development Package/Examples/Labview/V12/DefaultAging/Ch1_Device1_160513_14h_26m26s_JVs.txt", "JVMetricsFile"=path "C:/EC-Lab Development Package/Examples/Labview/V12/DefaultAging/Ch1_Device1_160513_14h_26m26s_JVmetrics.txt", "Status"=0.0, "ColorInd"=FALSE, "RunCont"=FALSE, "StatusStr"="stopped", "CopyToAll"=FALSE}, {"name"="Device2", "Channel"=1, "StartCh"=FALSE, "PauseCh"=FALSE, "StopCh"=FALSE, "ActiveArea cm2"=0.16, "AgingMode"=enum."MPP", "JVParameters"={"Hyst"=TRUE, "Start"=0.1, "End"=-0.2, "rate"=20.0, "record dE"=10.0, "equ t1"=1.0, "equ t2"=0.0, "vsInitEnd 2"=FALSE, "vsInitSt 3"=TRUE}, "AgingParams"={"Time"=1.0, "StepV"=0.01, "timetocheck"=1.0, "average over"=1.0}, "start time"=timestamp(3545986839.128179 s since 1904-01-01), "AgingFile"=path "C:/EC-Lab Development Package/Examples/Labview/V12/DefaultAging/Ch2_Device2_160513_14h_20m39s_aging.txt", "JVFile"=path "C:/EC-Lab Development Package/Examples/Labview/V12/DefaultAging/Ch2_Device2_160513_14h_20m39s_JVs.txt", "JVMetricsFile"=path "C:/EC-Lab Development Package/Examples/Labview/V12/DefaultAging/Ch2_Device2_160513_14h_20m39s_JVmetrics.txt", "Status"=0.0, "ColorInd"=FALSE, "RunCont"=FALSE, "StatusStr"="stopped", "CopyToAll"=FALSE}, {"name"="Device3", "Channel"=2, "StartCh"=FALSE, "PauseCh"=FALSE, "StopCh"=FALSE, "ActiveArea cm2"=0.16, "AgingMode"=enum."MPP", "JVParameters"={"Hyst"=TRUE, "Start"=0.1, "End"=-0.2, "rate"=20.0, "record dE"=10.0, "equ t1"=1.0, "equ t2"=0.0, "vsInitEnd 2"=FALSE, "vsInitSt 3"=TRUE}, "AgingParams"={"Time"=1.0, "StepV"=0.01, "timetocheck"=1.0, "average over"=1.0}, "start time"=timestamp(3545987186.5334716 s since 1904-01-01), "AgingFile"=path "C:/EC-Lab Development Package/Examples/Labview/V12/DefaultAging/Ch3_Device3_160513_14h_26m26s_aging.txt", "JVFile"=path "C:/EC-Lab Development Package/Examples/Labview/V12/DefaultAging/Ch3_Device3_160513_14h_26m26s_JVs.txt", "JVMetricsFile"=path "C:/EC-Lab Development Package/Examples/Labview/V12/DefaultAging/Ch3_Device3_160513_14h_26m26s_JVmetrics.txt", "Status"=0.0, "ColorInd"=FALSE, "RunCont"=FALSE, "StatusStr"="stopped", "CopyToAll"=FALSE}, {"name"="Device4", "Channel"=3, "StartCh"=FALSE, "PauseCh"=FALSE, "StopCh"=FALSE, "ActiveArea cm2"=0.16, "AgingMode"=enum."MPP", "JVParameters"={"Hyst"=TRUE, "Start"=0.1, "End"=-0.2, "rate"=20.0, "record dE"=10.0, "equ t1"=1.0, "equ t2"=0.0, "vsInitEnd 2"=FALSE, "vsInitSt 3"=TRUE}, "AgingParams"={"Time"=1.0, "StepV"=0.01, "timetocheck"=1.0, "average over"=1.0}, "start time"=timestamp(3545987186.5364795 s since 1904-01-01), "AgingFile"=path "C:/EC-Lab Development Package/Examples/Labview/V12/DefaultAging/Ch4_Device4_160513_14h_26m26s_aging.txt", "JVFile"=path "C:/EC-Lab Development Package/Examples/Labview/V12/DefaultAging/Ch4_Device4_160513_14h_26m26s_JVs.txt", "JVMetricsFile"=path "C:/EC-Lab Development Package/Examples/Labview/V12/DefaultAging/Ch4_Device4_160513_14h_26m26s_JVmetrics.txt", "Status"=0.0, "ColorInd"=FALSE, "RunCont"=FALSE, "StatusStr"="stopped", "CopyToAll"=FALSE}, {"name"="Device5", "Channel"=4, "StartCh"=FALSE, "PauseCh"=FALSE, "StopCh"=FALSE, "ActiveArea cm2"=0.16, "AgingMode"=enum."MPP", "JVParameters"={"Hyst"=TRUE, "Start"=0.1, "End"=-0.2, "rate"=20.0, "record dE"=10.0, "equ t1"=1.0, "equ t2"=0.0, "vsInitEnd 2"=FALSE, "vsInitSt 3"=TRUE}, "AgingParams"={"Time"=1.0, "StepV"=0.01, "timetocheck"=1.0, "average over"=1.0}, "start time"=timestamp(3545987186.537483 s since 1904-01-01), "AgingFile"=path "C:/EC-Lab Development Package/Examples/Labview/V12/DefaultAging/Ch5_Device5_160513_14h_26m26s_aging.txt", "JVFile"=path "C:/EC-Lab Development Package/Examples/Labview/V12/DefaultAging/Ch5_Device5_160513_14h_26m26s_JVs.txt", "JVMetricsFile"=path "C:/EC-Lab Development Package/Examples/Labview/V12/DefaultAging/Ch5_Device5_160513_14h_26m26s_JVmetrics.txt", "Status"=0.0, "ColorInd"=FALSE, "RunCont"=FALSE, "StatusStr"="stopped", "CopyToAll"=FALSE}, {"name"="Device6", "Channel"=5, "StartCh"=FALSE, "PauseCh"=FALSE, "StopCh"=FALSE, "ActiveArea cm2"=0.16, "AgingMode"=enum."MPP", "JVParameters"={"Hyst"=TRUE, "Start"=0.1, "End"=-0.2, "rate"=20.0, "record dE"=10.0, "equ t1"=1.0, "equ t2"=0.0, "vsInitEnd 2"=FALSE, "vsInitSt 3"=TRUE}, "AgingParams"={"Time"=1.0, "StepV"=0.01, "timetocheck"=1.0, "average over"=1.0}, "start time"=timestamp(3545987186.5399885 s since 1904-01-01), "AgingFile"=path "C:/EC-Lab Development Package/Examples/Labview/V12/DefaultAging/Ch6_Device6_160513_14h_26m26s_aging.txt", "JVFile"=path "C:/EC-Lab Development Package/Examples/Labview/V12/DefaultAging/Ch6_Device6_160513_14h_26m26s_JVs.txt", "JVMetricsFile"=path "C:/EC-Lab Development Package/Examples/Labview/V12/DefaultAging/Ch6_Device6_160513_14h_26m26s_JVmetrics.txt", "Status"=0.0, "ColorInd"=FALSE, "RunCont"=FALSE, "StatusStr"="stopped", "CopyToAll"=FALSE}, {"name"="Device7", "Channel"=6, "StartCh"=FALSE, "PauseCh"=FALSE, "StopCh"=FALSE, "ActiveArea cm2"=0.16, "AgingMode"=enum."MPP", "JVParameters"={"Hyst"=TRUE, "Start"=0.1, "End"=-0.2, "rate"=20.0, "record dE"=10.0, "equ t1"=1.0, "equ t2"=0.0, "vsInitEnd 2"=FALSE, "vsInitSt 3"=TRUE}, "AgingParams"={"Time"=1.0, "StepV"=0.01, "timetocheck"=1.0, "average over"=1.0}, "start time"=timestamp(3545987186.5446434 s since 1904-01-01), "AgingFile"=path "C:/EC-Lab Development Package/Examples/Labview/V12/DefaultAging/Ch7_Device7_160513_14h_26m26s_aging.txt", "JVFile"=path "C:/EC-Lab Development Package/Examples/Labview/V12/DefaultAging/Ch7_Device7_160513_14h_26m26s_JVs.txt", "JVMetricsFile"=path "C:/EC-Lab Development Package/Examples/Labview/V12/DefaultAging/Ch7_Device7_160513_14h_26m26s_JVmetrics.txt", "Status"=0.0, "ColorInd"=FALSE, "RunCont"=FALSE, "StatusStr"="stopped", "CopyToAll"=FALSE}, {"name"="Device8", "Channel"=7, "StartCh"=FALSE, "PauseCh"=FALSE, "StopCh"=FALSE, "ActiveArea cm2"=0.16, "AgingMode"=enum."MPP", "JVParameters"={"Hyst"=TRUE, "Start"=0.1, "End"=-0.2, "rate"=20.0, "record dE"=10.0, "equ t1"=1.0, "equ t2"=0.0, "vsInitEnd 2"=FALSE, "vsInitSt 3"=TRUE}, "AgingParams"={"Time"=1.0, "StepV"=0.01, "timetocheck"=1.0, "average over"=1.0}, "start time"=timestamp(3545987186.5466247 s since 1904-01-01), "AgingFile"=path "C:/EC-Lab Development Package/Examples/Labview/V12/DefaultAging/Ch8_Device8_160513_14h_26m26s_aging.txt", "JVFile"=path "C:/EC-Lab Development Package/Examples/Labview/V12/DefaultAging/Ch8_Device8_160513_14h_26m26s_JVs.txt", "JVMetricsFile"=path "C:/EC-Lab Development Package/Examples/Labview/V12/DefaultAging/Ch8_Device8_160513_14h_26m26s_JVmetrics.txt", "Status"=0.0, "ColorInd"=FALSE, "RunCont"=FALSE, "StatusStr"="stopped", "CopyToAll"=FALSE}, {"name"="Device9", "Channel"=8, "StartCh"=FALSE, "PauseCh"=FALSE, "StopCh"=FALSE, "ActiveArea cm2"=0.16, "AgingMode"=enum."MPP", "JVParameters"={"Hyst"=TRUE, "Start"=0.1, "End"=-0.2, "rate"=20.0, "record dE"=10.0, "equ t1"=1.0, "equ t2"=0.0, "vsInitEnd 2"=FALSE, "vsInitSt 3"=TRUE}, "AgingParams"={"Time"=1.0, "StepV"=0.01, "timetocheck"=1.0, "average over"=1.0}, "start time"=timestamp(0 s since 1904-01-01), "AgingFile"=path "", "JVFile"=path "", "JVMetricsFile"=path "", "Status"=0.0, "ColorInd"=FALSE, "RunCont"=FALSE, "StatusStr"="", "CopyToAll"=FALSE}, {"name"="Device10", "Channel"=9, "StartCh"=FALSE, "PauseCh"=FALSE, "StopCh"=FALSE, "ActiveArea cm2"=0.16, "AgingMode"=enum."MPP", "JVParameters"={"Hyst"=TRUE, "Start"=0.1, "End"=-0.2, "rate"=20.0, "record dE"=10.0, "equ t1"=1.0, "equ t2"=0.0, "vsInitEnd 2"=FALSE, "vsInitSt 3"=TRUE}, "AgingParams"={"Time"=1.0, "StepV"=0.01, "timetocheck"=1.0, "average over"=1.0}, "start time"=timestamp(0 s since 1904-01-01), "AgingFile"=path "", "JVFile"=path "", "JVMetricsFile"=path "", "Status"=0.0, "ColorInd"=FALSE, "RunCont"=FALSE, "StatusStr"="", "CopyToAll"=FALSE}, {"name"="Device11", "Channel"=10, "StartCh"=FALSE, "PauseCh"=FALSE, "StopCh"=FALSE, "ActiveArea cm2"=0.16, "AgingMode"=enum."MPP", "JVParameters"={"Hyst"=TRUE, "Start"=0.1, "End"=-0.2, "rate"=20.0, "record dE"=10.0, "equ t1"=1.0, "equ t2"=0.0, "vsInitEnd 2"=FALSE, "vsInitSt 3"=TRUE}, "AgingParams"={"Time"=1.0, "StepV"=0.01, "timetocheck"=1.0, "average over"=1.0}, "start time"=timestamp(0 s since 1904-01-01), "AgingFile"=path "", "JVFile"=path "", "JVMetricsFile"=path "", "Status"=0.0, "ColorInd"=FALSE, "RunCont"=FALSE, "StatusStr"="", "CopyToAll"=FALSE}, {"name"="Device12", "Channel"=11, "StartCh"=FALSE, "PauseCh"=FALSE, "StopCh"=FALSE, "ActiveArea cm2"=0.16, "AgingMode"=enum."MPP", "JVParameters"={"Hyst"=TRUE, "Start"=0.1, "End"=-0.2, "rate"=20.0, "record dE"=10.0, "equ t1"=1.0, "equ t2"=0.0, "vsInitEnd 2"=FALSE, "vsInitSt 3"=TRUE}, "AgingParams"={"Time"=1.0, "StepV"=0.01, "timetocheck"=1.0, "average over"=1.0}, "start time"=timestamp(0 s since 1904-01-01), "AgingFile"=path "", "JVFile"=path "", "JVMetricsFile"=path "", "Status"=0.0, "ColorInd"=FALSE, "RunCont"=FALSE, "StatusStr"="", "CopyToAll"=FALSE}, {"name"="Device13", "Channel"=12, "StartCh"=FALSE, "PauseCh"=FALSE, "StopCh"=FALSE, "ActiveArea cm2"=0.16, "AgingMode"=enum."MPP", "JVParameters"={"Hyst"=TRUE, "Start"=0.1, "End"=-0.2, "rate"=20.0, "record dE"=10.0, "equ t1"=1.0, "equ t2"=0.0, "vsInitEnd 2"=FALSE, "vsInitSt 3"=TRUE}, "AgingParams"={"Time"=1.0, "StepV"=0.01, "timetocheck"=1.0, "average over"=1.0}, "start time"=timestamp(0 s since 1904-01-01), "AgingFile"=path "", "JVFile"=path "", "JVMetricsFile"=path "", "Status"=0.0, "ColorInd"=FALSE, "RunCont"=FALSE, "StatusStr"="", "CopyToAll"=FALSE}, {"name"="Device14", "Channel"=13, "StartCh"=FALSE, "PauseCh"=FALSE, "StopCh"=FALSE, "ActiveArea cm2"=0.16, "AgingMode"=enum."MPP", "JVParameters"={"Hyst"=TRUE, "Start"=0.1, "End"=-0.2, "rate"=20.0, "record dE"=10.0, "equ t1"=1.0, "equ t2"=0.0, "vsInitEnd 2"=FALSE, "vsInitSt 3"=TRUE}, "AgingParams"={"Time"=1.0, "StepV"=0.01, "timetocheck"=1.0, "average over"=1.0}, "start time"=timestamp(0 s since 1904-01-01), "AgingFile"=path "", "JVFile"=path "", "JVMetricsFile"=path "", "Status"=0.0, "ColorInd"=FALSE, "RunCont"=FALSE, "StatusStr"="", "CopyToAll"=FALSE}, {"name"="Device15", "Channel"=14, "StartCh"=FALSE, "PauseCh"=FALSE, "StopCh"=FALSE, "ActiveArea cm2"=0.16, "AgingMode"=enum."MPP", "JVParameters"={"Hyst"=TRUE, "Start"=0.1, "End"=-0.2, "rate"=20.0, "record dE"=10.0, "equ t1"=1.0, "equ t2"=0.0, "vsInitEnd 2"=FALSE, "vsInitSt 3"=TRUE}, "AgingParams"={"Time"=1.0, "StepV"=0.01, "timetocheck"=1.0, "average over"=1.0}, "start time"=timestamp(0 s since 1904-01-01), "AgingFile"=path "", "JVFile"=path "", "JVMetricsFile"=path "", "Status"=0.0, "ColorInd"=FALSE, "RunCont"=FALSE, "StatusStr"="", "CopyToAll"=FALSE}, {"name"="Device16", "Channel"=15, "StartCh"=FALSE, "PauseCh"=FALSE, "StopCh"=FALSE, "ActiveArea cm2"=0.16, "AgingMode"=enum."MPP", "JVParameters"={"Hyst"=TRUE, "Start"=0.1, "End"=-0.2, "rate"=20.0, "record dE"=10.0, "equ t1"=1.0, "equ t2"=0.0, "vsInitEnd 2"=FALSE, "vsInitSt 3"=TRUE}, "AgingParams"={"Time"=1.0, "StepV"=0.01, "timetocheck"=1.0, "average over"=1.0}, "start time"=timestamp(0 s since 1904-01-01), "AgingFile"=path "", "JVFile"=path "", "JVMetricsFile"=path "", "Status"=0.0, "ColorInd"=FALSE, "RunCont"=FALSE, "StatusStr"="", "CopyToAll"=FALSE}] {"JVParameters"."End" min=-2.0 max=2.0; "JVParameters"."Start" min=-2.0 max=2.0; "Channel" items=["1", "2", "3", "4", "5", "6", "7", "8", "9", "10", "11", "12", "13", "14", "15", "16"]}
  in  "AgingStandard":T12(array[cluster])=[{"name"="Device1", "Channel"=0, "StartCh"=FALSE, "PauseCh"=FALSE, "StopCh"=FALSE, "ActiveArea cm2"=0.16, "AgingMode"=enum."MPP", "JVParameters"={"Hyst"=TRUE, "Start"=0.1, "End"=-0.2, "rate"=100.0, "record dE"=20.0, "equ t1"=1.0, "equ t2"=0.0, "vsInitEnd 2"=FALSE, "vsInitSt 3"=TRUE}, "AgingParams"={"Time"=30.0, "StepV"=0.01, "timetocheck"=5.0, "average over"=12.0}, "start time"=timestamp(3545987186.527957 s since 1904-01-01), "AgingFile"=path "C:/EC-Lab Development Package/Examples/Labview/V12/DefaultAging/Ch1_Device1_160513_14h_26m26s_aging.txt", "JVFile"=path "C:/EC-Lab Development Package/Examples/Labview/V12/DefaultAging/Ch1_Device1_160513_14h_26m26s_JVs.txt", "JVMetricsFile"=path "C:/EC-Lab Development Package/Examples/Labview/V12/DefaultAging/Ch1_Device1_160513_14h_26m26s_JVmetrics.txt", "Status"=0.0, "ColorInd"=FALSE, "RunCont"=TRUE, "StatusStr"="stopped", "CopyToAll"=FALSE}, {"name"="Device2", "Channel"=1, "StartCh"=FALSE, "PauseCh"=FALSE, "StopCh"=FALSE, "ActiveArea cm2"=0.16, "AgingMode"=enum."MPP", "JVParameters"={"Hyst"=TRUE, "Start"=0.1, "End"=-0.2, "rate"=100.0, "record dE"=20.0, "equ t1"=1.0, "equ t2"=0.0, "vsInitEnd 2"=FALSE, "vsInitSt 3"=TRUE}, "AgingParams"={"Time"=30.0, "StepV"=0.01, "timetocheck"=5.0, "average over"=12.0}, "start time"=timestamp(3545986839.128179 s since 1904-01-01), "AgingFile"=path "C:/EC-Lab Development Package/Examples/Labview/V12/DefaultAging/Ch2_Device2_160513_14h_20m39s_aging.txt", "JVFile"=path "C:/EC-Lab Development Package/Examples/Labview/V12/DefaultAging/Ch2_Device2_160513_14h_20m39s_JVs.txt", "JVMetricsFile"=path "C:/EC-Lab Development Package/Examples/Labview/V12/DefaultAging/Ch2_Device2_160513_14h_20m39s_JVmetrics.txt", "Status"=0.0, "ColorInd"=FALSE, "RunCont"=TRUE, "StatusStr"="stopped", "CopyToAll"=FALSE}, {"name"="Device3", "Channel"=2, "StartCh"=FALSE, "PauseCh"=FALSE, "StopCh"=FALSE, "ActiveArea cm2"=0.16, "AgingMode"=enum."MPP", "JVParameters"={"Hyst"=TRUE, "Start"=0.1, "End"=-0.2, "rate"=100.0, "record dE"=20.0, "equ t1"=1.0, "equ t2"=0.0, "vsInitEnd 2"=FALSE, "vsInitSt 3"=TRUE}, "AgingParams"={"Time"=30.0, "StepV"=0.01, "timetocheck"=5.0, "average over"=12.0}, "start time"=timestamp(3545987186.5334716 s since 1904-01-01), "AgingFile"=path "C:/EC-Lab Development Package/Examples/Labview/V12/DefaultAging/Ch3_Device3_160513_14h_26m26s_aging.txt", "JVFile"=path "C:/EC-Lab Development Package/Examples/Labview/V12/DefaultAging/Ch3_Device3_160513_14h_26m26s_JVs.txt", "JVMetricsFile"=path "C:/EC-Lab Development Package/Examples/Labview/V12/DefaultAging/Ch3_Device3_160513_14h_26m26s_JVmetrics.txt", "Status"=0.0, "ColorInd"=FALSE, "RunCont"=TRUE, "StatusStr"="stopped", "CopyToAll"=FALSE}, {"name"="Device4", "Channel"=3, "StartCh"=FALSE, "PauseCh"=FALSE, "StopCh"=FALSE, "ActiveArea cm2"=0.16, "AgingMode"=enum."MPP", "JVParameters"={"Hyst"=TRUE, "Start"=0.1, "End"=-0.2, "rate"=100.0, "record dE"=20.0, "equ t1"=1.0, "equ t2"=0.0, "vsInitEnd 2"=FALSE, "vsInitSt 3"=TRUE}, "AgingParams"={"Time"=30.0, "StepV"=0.01, "timetocheck"=5.0, "average over"=12.0}, "start time"=timestamp(3545987186.5364795 s since 1904-01-01), "AgingFile"=path "C:/EC-Lab Development Package/Examples/Labview/V12/DefaultAging/Ch4_Device4_160513_14h_26m26s_aging.txt", "JVFile"=path "C:/EC-Lab Development Package/Examples/Labview/V12/DefaultAging/Ch4_Device4_160513_14h_26m26s_JVs.txt", "JVMetricsFile"=path "C:/EC-Lab Development Package/Examples/Labview/V12/DefaultAging/Ch4_Device4_160513_14h_26m26s_JVmetrics.txt", "Status"=0.0, "ColorInd"=FALSE, "RunCont"=TRUE, "StatusStr"="stopped", "CopyToAll"=FALSE}, {"name"="Device5", "Channel"=4, "StartCh"=FALSE, "PauseCh"=FALSE, "StopCh"=FALSE, "ActiveArea cm2"=0.16, "AgingMode"=enum."MPP", "JVParameters"={"Hyst"=TRUE, "Start"=0.1, "End"=-0.2, "rate"=100.0, "record dE"=20.0, "equ t1"=1.0, "equ t2"=0.0, "vsInitEnd 2"=FALSE, "vsInitSt 3"=TRUE}, "AgingParams"={"Time"=30.0, "StepV"=0.01, "timetocheck"=5.0, "average over"=12.0}, "start time"=timestamp(3545987186.537483 s since 1904-01-01), "AgingFile"=path "C:/EC-Lab Development Package/Examples/Labview/V12/DefaultAging/Ch5_Device5_160513_14h_26m26s_aging.txt", "JVFile"=path "C:/EC-Lab Development Package/Examples/Labview/V12/DefaultAging/Ch5_Device5_160513_14h_26m26s_JVs.txt", "JVMetricsFile"=path "C:/EC-Lab Development Package/Examples/Labview/V12/DefaultAging/Ch5_Device5_160513_14h_26m26s_JVmetrics.txt", "Status"=0.0, "ColorInd"=FALSE, "RunCont"=TRUE, "StatusStr"="stopped", "CopyToAll"=FALSE}, {"name"="Device6", "Channel"=5, "StartCh"=FALSE, "PauseCh"=FALSE, "StopCh"=FALSE, "ActiveArea cm2"=0.16, "AgingMode"=enum."MPP", "JVParameters"={"Hyst"=TRUE, "Start"=0.1, "End"=-0.2, "rate"=100.0, "record dE"=20.0, "equ t1"=1.0, "equ t2"=0.0, "vsInitEnd 2"=FALSE, "vsInitSt 3"=TRUE}, "AgingParams"={"Time"=30.0, "StepV"=0.01, "timetocheck"=5.0, "average over"=12.0}, "start time"=timestamp(3545987186.5399885 s since 1904-01-01), "AgingFile"=path "C:/EC-Lab Development Package/Examples/Labview/V12/DefaultAging/Ch6_Device6_160513_14h_26m26s_aging.txt", "JVFile"=path "C:/EC-Lab Development Package/Examples/Labview/V12/DefaultAging/Ch6_Device6_160513_14h_26m26s_JVs.txt", "JVMetricsFile"=path "C:/EC-Lab Development Package/Examples/Labview/V12/DefaultAging/Ch6_Device6_160513_14h_26m26s_JVmetrics.txt", "Status"=0.0, "ColorInd"=FALSE, "RunCont"=TRUE, "StatusStr"="stopped", "CopyToAll"=FALSE}, {"name"="Device7", "Channel"=6, "StartCh"=FALSE, "PauseCh"=FALSE, "StopCh"=FALSE, "ActiveArea cm2"=0.16, "AgingMode"=enum."MPP", "JVParameters"={"Hyst"=TRUE, "Start"=0.1, "End"=-0.2, "rate"=100.0, "record dE"=20.0, "equ t1"=1.0, "equ t2"=0.0, "vsInitEnd 2"=FALSE, "vsInitSt 3"=TRUE}, "AgingParams"={"Time"=30.0, "StepV"=0.01, "timetocheck"=5.0, "average over"=12.0}, "start time"=timestamp(3545987186.5446434 s since 1904-01-01), "AgingFile"=path "C:/EC-Lab Development Package/Examples/Labview/V12/DefaultAging/Ch7_Device7_160513_14h_26m26s_aging.txt", "JVFile"=path "C:/EC-Lab Development Package/Examples/Labview/V12/DefaultAging/Ch7_Device7_160513_14h_26m26s_JVs.txt", "JVMetricsFile"=path "C:/EC-Lab Development Package/Examples/Labview/V12/DefaultAging/Ch7_Device7_160513_14h_26m26s_JVmetrics.txt", "Status"=0.0, "ColorInd"=FALSE, "RunCont"=TRUE, "StatusStr"="stopped", "CopyToAll"=FALSE}, {"name"="Device8", "Channel"=7, "StartCh"=FALSE, "PauseCh"=FALSE, "StopCh"=FALSE, "ActiveArea cm2"=0.16, "AgingMode"=enum."MPP", "JVParameters"={"Hyst"=TRUE, "Start"=0.1, "End"=-0.2, "rate"=100.0, "record dE"=20.0, "equ t1"=1.0, "equ t2"=0.0, "vsInitEnd 2"=FALSE, "vsInitSt 3"=TRUE}, "AgingParams"={"Time"=30.0, "StepV"=0.01, "timetocheck"=5.0, "average over"=12.0}, "start time"=timestamp(3545987186.5466247 s since 1904-01-01), "AgingFile"=path "C:/EC-Lab Development Package/Examples/Labview/V12/DefaultAging/Ch8_Device8_160513_14h_26m26s_aging.txt", "JVFile"=path "C:/EC-Lab Development Package/Examples/Labview/V12/DefaultAging/Ch8_Device8_160513_14h_26m26s_JVs.txt", "JVMetricsFile"=path "C:/EC-Lab Development Package/Examples/Labview/V12/DefaultAging/Ch8_Device8_160513_14h_26m26s_JVmetrics.txt", "Status"=0.0, "ColorInd"=FALSE, "RunCont"=TRUE, "StatusStr"="stopped", "CopyToAll"=FALSE}, {"name"="Device9", "Channel"=8, "StartCh"=FALSE, "PauseCh"=FALSE, "StopCh"=FALSE, "ActiveArea cm2"=0.16, "AgingMode"=enum."MPP", "JVParameters"={"Hyst"=TRUE, "Start"=0.1, "End"=-0.2, "rate"=100.0, "record dE"=20.0, "equ t1"=1.0, "equ t2"=0.0, "vsInitEnd 2"=FALSE, "vsInitSt 3"=TRUE}, "AgingParams"={"Time"=30.0, "StepV"=0.01, "timetocheck"=5.0, "average over"=12.0}, "start time"=timestamp(0 s since 1904-01-01), "AgingFile"=path "", "JVFile"=path "", "JVMetricsFile"=path "", "Status"=0.0, "ColorInd"=FALSE, "RunCont"=TRUE, "StatusStr"="", "CopyToAll"=FALSE}, {"name"="Device10", "Channel"=9, "StartCh"=FALSE, "PauseCh"=FALSE, "StopCh"=FALSE, "ActiveArea cm2"=0.16, "AgingMode"=enum."MPP", "JVParameters"={"Hyst"=TRUE, "Start"=0.1, "End"=-0.2, "rate"=100.0, "record dE"=20.0, "equ t1"=1.0, "equ t2"=0.0, "vsInitEnd 2"=FALSE, "vsInitSt 3"=TRUE}, "AgingParams"={"Time"=30.0, "StepV"=0.01, "timetocheck"=5.0, "average over"=12.0}, "start time"=timestamp(0 s since 1904-01-01), "AgingFile"=path "", "JVFile"=path "", "JVMetricsFile"=path "", "Status"=0.0, "ColorInd"=FALSE, "RunCont"=TRUE, "StatusStr"="", "CopyToAll"=FALSE}, {"name"="Device11", "Channel"=10, "StartCh"=FALSE, "PauseCh"=FALSE, "StopCh"=FALSE, "ActiveArea cm2"=0.16, "AgingMode"=enum."MPP", "JVParameters"={"Hyst"=TRUE, "Start"=0.1, "End"=-0.2, "rate"=100.0, "record dE"=20.0, "equ t1"=1.0, "equ t2"=0.0, "vsInitEnd 2"=FALSE, "vsInitSt 3"=TRUE}, "AgingParams"={"Time"=30.0, "StepV"=0.01, "timetocheck"=5.0, "average over"=12.0}, "start time"=timestamp(0 s since 1904-01-01), "AgingFile"=path "", "JVFile"=path "", "JVMetricsFile"=path "", "Status"=0.0, "ColorInd"=FALSE, "RunCont"=TRUE, "StatusStr"="", "CopyToAll"=FALSE}, {"name"="Device12", "Channel"=11, "StartCh"=FALSE, "PauseCh"=FALSE, "StopCh"=FALSE, "ActiveArea cm2"=0.16, "AgingMode"=enum."MPP", "JVParameters"={"Hyst"=TRUE, "Start"=0.1, "End"=-0.2, "rate"=100.0, "record dE"=20.0, "equ t1"=1.0, "equ t2"=0.0, "vsInitEnd 2"=FALSE, "vsInitSt 3"=TRUE}, "AgingParams"={"Time"=30.0, "StepV"=0.01, "timetocheck"=5.0, "average over"=12.0}, "start time"=timestamp(0 s since 1904-01-01), "AgingFile"=path "", "JVFile"=path "", "JVMetricsFile"=path "", "Status"=0.0, "ColorInd"=FALSE, "RunCont"=TRUE, "StatusStr"="", "CopyToAll"=FALSE}, {"name"="Device13", "Channel"=12, "StartCh"=FALSE, "PauseCh"=FALSE, "StopCh"=FALSE, "ActiveArea cm2"=0.16, "AgingMode"=enum."MPP", "JVParameters"={"Hyst"=TRUE, "Start"=0.1, "End"=-0.2, "rate"=100.0, "record dE"=20.0, "equ t1"=1.0, "equ t2"=0.0, "vsInitEnd 2"=FALSE, "vsInitSt 3"=TRUE}, "AgingParams"={"Time"=30.0, "StepV"=0.01, "timetocheck"=5.0, "average over"=12.0}, "start time"=timestamp(0 s since 1904-01-01), "AgingFile"=path "", "JVFile"=path "", "JVMetricsFile"=path "", "Status"=0.0, "ColorInd"=FALSE, "RunCont"=TRUE, "StatusStr"="", "CopyToAll"=FALSE}, {"name"="Device14", "Channel"=13, "StartCh"=FALSE, "PauseCh"=FALSE, "StopCh"=FALSE, "ActiveArea cm2"=0.16, "AgingMode"=enum."MPP", "JVParameters"={"Hyst"=TRUE, "Start"=0.1, "End"=-0.2, "rate"=100.0, "record dE"=20.0, "equ t1"=1.0, "equ t2"=0.0, "vsInitEnd 2"=FALSE, "vsInitSt 3"=TRUE}, "AgingParams"={"Time"=30.0, "StepV"=0.01, "timetocheck"=5.0, "average over"=12.0}, "start time"=timestamp(0 s since 1904-01-01), "AgingFile"=path "", "JVFile"=path "", "JVMetricsFile"=path "", "Status"=0.0, "ColorInd"=FALSE, "RunCont"=TRUE, "StatusStr"="", "CopyToAll"=FALSE}, {"name"="Device15", "Channel"=14, "StartCh"=FALSE, "PauseCh"=FALSE, "StopCh"=FALSE, "ActiveArea cm2"=0.16, "AgingMode"=enum."MPP", "JVParameters"={"Hyst"=TRUE, "Start"=0.1, "End"=-0.2, "rate"=100.0, "record dE"=20.0, "equ t1"=1.0, "equ t2"=0.0, "vsInitEnd 2"=FALSE, "vsInitSt 3"=TRUE}, "AgingParams"={"Time"=30.0, "StepV"=0.01, "timetocheck"=5.0, "average over"=12.0}, "start time"=timestamp(0 s since 1904-01-01), "AgingFile"=path "", "JVFile"=path "", "JVMetricsFile"=path "", "Status"=0.0, "ColorInd"=FALSE, "RunCont"=TRUE, "StatusStr"="", "CopyToAll"=FALSE}, {"name"="Device16", "Channel"=15, "StartCh"=FALSE, "PauseCh"=FALSE, "StopCh"=FALSE, "ActiveArea cm2"=0.16, "AgingMode"=enum."MPP", "JVParameters"={"Hyst"=TRUE, "Start"=0.1, "End"=-0.2, "rate"=100.0, "record dE"=20.0, "equ t1"=1.0, "equ t2"=0.0, "vsInitEnd 2"=FALSE, "vsInitSt 3"=TRUE}, "AgingParams"={"Time"=30.0, "StepV"=0.01, "timetocheck"=5.0, "average over"=12.0}, "start time"=timestamp(0 s since 1904-01-01), "AgingFile"=path "", "JVFile"=path "", "JVMetricsFile"=path "", "Status"=0.0, "ColorInd"=FALSE, "RunCont"=TRUE, "StatusStr"="", "CopyToAll"=FALSE}] {"JVParameters"."End" min=-2.0 max=2.0; "JVParameters"."Start" min=-2.0 max=2.0; "Channel" items=["1", "2", "3", "4", "5", "6", "7", "8", "9", "10", "11", "12", "13", "14", "15", "16"]}
  in  "JVStandard":T12(array[cluster])=[{"name"="Device1", "Channel"=0, "StartCh"=FALSE, "PauseCh"=FALSE, "StopCh"=FALSE, "ActiveArea cm2"=0.16, "AgingMode"=enum."none", "JVParameters"={"Hyst"=TRUE, "Start"=0.1, "End"=-0.2, "rate"=10.0, "record dE"=10.0, "equ t1"=1.0, "equ t2"=0.0, "vsInitEnd 2"=FALSE, "vsInitSt 3"=TRUE}, "AgingParams"={"Time"=1.0, "StepV"=0.01, "timetocheck"=5.0, "average over"=4.0}, "start time"=timestamp(3545987186.527957 s since 1904-01-01), "AgingFile"=path "C:/EC-Lab Development Package/Examples/Labview/V12/DefaultAging/Ch1_Device1_160513_14h_26m26s_aging.txt", "JVFile"=path "C:/EC-Lab Development Package/Examples/Labview/V12/DefaultAging/Ch1_Device1_160513_14h_26m26s_JVs.txt", "JVMetricsFile"=path "C:/EC-Lab Development Package/Examples/Labview/V12/DefaultAging/Ch1_Device1_160513_14h_26m26s_JVmetrics.txt", "Status"=0.0, "ColorInd"=FALSE, "RunCont"=FALSE, "StatusStr"="stopped", "CopyToAll"=FALSE}, {"name"="Device2", "Channel"=1, "StartCh"=FALSE, "PauseCh"=FALSE, "StopCh"=FALSE, "ActiveArea cm2"=0.16, "AgingMode"=enum."none", "JVParameters"={"Hyst"=TRUE, "Start"=0.1, "End"=-0.2, "rate"=10.0, "record dE"=10.0, "equ t1"=1.0, "equ t2"=0.0, "vsInitEnd 2"=FALSE, "vsInitSt 3"=TRUE}, "AgingParams"={"Time"=1.0, "StepV"=0.01, "timetocheck"=5.0, "average over"=4.0}, "start time"=timestamp(3545986839.128179 s since 1904-01-01), "AgingFile"=path "C:/EC-Lab Development Package/Examples/Labview/V12/DefaultAging/Ch2_Device2_160513_14h_20m39s_aging.txt", "JVFile"=path "C:/EC-Lab Development Package/Examples/Labview/V12/DefaultAging/Ch2_Device2_160513_14h_20m39s_JVs.txt", "JVMetricsFile"=path "C:/EC-Lab Development Package/Examples/Labview/V12/DefaultAging/Ch2_Device2_160513_14h_20m39s_JVmetrics.txt", "Status"=0.0, "ColorInd"=FALSE, "RunCont"=FALSE, "StatusStr"="stopped", "CopyToAll"=FALSE}, {"name"="Device3", "Channel"=2, "StartCh"=FALSE, "PauseCh"=FALSE, "StopCh"=FALSE, "ActiveArea cm2"=0.16, "AgingMode"=enum."none", "JVParameters"={"Hyst"=TRUE, "Start"=0.1, "End"=-0.2, "rate"=10.0, "record dE"=10.0, "equ t1"=1.0, "equ t2"=0.0, "vsInitEnd 2"=FALSE, "vsInitSt 3"=TRUE}, "AgingParams"={"Time"=1.0, "StepV"=0.01, "timetocheck"=5.0, "average over"=4.0}, "start time"=timestamp(3545987186.5334716 s since 1904-01-01), "AgingFile"=path "C:/EC-Lab Development Package/Examples/Labview/V12/DefaultAging/Ch3_Device3_160513_14h_26m26s_aging.txt", "JVFile"=path "C:/EC-Lab Development Package/Examples/Labview/V12/DefaultAging/Ch3_Device3_160513_14h_26m26s_JVs.txt", "JVMetricsFile"=path "C:/EC-Lab Development Package/Examples/Labview/V12/DefaultAging/Ch3_Device3_160513_14h_26m26s_JVmetrics.txt", "Status"=0.0, "ColorInd"=FALSE, "RunCont"=FALSE, "StatusStr"="stopped", "CopyToAll"=FALSE}, {"name"="Device4", "Channel"=3, "StartCh"=FALSE, "PauseCh"=FALSE, "StopCh"=FALSE, "ActiveArea cm2"=0.16, "AgingMode"=enum."none", "JVParameters"={"Hyst"=TRUE, "Start"=0.1, "End"=-0.2, "rate"=10.0, "record dE"=10.0, "equ t1"=1.0, "equ t2"=0.0, "vsInitEnd 2"=FALSE, "vsInitSt 3"=TRUE}, "AgingParams"={"Time"=1.0, "StepV"=0.01, "timetocheck"=5.0, "average over"=4.0}, "start time"=timestamp(3545987186.5364795 s since 1904-01-01), "AgingFile"=path "C:/EC-Lab Development Package/Examples/Labview/V12/DefaultAging/Ch4_Device4_160513_14h_26m26s_aging.txt", "JVFile"=path "C:/EC-Lab Development Package/Examples/Labview/V12/DefaultAging/Ch4_Device4_160513_14h_26m26s_JVs.txt", "JVMetricsFile"=path "C:/EC-Lab Development Package/Examples/Labview/V12/DefaultAging/Ch4_Device4_160513_14h_26m26s_JVmetrics.txt", "Status"=0.0, "ColorInd"=FALSE, "RunCont"=FALSE, "StatusStr"="stopped", "CopyToAll"=FALSE}, {"name"="Device5", "Channel"=4, "StartCh"=FALSE, "PauseCh"=FALSE, "StopCh"=FALSE, "ActiveArea cm2"=0.16, "AgingMode"=enum."none", "JVParameters"={"Hyst"=TRUE, "Start"=0.1, "End"=-0.2, "rate"=10.0, "record dE"=10.0, "equ t1"=1.0, "equ t2"=0.0, "vsInitEnd 2"=FALSE, "vsInitSt 3"=TRUE}, "AgingParams"={"Time"=1.0, "StepV"=0.01, "timetocheck"=5.0, "average over"=4.0}, "start time"=timestamp(3545987186.537483 s since 1904-01-01), "AgingFile"=path "C:/EC-Lab Development Package/Examples/Labview/V12/DefaultAging/Ch5_Device5_160513_14h_26m26s_aging.txt", "JVFile"=path "C:/EC-Lab Development Package/Examples/Labview/V12/DefaultAging/Ch5_Device5_160513_14h_26m26s_JVs.txt", "JVMetricsFile"=path "C:/EC-Lab Development Package/Examples/Labview/V12/DefaultAging/Ch5_Device5_160513_14h_26m26s_JVmetrics.txt", "Status"=0.0, "ColorInd"=FALSE, "RunCont"=FALSE, "StatusStr"="stopped", "CopyToAll"=FALSE}, {"name"="Device6", "Channel"=5, "StartCh"=FALSE, "PauseCh"=FALSE, "StopCh"=FALSE, "ActiveArea cm2"=0.16, "AgingMode"=enum."none", "JVParameters"={"Hyst"=TRUE, "Start"=0.1, "End"=-0.2, "rate"=10.0, "record dE"=10.0, "equ t1"=1.0, "equ t2"=0.0, "vsInitEnd 2"=FALSE, "vsInitSt 3"=TRUE}, "AgingParams"={"Time"=1.0, "StepV"=0.01, "timetocheck"=5.0, "average over"=4.0}, "start time"=timestamp(3545987186.5399885 s since 1904-01-01), "AgingFile"=path "C:/EC-Lab Development Package/Examples/Labview/V12/DefaultAging/Ch6_Device6_160513_14h_26m26s_aging.txt", "JVFile"=path "C:/EC-Lab Development Package/Examples/Labview/V12/DefaultAging/Ch6_Device6_160513_14h_26m26s_JVs.txt", "JVMetricsFile"=path "C:/EC-Lab Development Package/Examples/Labview/V12/DefaultAging/Ch6_Device6_160513_14h_26m26s_JVmetrics.txt", "Status"=0.0, "ColorInd"=FALSE, "RunCont"=FALSE, "StatusStr"="stopped", "CopyToAll"=FALSE}, {"name"="Device7", "Channel"=6, "StartCh"=FALSE, "PauseCh"=FALSE, "StopCh"=FALSE, "ActiveArea cm2"=0.16, "AgingMode"=enum."none", "JVParameters"={"Hyst"=TRUE, "Start"=0.1, "End"=-0.2, "rate"=10.0, "record dE"=10.0, "equ t1"=1.0, "equ t2"=0.0, "vsInitEnd 2"=FALSE, "vsInitSt 3"=TRUE}, "AgingParams"={"Time"=1.0, "StepV"=0.01, "timetocheck"=5.0, "average over"=4.0}, "start time"=timestamp(3545987186.5446434 s since 1904-01-01), "AgingFile"=path "C:/EC-Lab Development Package/Examples/Labview/V12/DefaultAging/Ch7_Device7_160513_14h_26m26s_aging.txt", "JVFile"=path "C:/EC-Lab Development Package/Examples/Labview/V12/DefaultAging/Ch7_Device7_160513_14h_26m26s_JVs.txt", "JVMetricsFile"=path "C:/EC-Lab Development Package/Examples/Labview/V12/DefaultAging/Ch7_Device7_160513_14h_26m26s_JVmetrics.txt", "Status"=0.0, "ColorInd"=FALSE, "RunCont"=FALSE, "StatusStr"="stopped", "CopyToAll"=FALSE}, {"name"="Device8", "Channel"=7, "StartCh"=FALSE, "PauseCh"=FALSE, "StopCh"=FALSE, "ActiveArea cm2"=0.16, "AgingMode"=enum."none", "JVParameters"={"Hyst"=TRUE, "Start"=0.1, "End"=-0.2, "rate"=10.0, "record dE"=10.0, "equ t1"=1.0, "equ t2"=0.0, "vsInitEnd 2"=FALSE, "vsInitSt 3"=TRUE}, "AgingParams"={"Time"=1.0, "StepV"=0.01, "timetocheck"=5.0, "average over"=4.0}, "start time"=timestamp(3545987186.5466247 s since 1904-01-01), "AgingFile"=path "C:/EC-Lab Development Package/Examples/Labview/V12/DefaultAging/Ch8_Device8_160513_14h_26m26s_aging.txt", "JVFile"=path "C:/EC-Lab Development Package/Examples/Labview/V12/DefaultAging/Ch8_Device8_160513_14h_26m26s_JVs.txt", "JVMetricsFile"=path "C:/EC-Lab Development Package/Examples/Labview/V12/DefaultAging/Ch8_Device8_160513_14h_26m26s_JVmetrics.txt", "Status"=0.0, "ColorInd"=FALSE, "RunCont"=FALSE, "StatusStr"="stopped", "CopyToAll"=FALSE}, {"name"="Device9", "Channel"=8, "StartCh"=FALSE, "PauseCh"=FALSE, "StopCh"=FALSE, "ActiveArea cm2"=0.16, "AgingMode"=enum."none", "JVParameters"={"Hyst"=TRUE, "Start"=0.1, "End"=-0.2, "rate"=10.0, "record dE"=10.0, "equ t1"=1.0, "equ t2"=0.0, "vsInitEnd 2"=FALSE, "vsInitSt 3"=TRUE}, "AgingParams"={"Time"=0.0, "StepV"=0.0, "timetocheck"=0.0, "average over"=0.0}, "start time"=timestamp(0 s since 1904-01-01), "AgingFile"=path "", "JVFile"=path "", "JVMetricsFile"=path "", "Status"=0.0, "ColorInd"=FALSE, "RunCont"=FALSE, "StatusStr"="", "CopyToAll"=FALSE}, {"name"="Device10", "Channel"=9, "StartCh"=FALSE, "PauseCh"=FALSE, "StopCh"=FALSE, "ActiveArea cm2"=0.16, "AgingMode"=enum."none", "JVParameters"={"Hyst"=TRUE, "Start"=0.1, "End"=-0.2, "rate"=10.0, "record dE"=10.0, "equ t1"=1.0, "equ t2"=0.0, "vsInitEnd 2"=FALSE, "vsInitSt 3"=TRUE}, "AgingParams"={"Time"=0.0, "StepV"=0.0, "timetocheck"=0.0, "average over"=0.0}, "start time"=timestamp(0 s since 1904-01-01), "AgingFile"=path "", "JVFile"=path "", "JVMetricsFile"=path "", "Status"=0.0, "ColorInd"=FALSE, "RunCont"=FALSE, "StatusStr"="", "CopyToAll"=FALSE}, {"name"="Device11", "Channel"=10, "StartCh"=FALSE, "PauseCh"=FALSE, "StopCh"=FALSE, "ActiveArea cm2"=0.16, "AgingMode"=enum."none", "JVParameters"={"Hyst"=TRUE, "Start"=0.1, "End"=-0.2, "rate"=10.0, "record dE"=10.0, "equ t1"=1.0, "equ t2"=0.0, "vsInitEnd 2"=FALSE, "vsInitSt 3"=TRUE}, "AgingParams"={"Time"=0.0, "StepV"=0.0, "timetocheck"=0.0, "average over"=0.0}, "start time"=timestamp(0 s since 1904-01-01), "AgingFile"=path "", "JVFile"=path "", "JVMetricsFile"=path "", "Status"=0.0, "ColorInd"=FALSE, "RunCont"=FALSE, "StatusStr"="", "CopyToAll"=FALSE}, {"name"="Device12", "Channel"=11, "StartCh"=FALSE, "PauseCh"=FALSE, "StopCh"=FALSE, "ActiveArea cm2"=0.16, "AgingMode"=enum."none", "JVParameters"={"Hyst"=TRUE, "Start"=0.1, "End"=-0.2, "rate"=10.0, "record dE"=10.0, "equ t1"=1.0, "equ t2"=0.0, "vsInitEnd 2"=FALSE, "vsInitSt 3"=TRUE}, "AgingParams"={"Time"=0.0, "StepV"=0.0, "timetocheck"=0.0, "average over"=0.0}, "start time"=timestamp(0 s since 1904-01-01), "AgingFile"=path "", "JVFile"=path "", "JVMetricsFile"=path "", "Status"=0.0, "ColorInd"=FALSE, "RunCont"=FALSE, "StatusStr"="", "CopyToAll"=FALSE}, {"name"="Device13", "Channel"=12, "StartCh"=FALSE, "PauseCh"=FALSE, "StopCh"=FALSE, "ActiveArea cm2"=0.16, "AgingMode"=enum."none", "JVParameters"={"Hyst"=TRUE, "Start"=0.1, "End"=-0.2, "rate"=10.0, "record dE"=10.0, "equ t1"=1.0, "equ t2"=0.0, "vsInitEnd 2"=FALSE, "vsInitSt 3"=TRUE}, "AgingParams"={"Time"=0.0, "StepV"=0.0, "timetocheck"=0.0, "average over"=0.0}, "start time"=timestamp(0 s since 1904-01-01), "AgingFile"=path "", "JVFile"=path "", "JVMetricsFile"=path "", "Status"=0.0, "ColorInd"=FALSE, "RunCont"=FALSE, "StatusStr"="", "CopyToAll"=FALSE}, {"name"="Device14", "Channel"=13, "StartCh"=FALSE, "PauseCh"=FALSE, "StopCh"=FALSE, "ActiveArea cm2"=0.16, "AgingMode"=enum."none", "JVParameters"={"Hyst"=TRUE, "Start"=0.1, "End"=-0.2, "rate"=10.0, "record dE"=10.0, "equ t1"=1.0, "equ t2"=0.0, "vsInitEnd 2"=FALSE, "vsInitSt 3"=TRUE}, "AgingParams"={"Time"=0.0, "StepV"=0.0, "timetocheck"=0.0, "average over"=0.0}, "start time"=timestamp(0 s since 1904-01-01), "AgingFile"=path "", "JVFile"=path "", "JVMetricsFile"=path "", "Status"=0.0, "ColorInd"=FALSE, "RunCont"=FALSE, "StatusStr"="", "CopyToAll"=FALSE}, {"name"="Device15", "Channel"=14, "StartCh"=FALSE, "PauseCh"=FALSE, "StopCh"=FALSE, "ActiveArea cm2"=0.16, "AgingMode"=enum."none", "JVParameters"={"Hyst"=TRUE, "Start"=0.1, "End"=-0.2, "rate"=10.0, "record dE"=10.0, "equ t1"=1.0, "equ t2"=0.0, "vsInitEnd 2"=FALSE, "vsInitSt 3"=TRUE}, "AgingParams"={"Time"=0.0, "StepV"=0.0, "timetocheck"=0.0, "average over"=0.0}, "start time"=timestamp(0 s since 1904-01-01), "AgingFile"=path "", "JVFile"=path "", "JVMetricsFile"=path "", "Status"=0.0, "ColorInd"=FALSE, "RunCont"=FALSE, "StatusStr"="", "CopyToAll"=FALSE}, {"name"="Device16", "Channel"=15, "StartCh"=FALSE, "PauseCh"=FALSE, "StopCh"=FALSE, "ActiveArea cm2"=0.16, "AgingMode"=enum."none", "JVParameters"={"Hyst"=TRUE, "Start"=0.1, "End"=-0.2, "rate"=10.0, "record dE"=10.0, "equ t1"=1.0, "equ t2"=0.0, "vsInitEnd 2"=FALSE, "vsInitSt 3"=TRUE}, "AgingParams"={"Time"=0.0, "StepV"=0.0, "timetocheck"=0.0, "average over"=0.0}, "start time"=timestamp(0 s since 1904-01-01), "AgingFile"=path "", "JVFile"=path "", "JVMetricsFile"=path "", "Status"=0.0, "ColorInd"=FALSE, "RunCont"=FALSE, "StatusStr"="", "CopyToAll"=FALSE}] {"JVParameters"."End" min=-2.0 max=2.0; "JVParameters"."Start" min=-2.0 max=2.0; "Channel" items=["1", "2", "3", "4", "5", "6", "7", "8", "9", "10", "11", "12", "13", "14", "15", "16"]}
  in  "HeaderJVMetrics":string[](array[string])=["time (h)", "1st: Voc (V)", "Jsc (mA/cm2)", "FF", "P (mW/cm2)", "VMPP (V)", "JMPP (mA/cm2)", "Hyst P1/P2", "2nd: Voc (V)", "Jsc (mA/cm2)", "FF", "P (mW/cm2)", "VMPP (V)", "JMPP (mA/cm2)", "scan rate (mV/s)", "intensity (suns)", "temperature (C)"]
  in  "NoOfChannels":i32=16
  in  "HeaderAging":string[](array[string])=["time (h)", "P (mW/cm2)", "V (V)", "J (mA/cm2)", "intensity (suns)", "temperature (C)"]
  in  "VoltageRange abs and vs Voc":dbl[][](array[numeric])=[[-1.0, -2.0], [1.7, 0.2]]
  in  "autosave file":path=path "C:/EC-Lab Development Package/Examples/Labview/V12/AUTOSAVE.DAT"
  in  "Autosave every minutes":u32=1
  in  "device area (cm2)":dbl=0.16 caption="Time Target (s)"
  out "Device Code":i32=22
  out "Exit 2":bool=TRUE
  # "JV parameters                                                               rest time\nStart V               End V          Scan Rate     Step        -->         <--   Hysteresis\n     V     vs OC      V  vs. OC       mV/s        mV            s              s"
  # "Aging Parameters\n   Time       V (Step) / J   Update    Average\n    min      V (mA/cm2)        s            over"
  # "run \ncontinuously?"
  # "AgingMode"
  # "start time"
  # "status"
  # "Device Name"
  # "Channel"
  # "Area cm2"
  # "Holder 3"
  # "Holder 4"
  # "Remember to export your aging data to Excel!"
  # "All Channels"
  # "Hardware by Konrad Domanski\nSoftware by Wolfgang Tress"
  # "time     -->    Voc         Jsc              FF             P          Hyst   <-- Voc           Jsc             FF        Power        \nhours               V         mA/cm2                mW/cm2  P1/P2          V        mA/cm2                mW/cm2"
  # "Last JV Curve"
  # "Last Aging Track"
  # "--> Voc           Jsc            FF            P          Hyst   <-- Voc        Jsc           FF            P     scan rate intensity temperature\n         V         mA/cm2               mW/cm2 P1/P2         V        mA/cm2               mW/cm2   mV/s      suns         C"
  # "Default Values"
  # "JV limits"
  # "Plot legends"
  # "min value\n\nmax value"
  # "absolute         vs. init"
  # "File headers"
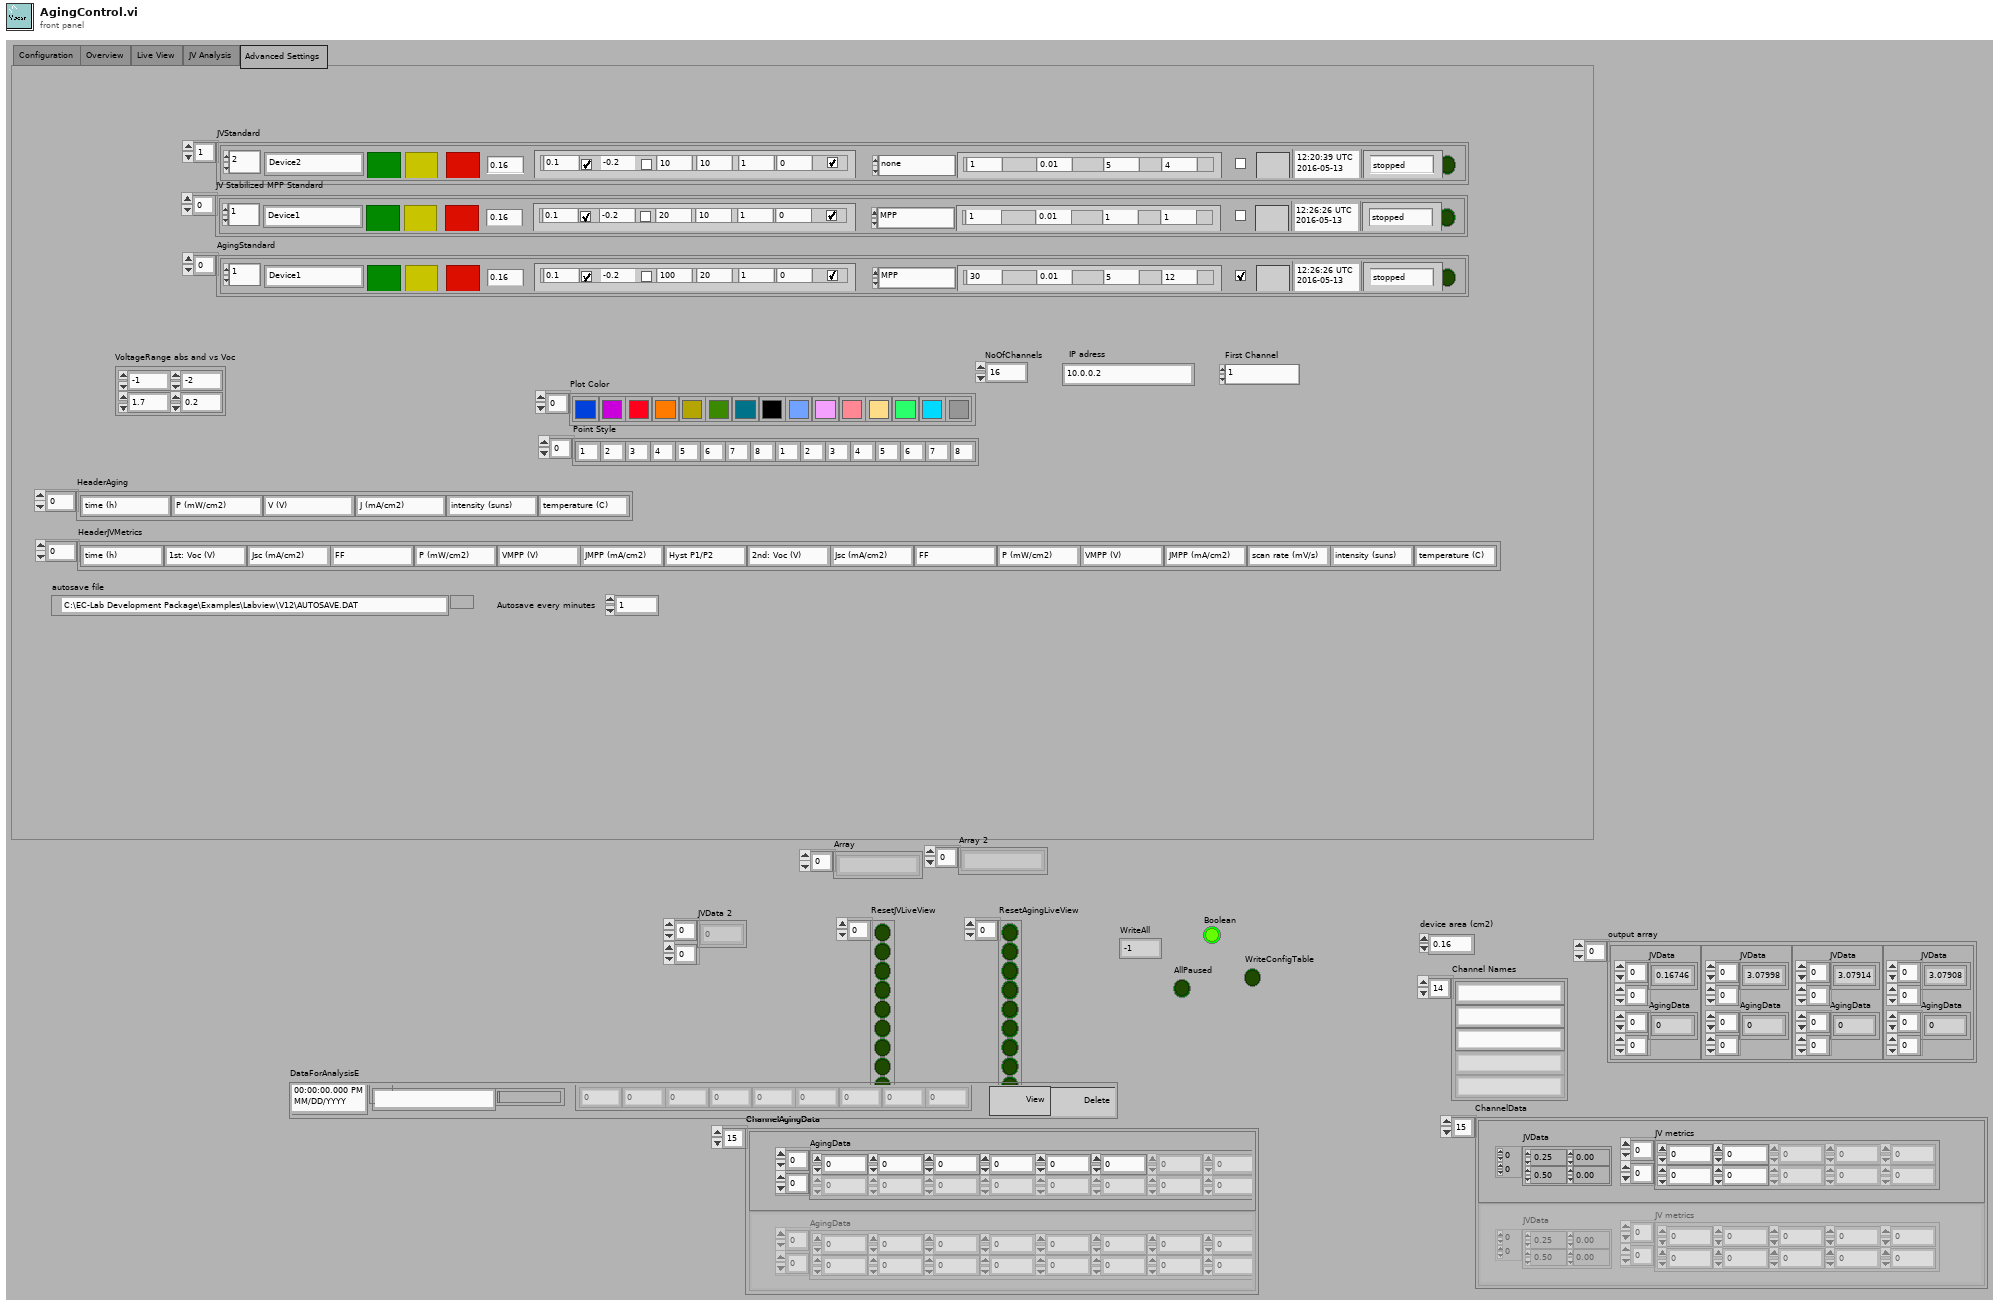
[diagram p1: front panel]
types:
  T1 = cluster{"JVData":dbl[][], "JVmetrics":dbl[], "TransientData":dbl[][], "TimeMeasured":timestamp, "Name":string, "Delete":bool, "Eff":u8, "ViewJV":bool}
  T2 = cluster{"JV metrics":sgl[][], "JVData":sgl[][]}[]
  T3 = enum32{"Configuration", "Overview", "Live View", "JV Analysis", "Advanced Settings"}
  T4 = cluster{"name":string, "Channel":u8, "StartCh":bool, "PauseCh":bool, "StopCh":bool, "ActiveArea cm2":dbl, "AgingMode":enum16{"MPP", "Voc", "Fixed Voltage", "Fixed Current", "none"}, "JVParameters":cluster{"Hyst":bool, "Start":dbl, "End":dbl, "rate":dbl, "record dE":dbl, "equ t1":dbl, "equ t2":dbl, "vsInitEnd 2":bool, "vsInitSt 3":bool}, "AgingParams":cluster{"Time":dbl, "StepV":dbl, "timetocheck":dbl, "average over":dbl}, "start time":timestamp, "AgingFile":path, "JVFile":path, "JVMetricsFile":path, "Status":dbl, "ColorInd":bool, "RunCont":bool, "StatusStr":string, "CopyToAll":bool}[]
  T5 = cluster{"JV metrics":sgl[], "JV metrics":sgl[]}[]
  T6 = enum16{"J(V)", "-J(V)", "abs J(V)", "P(V)", "-P(V)", "V(t)", "I(t)"}
  T7 = enum16{"t h", "P mW/cm2", "V V", "J mA/cm2", "Int suns", "Temp C"}
  T8 = cluster{"ExchangeJVData":sgl[], "ExchangeJVData":dbl[]}
  T9 = cluster{"ExchangeCAData":sgl[], "ExchangeCAData":dbl[]}
  T10 = cluster{"JVData":dbl[][], "JVmetrics":dbl[], "TransientData":dbl[][], "TimeMeasured":timestamp, "Name":string, "Delete":bool, "Eff":u8, "ViewJV":bool}[]
  T11 = cluster{"TransientData":dbl[], "TransientData":dbl[]}[]
  T12 = cluster{"name":string, "Channel":u8, "StartCh":bool, "PauseCh":bool, "StopCh":bool, "ActiveArea cm2":dbl, "AgingMode":enum16{"MPP", "Voc", "fixed Voltage", "fixed Current", "none"}, "JVParameters":cluster{"Hyst":bool, "Start":dbl, "End":dbl, "rate":dbl, "record dE":dbl, "equ t1":dbl, "equ t2":dbl, "vsInitEnd 2":bool, "vsInitSt 3":bool}, "AgingParams":cluster{"Time":dbl, "StepV":dbl, "timetocheck":dbl, "average over":dbl}, "start time":timestamp, "AgingFile":path, "JVFile":path, "JVMetricsFile":path, "Status":dbl, "ColorInd":bool, "RunCont":bool, "StatusStr":string, "CopyToAll":bool}[]
  T13 = cluster{"TransientData":dbl[], "TransientData":dbl[]}
  T14 = cluster{"name":string, "Channel":u8, "StartCh":bool, "PauseCh":bool, "StopCh":bool, "ActiveArea cm2":dbl, "AgingMode":enum16{"MPP", "Voc", "Fixed Voltage", "Fixed Current", "none"}, "JVParameters":cluster{"Hyst":bool, "Start":dbl, "End":dbl, "rate":dbl, "record dE":dbl, "equ t1":dbl, "equ t2":dbl, "vsInitEnd 2":bool, "vsInitSt 3":bool}, "AgingParams":cluster{"Time":dbl, "StepV":dbl, "timetocheck":dbl, "average over":dbl}, "start time":timestamp, "AgingFile":path, "JVFile":path, "JVMetricsFile":path, "Status":dbl, "ColorInd":bool, "RunCont":bool, "StatusStr":string, "CopyToAll":bool}
  T15 = cluster{"Channel":i32, "BoardVersion":i32, "BoardSerialCode":i32, "FirmwareCode":i32, "FirmwareVersion":i32, "XilinxVersion":i32, "AmpCode":i32, "NbAmp":i32, "LcBoard":i32, "Zboard":i32, "MuxBoard":i32, "GPRAboard":i32, "MemSize":i32, "MemFilled":i32, "state":i32, "MaxIRange":i32, "MinIRange":i32, "MaxBandwidth":i32, "NbOfTechniques":i32}
  T16 = enum16{"MPP", "Voc", "Fixed Voltage", "Fixed Current", "none"}
  T17 = cluster{"Hyst":bool, "Start":dbl, "End":dbl, "rate":dbl, "record dE":dbl, "equ t1":dbl, "equ t2":dbl, "vsInitEnd 2":bool, "vsInitSt 3":bool}
  T18 = cluster{"Time":dbl, "StepV":dbl, "timetocheck":dbl, "average over":dbl}
  T19 = enum16{"open", "replace", "create", "open or create", "replace or create", "replace or create with confirmation"}
  T20 = cluster{"name":string, "Channel":u8, "StartCh":bool, "PauseCh":bool, "StopCh":bool, "ActiveArea cm2":dbl, "AgingMode":u16, "JVParameters":cluster{"Hyst":bool, "Start":dbl, "End":dbl, "rate":dbl, "record dE":dbl, "equ t1":dbl, "equ t2":dbl, "vsInitEnd 2":bool, "vsInitSt 3":bool}, "AgingParams":cluster{"Time":dbl, "StepV":dbl, "timetocheck":dbl, "average over":dbl}, "start time":timestamp, "AgingFile":path, "JVFile":path, "JVMetricsFile":path, "Status":dbl, "ColorInd":bool, "RunCont":bool, "StatusStr":string, "CopyToAll":bool}[]
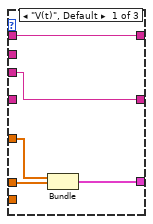
[diagram p10: hidden frame]
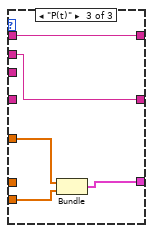
[diagram p11: hidden frame]
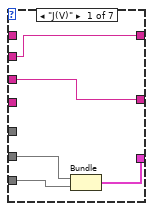
[diagram p12: hidden frame]
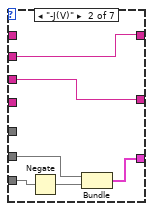
[diagram p13: hidden frame]
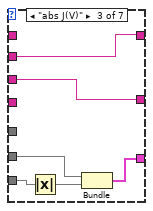
[diagram p14: hidden frame]
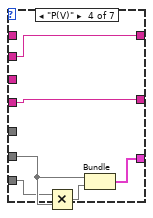
[diagram p15: hidden frame]
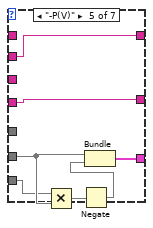
[diagram p16: hidden frame]
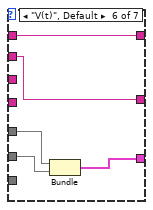
[diagram p17: hidden frame]
diagram:
  w37 = FALSE ("Exit 2")
  # "Channel Control and Live View"
  # "Aging Procedure"
  # "Overview Graphs"
  n1 = while {
    stop <- w164 stop-if-true
    w99 = 1 ("index (row)")
    w39 = 0 ("index (row)")
    n2 = local read "ChannelData"() -> (w153:T2)
    n3 = local read "LiveViewData"() -> (w163:cluster{"JVData":sgl[][], "AgingData":sgl[][]}[])
    n4 = for {
      tunnel: w163 -> [w179] mode=indexing
      tunnel: [w175] -> w111 mode=indexing
      tunnel: w153 -> [w172] mode=indexing
      tunnel: [w165] -> w110 mode=indexing
      tunnel: [w166] -> w109 mode=indexing
      n5 = Unbundle By Name(w172) -> ("JV metrics"=w171:sgl[][])
      n6 = Unbundle By Name(w179) -> ("AgingData"=w177:sgl[][])
      n7 = Index Array(array=w171, index (col)=4 ("disabled index (col)")) -> (element=w168:sgl[])  [unwired: 1 in]
      n8 = Array Size(array=w177) -> (size(s)=w176:i32[])
      n9 = Array Size(array=w168) -> (size(s)=w169:i32)
      n10 = Array Max & Min(array=w168) -> (max value=w165:sgl)  [unwired: 3 out]
      n11 = Index Array(array=w176) -> (element=w174:i32)  [unwired: 1 in]
      n12 = Decrement(x=w169) -> (x-1=w167:i32)
      n13 = Decrement(x=w174) -> (x-1=w173:i32)
      n14 = Index Array(array=w177, index (row)=w173, index (col)=1 ("disabled index (col)")) -> (element=w175:sgl)
      n15 = Index Array(array=w168, index=w167) -> (element=w166:sgl)
    }
    n16 = Index Array(array=w109) -> (element #1=→"Tank 1":sgl, element #2=→"Tank 2":sgl, element #3=→"Tank 3":sgl, element #4=→"Tank 4":sgl, element #5=→"Tank 5":sgl, element #6=→"Tank 6":sgl, element #7=→"Tank 7":sgl, element #8=→"Tank 8":sgl, element #9=→"Tank 9":sgl, element #10=→"Tank 10":sgl, element #11=→"Tank 11":sgl, element #12=→"Tank 12":sgl, element #13=→"Tank 13":sgl, element #14=→"Tank 14":sgl, element #15=→"Tank 15":sgl, element #16=→"Tank 16":sgl)  [unwired: 16 in]
    n17 = Wait Until Next ms Multiple(millisecond multiple=u32 300) -> ()  [unwired: 1 out]
    n18 = global read "ActiveArray.vi" "Active"() -> (w112:bool[])
    n19 = local read "Exit"() -> (w164:bool)
    n20 = Index Array(array=w112) -> (element #1=w120:bool, element #2=w119:bool, element #3=w118:bool, element #4=w117:bool, element #5=w116:bool, element #6=w115:bool, element #7=w114:bool, element #8=w113:bool, element #9=w66:bool, element #10=w65:bool, element #11=w64:bool, element #12=w63:bool, element #13=w62:bool, element #14=w61:bool, element #15=w60:bool, element #16=w59:bool)  [unwired: 16 in]
    "Active 1" <- w120
    "Active 2" <- w119
    "Active 3" <- w118
    "Active 4" <- w117
    "Active 5" <- w116
    "Active 6" <- w115
    "Active 7" <- w114
    "Active 8" <- w113
    "Active 16" <- w59
    "Active 15" <- w60
    "Active 14" <- w61
    "Active 13" <- w62
    "Active 12" <- w63
    "Active 11" <- w64
    "Active 10" <- w65
    "Active 9" <- w66
    n21 = control-ref of="Tank 13"() -> (w46:refnum<vi>)
    n22 = control-ref of="Tank 15"() -> (w44:refnum<vi>)
    n23 = control-ref of="Tank 11"() -> (w48:refnum<vi>)
    n24 = control-ref of="Tank 9"() -> (w50:refnum<vi>)
    n25 = Index Array(array=w110) -> (element #1=w143:sgl, element #2=w139:sgl, element #3=w127:sgl, element #4=w126:sgl, element #5=w124:sgl, element #6=w123:sgl, element #7=w122:sgl, element #8=w121:sgl, element #9=w58:sgl, element #10=w57:sgl, element #11=w56:sgl, element #12=w55:sgl, element #13=w54:sgl, element #14=w53:sgl, element #15=w52:sgl, element #16=w51:sgl)  [unwired: 16 in]
    n26 = property class="Slide (strict)"(reference=w46, "Scale.Maximum"=w54, "Scale.Minimum"=0.0 ("Scale.Range:Minimum"), "Visible"=w62) -> ()  [unwired: 1 in, 2 out]
    n27 = property class="Slide (strict)"(reference=w44, "Scale.Maximum"=w52, "Scale.Minimum"=0.0 ("Scale.Range:Minimum"), "Visible"=w60) -> ()  [unwired: 1 in, 2 out]
    n28 = property class="Slide (strict)"(reference=w48, "Scale.Maximum"=w56, "Scale.Minimum"=0.0 ("Scale.Range:Minimum"), "Visible"=w64) -> ()  [unwired: 1 in, 2 out]
    n29 = property class="Slide (strict)"(reference=w50, "Scale.Maximum"=w58, "Scale.Minimum"=0.0 ("Scale.Range:Minimum"), "Visible"=w66) -> ()  [unwired: 1 in, 2 out]
    n30 = control-ref of="Tank 1"() -> (w144:refnum<vi>)
    n31 = property class="Slide (strict)"(reference=w144, "Scale.Maximum"=w143, "Scale.Minimum"=0.0 ("Scale.Range:Minimum"), "Visible"=w120) -> ()  [unwired: 1 in, 2 out]
    n32 = control-ref of="Tank 3"() -> (w135:refnum<vi>)
    n33 = control-ref of="Tank 4"() -> (w134:refnum<vi>)
    n34 = control-ref of="Tank 7"() -> (w129:refnum<vi>)
    n35 = control-ref of="Tank 12"() -> (w47:refnum<vi>)
    n36 = control-ref of="Tank 14"() -> (w45:refnum<vi>)
    n37 = control-ref of="Tank 16"() -> (w43:refnum<vi>)
    n38 = control-ref of="Tank 10"() -> (w49:refnum<vi>)
    n39 = property class="Slide (strict)"(reference=w135, "Scale.Maximum"=w127, "Scale.Minimum"=0.0 ("Scale.Range:Minimum"), "Visible"=w118) -> ()  [unwired: 1 in, 2 out]
    n40 = property class="Slide (strict)"(reference=w134, "Scale.Maximum"=w126, "Scale.Minimum"=0.0 ("Scale.Range:Minimum"), "Visible"=w117) -> ()  [unwired: 1 in, 2 out]
    n41 = property class="Slide (strict)"(reference=w129, "Scale.Maximum"=w122, "Scale.Minimum"=0.0 ("Scale.Range:Minimum"), "Visible"=w114) -> ()  [unwired: 1 in, 2 out]
    n42 = control-ref of="Tank 2"() -> (w141:refnum<vi>)
    n43 = property class="Slide (strict)"(reference=w141, "Scale.Maximum"=w139, "Scale.Minimum"=0.0 ("Scale.Range:Minimum"), "Visible"=w119) -> ()  [unwired: 1 in, 2 out]
    n44 = property class="Slide (strict)"(reference=w49, "Scale.Maximum"=w57, "Scale.Minimum"=0.0 ("Scale.Range:Minimum"), "Visible"=w65) -> ()  [unwired: 1 in, 2 out]
    n45 = property class="Slide (strict)"(reference=w47, "Scale.Maximum"=w55, "Scale.Minimum"=0.0 ("Scale.Range:Minimum"), "Visible"=w63) -> ()  [unwired: 1 in, 2 out]
    n46 = property class="Slide (strict)"(reference=w45, "Scale.Maximum"=w53, "Scale.Minimum"=0.0 ("Scale.Range:Minimum"), "Visible"=w61) -> ()  [unwired: 1 in, 2 out]
    n47 = property class="Slide (strict)"(reference=w43, "Scale.Maximum"=w51, "Scale.Minimum"=0.0 ("Scale.Range:Minimum"), "Visible"=w59) -> ()  [unwired: 1 in, 2 out]
    n48 = control-ref of="Tank 5"() -> (w133:refnum<vi>)
    n49 = control-ref of="Tank 6"() -> (w125:refnum<vi>)
    n50 = control-ref of="Tank 8"() -> (w128:refnum<vi>)
    n51 = property class="Slide (strict)"(reference=w133, "Scale.Maximum"=w124, "Scale.Minimum"=0.0 ("Scale.Range:Minimum"), "Visible"=w116) -> ()  [unwired: 1 in, 2 out]
    n52 = property class="Slide (strict)"(reference=w128, "Scale.Maximum"=w121, "Scale.Minimum"=0.0 ("Scale.Range:Minimum"), "Visible"=w113) -> ()  [unwired: 1 in, 2 out]
    n53 = property class="Slide (strict)"(reference=w125, "Scale.Maximum"=w123, "Scale.Minimum"=0.0 ("Scale.Range:Minimum"), "Visible"=w115) -> ()  [unwired: 1 in, 2 out]
    n54 = Build Array(w111, w110, w109) -> (w108:sgl[][])
    n55 = global read "IntensityTemperature.vi" "IntTemp"() -> (w107:dbl[][])
    n56 = Index Array(array=w111) -> (element #1=→"Voc 1":sgl, element #2=→"Voc 2":sgl, element #3=→"Voc 3":sgl, element #4=→"Voc 4":sgl, element #5=→"Voc 5":sgl, element #6=→"Voc 6":sgl, element #7=→"Voc 7":sgl, element #8=→"Voc 8":sgl, element #9=→"Voc 9":sgl, element #10=→"Voc 10":sgl, element #11=→"Voc 11":sgl, element #12=→"Voc 12":sgl, element #13=→"Voc 13":sgl, element #14=→"Voc 14":sgl, element #15=→"Voc 15":sgl, element #16=→"Voc 16":sgl)  [unwired: 16 in]
    n57 = global write "AgingStatus.vi" "StatusVJV"(w108) -> ()
    n58 = Index Array(array=w107, index (row) #1=w39, index (col) #1=w39, index (row) #2=w99, index (col) #2=w39, index (row) #3=w99, index (col) #3=2 ("index (row)"), index (row) #4=w99, index (col) #4=4 ("index (row)"), index (row) #5=w99, index (col) #5=6 ("index (row)"), index (row) #6=w39, index (col) #6=8 ("disabled index (col)"), index (row) #7=w99, index (col) #7=8 ("disabled index (col)"), index (row) #8=w99, index (col) #8=10 ("disabled index (col)"), index (row) #9=w99, index (col) #9=12 ("disabled index (col)"), index (row) #10=w99, index (col) #10=14 ("disabled index (col)")) -> (element #1=→"IntA" →"IntBar A 1":dbl, element #2=→"T12":dbl, element #3=→"T34":dbl, element #4=→"T56":dbl, element #5=→"T78":dbl, element #6=→"IntA 2" →"IntBar A 2":dbl, element #7=→"T12 2":dbl, element #8=→"T34 2":dbl, element #9=→"T56 2":dbl, element #10=→"T78 2":dbl)
  }
  n59 = local write "DataForAnalysis"(T10 [] ("DataForAnalysis")) -> ()
  n60 = for {
    N: "NoOfChannels" -> [_]
    tunnel: [w190] -> w11 mode=indexing
    tunnel: "AgingData" ("name (unnamed)") -> [w189]
    tunnel: "LiveViewAgingData" ("name (unnamed)") -> [w188]
    tunnel: "LiveViewJVData" ("name (unnamed)") -> [w183]
    tunnel: [w182] -> w21 mode=indexing
    tunnel: [w181] -> w7 mode=indexing
    i -> [w191]
    w185 = sgl[][] [[0.100549996, 1.4351095e-06, 1.050421, 1.0], [0.20105, 9.236625e-07, 1.0001758, 1.0], [0.30155, 6.189802e-07, 0.9500262, 1.0], [0.40199998, 4.1734597e-07, 0.8998193, 1.0], [0.5025, 2.727543e-07, 0.84953594, 1.0], [0.60295, 1.5926109e-07, 0.79927176, 1.0], [0.70344996, 6.1173935e-08, 0.74896926, 1.0], [0.80394995, -3.2675118e-08, 0.6988388, 1.0], [0.9044, -1.2635233e-07, 0.6485172, 1.0], [1.0049, -2.2340859e-07, 0.5983485, 1.0], [1.10535, -3.2556198e-07, 0.54804605, 1.0], [1.20585, -4.3832975e-07, 0.49776268, 1.0], [1.30635, -5.69768e-07, 0.4476513, 1.0], [1.4067999, -7.1970504e-07, 0.39734882, 1.0], [1.5073, -8.8991624e-07, 0.34698907, 1.0], [1.6077499, -1.0825205e-06, 0.29668662, 1.0], [1.7082499, -1.2993553e-06, 0.24649878, 1.0], [1.8087, -1.5556518e-06, 0.1961008, 1.0], [1.9092, -1.8493804e-06, 0.1459321, 1.0], [2.0097, -2.1908543e-06, 0.09568695, 1.0], [2.1101499, -2.5915322e-06, 0.04548002, 1.0], [2.21065, -3.023531e-06, -0.0047842218, 1.0], [2.3111, -3.4648879e-06, -0.055105776, 1.0], [2.4115999, -3.88199e-06, -0.10525539, 1.0], [2.5121, -4.2503925e-06, -0.155405, 1.0], [2.61255, -4.5876645e-06, -0.20566924, 1.0], [2.71305, -4.902974e-06, -0.25600988, 1.0]] ("JVData 2")
    n61 = Number To Decimal String(number=w191) -> (decimal integer string=w184:string)  [unwired: 1 in]
    n62 = Concatenate Strings(w189, w184) -> (w192:string)
    n63 = Concatenate Strings(w188, w184) -> (w187:string)
    n64 = Concatenate Strings(w183, w184) -> (w186:string)
    n65 = Obtain Queue(name (unnamed)=w192, element data type=dbl[] [0.0, 0.6932165634222212, 0.002936372303467471, 0.2869923716049554, 0.0005841850023007069, 0.39914193749427795, 0.001463602161096093, 0.0, 0.0, 0.0, 0.0, 0.0, 0.0, inf] ("appended array 2")) -> (queue out=w190:refnum<queue>)  [unwired: 3 in, 2 out]
    n66 = Obtain Queue(name (unnamed)=w187, element data type=w185) -> (queue out=w182:refnum<queue>)  [unwired: 3 in, 2 out]
    n67 = Obtain Queue(name (unnamed)=w186, element data type=w185) -> (queue out=w181:refnum<queue>)  [unwired: 3 in, 2 out]
  }
  n68 = while {
    stop <- w210 stop-if-true
    w213 = T5 []
    n69 = local read "DataForAnalysis"() -> (w196:T10)
    n70 = Array Size(array=w196) -> (size(s)=w204:i32)
    n71 = Subtract(x=w204, y=14) -> (x-y=w202:i32)
    n72 = Build Array("Scrollbar") -> (w205:i32[])
    n73 = property on="DataForAnalysis" class="Arr"("Index Values"=w205) -> ()  [unwired: 2 in, 2 out]
    n74 = Max & Min(x=0, y=w202) -> (max(x,y)=w200:i32)  [unwired: 1 out]
    n75 = property on="Scrollbar" class="Scroll (strict)"("DocMax"=w200) -> ()  [unwired: 2 in, 2 out]
    n76 = case shown="True" "Hide all Button" {
      tunnel: w196 -> [_ w218]
      frame False {
      }
      frame True {
        n77 = for {
          tunnel: w218 -> [w221] mode=indexing
          tunnel: [w219] -> w217 mode=indexing
          n78 = Bundle By Name(cluster=w221, "ViewJV"=FALSE) -> (w219:T1)
        }
        n79 = local write "DataForAnalysis"(w217) -> ()
      }
    }
    n80 = for {
      tunnel: w196 -> [w239] mode=indexing
      shift-right: [w237] -> w214
      shift-left: w213 -> [w238]
      shift-right: [w235] -> w212
      shift-left: w213 -> [w236]
      shift-right: [w234] -> w194
      shift-left: dbl[] [] -> [w233]
      tunnel: w196 -> [w229]
      shift-right: [w225] -> _
      shift-left: 0 -> [w226]
      i -> [w227]
      n81 = Unbundle By Name(w239) -> ("ViewJV"=w231:bool, "Delete"=w228:bool)
      n82 = case shown="True" w228 {
        tunnel: w229 -> [_ w242]
        tunnel: w227 -> [_ w241]
        frame False {
        }
        frame True {
          n83 = Delete From Array(array=w242, index=w241) -> (array with subset deleted=w240:T10)  [unwired: 1 in, 1 out]
          n84 = local write "DataForAnalysis"(w240) -> ()
        }
      }
      n85 = Not(x=w228) -> (.not. x?=w230:bool)
      n86 = And(x=w231, y=w230) -> (x .and. y?=w232:bool)
      n87 = case shown="True" w232 {
        tunnel: w239 -> [_ w291]
        tunnel: w238 -> [w246 w284]
        tunnel: [w246 w285] -> w237
        tunnel: w236 -> [w245 w265]
        tunnel: [w245 w263] -> w235
        tunnel: [w244 w261] -> w234
        tunnel: w233 -> [w244 w260]
        tunnel: w226 -> [w243 w248]
        tunnel: [w243 w257] -> w225
        frame False {
        }
        frame True {
          # "I"
          # "Ewe"
          # "t"
          # "Ewe"
          # "I"
          # "t"
          n88 = Unbundle By Name(w291) -> ("Name"=w255:string, "TimeMeasured"=w254:timestamp, "JVData"=w290:dbl[][], "TransientData"=w270:dbl[][])
          n89 = Index Array(array=w290, index (col) #1=0 ("Index"), index (col) #2=1 ("Index"), index (col) #3=2 ("Index")) -> (element #1=w289:dbl[], element #2=w287:dbl[], element #3=w288:dbl[])  [unwired: 3 in]
          n90 = Index Array(array=w270, index (col)=2 ("disabled index (col)")) -> (element=w266:dbl[])  [unwired: 1 in]
          n91 = Index Array(array=w270, index (col)=1 ("disabled index (col)")) -> (element=w272:dbl[])  [unwired: 1 in]
          n92 = Index Array(array=w270, index (col)=0 ("disabled index (col)")) -> (element=w273:dbl[])  [unwired: 1 in]
          n93 = Format Date/Time String(time format string (%c)=" %H:%M", seconds (now)=w254) -> (date/time string=w253:string)  [unwired: 1 in]
          n94 = Concatenate Strings(w255, w253) -> (w256:string)
          n95 = Array Size(array=w273) -> (size(s)=w275:i32)
          n96 = Multiply(x=w272, y=w266) -> (x*y=w271:dbl[])
          n97 = case shown="\"I(t)\"" "Select how to plot:" {
            tunnel: w289 -> [_ _ _ _ _ w351 w356]
            tunnel: w288 -> [w318 w326 w329 w335 w343 _ w355]
            tunnel: [w317 w327 w333 w334 w342 w347 w352] -> w286
            tunnel: "Potential (V)" ("Y Scale.Name Label.Text") -> [w321 w322 w330 w338 w346 w350 _]
            tunnel: "Current density (mA/cm2)" ("Y Scale.Name Label.Text") -> [w320 w323 w331 _ _ _ w354]
            tunnel: [w320 w323 w331 w337 w345 w350 w354] -> w292
            tunnel: [w321 w322 w330 w338 w346 w349 w353] -> w293
            tunnel: "Time (s)" ("Y Scale.Name Label.Text") -> [_ _ _ _ _ w349 w353]
            tunnel: w287 -> [w319 w324 w332 w336 w344 w348 _]
            tunnel: "Power (W)" ("Y Scale.Name Label.Text") -> [_ _ _ w337 w345 _ _]
            frame "J(V)" {
              n98 = Bundle("JVData"=w319, "JVData"=w318) -> (w317:cluster{"JVData":dbl[], "JVData":dbl[]})  [unwired: 1 in]
            }
            frame "-J(V)" {
              n99 = Negate(x=w326) -> (-x=w325:dbl[])
              n100 = Bundle("JVData"=w324, w325) -> (w327:cluster{"JVData":dbl[], dbl[]})  [unwired: 1 in]
            }
            frame "abs J(V)" {
              n101 = Absolute Value(x=w329) -> (abs(x)=w328:dbl[])
              n102 = Bundle("JVData"=w332, w328) -> (w333:cluster{"JVData":dbl[], dbl[]})  [unwired: 1 in]
            }
            frame "P(V)" {
              n103 = Multiply(x=w335, y=w336) -> (x*y=w339:dbl[])
              n104 = Bundle("JVData"=w336, w339) -> (w334:cluster{"JVData":dbl[], dbl[]})  [unwired: 1 in]
            }
            frame "-P(V)" {
              n105 = Multiply(x=w343, y=w344) -> (x*y=w341:dbl[])
              n106 = Negate(x=w341) -> (-x=w340:dbl[])
              n107 = Bundle("JVData"=w344, w340) -> (w342:cluster{"JVData":dbl[], dbl[]})  [unwired: 1 in]
            }
            frame "V(t)", Default {
              n108 = Bundle("JVData"=w351, "JVData"=w348) -> (w347:cluster{"JVData":dbl[], "JVData":dbl[]})  [unwired: 1 in]
            }
            frame "I(t)" {
              n109 = Bundle("JVData"=w356, "JVData"=w355) -> (w352:cluster{"JVData":dbl[], "JVData":dbl[]})  [unwired: 1 in]
            }
          }
          n110 = case shown="\"I(t)\"" "Select how to plot:" {
            tunnel: w273 -> [w306 w307 w314]
            tunnel: [w303 w308 w312] -> w264
            tunnel: "Potential (V)" ("Y Scale.Name Label.Text") -> [w305 _ _]
            tunnel: "Current density (mA/cm2)" ("Y Scale.Name Label.Text") -> [_ w311 _]
            tunnel: [w305 w311 w315] -> w279
            tunnel: [w304 w310 w316] -> w278
            tunnel: "Time (s)" ("Y Scale.Name Label.Text") -> [w304 w310 w316]
            tunnel: w272 -> [w302 _ _]
            tunnel: w266 -> [_ w309 _]
            tunnel: "Power (mW/cm2)" ("Y Scale.Name Label.Text") -> [_ _ w315]
            tunnel: w271 -> [_ _ w313]
            frame "V(t)", Default {
              n111 = Bundle("TransientData"=w306, "TransientData"=w302) -> (w303:T13)  [unwired: 1 in]
            }
            frame "I(t)" {
              n112 = Bundle("TransientData"=w307, "TransientData"=w309) -> (w308:T13)  [unwired: 1 in]
            }
            frame "P(t)" {
              n113 = Bundle("TransientData"=w314, w313) -> (w312:cluster{"TransientData":dbl[], dbl[]})  [unwired: 1 in]
            }
          }
          n114 = Subtract(x=w275, y=1) -> (x-y=w283:i32)
          n115 = Increment(x=w248) -> (x+1=w257:i32)
          n116 = control-ref of="XY Graph 11"() -> (w247:refnum<vi>)
          n117 = Index Array(array=w271, index=w283) -> (element=w262:dbl)
          n118 = control-ref of="XY Graph 10"() -> (w259:refnum<vi>)
          n119 = property on="XY Graph 10" class="XYGraph (strict)"("X Scale.Name Label.Text"=w293) -> ()  [unwired: 2 in, 2 out]
          n120 = property on="XY Graph 10" class="XYGraph (strict)"("Y Scale.Name Label.Text"=w292) -> ()  [unwired: 2 in, 2 out]
          n121 = property on="XY Graph 11" class="XYGraph (strict)"("X Scale.Name Label.Text"=w278) -> ()  [unwired: 2 in, 2 out]
          n122 = property on="XY Graph 11" class="XYGraph (strict)"("Y Scale.Name Label.Text"=w279) -> ()  [unwired: 2 in, 2 out]
          n123 = property class="XYGraph (strict)"(reference=w259, "Active Plot"=w248, "Plot.Point Style"=u8 1, "Plot.Plot Name"=w256) -> ("Plot.Plot Color"=w249:u32, "Plot.Fill/Pt. Color"=w250:u32)  [unwired: 1 in, 2 out]
          n124 = property class="XYGraph (strict)"(reference=w247, "Active Plot"=w248, "Plot.Plot Color"=w249, "Plot.Point Style"=u8 1, "Plot.Fill/Pt. Color"=w250) -> ()  [unwired: 1 in, 2 out]
          n125 = Build Array (concatenate)(w260, w262) -> (w261:dbl[])
          n126 = Build Array (concatenate)(w265, w264) -> (w263:T11)
          n127 = Build Array (concatenate)(w284, w286) -> (w285:cluster{"JVData":dbl[], "JVData":dbl[]}[])
        }
      }
    }
    "XY Graph 10" <- w214
    "XY Graph 11" <- w212
    n128 = case shown="True" "DeleteAll Button" {
      frame False {
      }
      frame True {
        n129 = local write "DataForAnalysis"(T10 [] ("DataForAnalysis")) -> ()
      }
    }
    n130 = case shown="True" "Save Button" {
      frame False {
      }
      frame True {
        n131 = local read "DataForAnalysis"() -> (w223:T10)
        n132 = call "ExportDataToExcel.vi"("DataForAnalysis"=w223, "title"="Project name") -> ()  [unwired: 2 in]
      }
    }
    n133 = case shown="True" "Save Button 2" {
      frame False {
      }
      frame True {
        n134 = local read "DataForAnalysis"() -> (w222:T10)
        n135 = call "ExportToWord.vi"("DataForAnalysis"=w222) -> ()  [unwired: 11 in]
      }
    }
    n136 = Array Size(array=w214) -> (size(s)=w215:i32)
    n137 = Negate(x=w194) -> (-x=→"Final power (mW/cm2)":dbl[])
    n138 = Array Size(array=w194) -> (size(s)=w199:i32)
    n139 = property on="XY Graph 10" class="XYGraph (strict)"("LegNumRows"=w215) -> ()  [unwired: 2 in, 2 out]
    n140 = Wait Until Next ms Multiple(millisecond multiple=u32 500) -> ()  [unwired: 1 out]
    n141 = local read "Exit"() -> (w210:bool)
    n142 = property on="Final power (mW/cm2)" class="Arr (strict)"("Number of Rows"=w199) -> ()  [unwired: 2 in, 2 out]
  }
  n143 = for {
    N: "NoOfChannels" -> [_]
    tunnel: [w360] -> w12 mode=indexing
    tunnel: [w359] -> w8 mode=indexing
    n144 = Obtain Queue(element data type=dbl[] [0.0, 0.6932165634222212, 0.002936372303467471, 0.2869923716049554, 0.0005841850023007069, 0.39914193749427795, 0.001463602161096093, 0.0, 0.0, 0.0, 0.0, 0.0, 0.0, inf] ("appended array 2")) -> (queue out=w360:refnum<queue>)  [unwired: 4 in, 2 out]
    n145 = Obtain Queue(element data type=sgl[][] [[0.100549996, 1.4351095e-06, 1.050421, 1.0], [0.20105, 9.236625e-07, 1.0001758, 1.0], [0.30155, 6.189802e-07, 0.9500262, 1.0], [0.40199998, 4.1734597e-07, 0.8998193, 1.0], [0.5025, 2.727543e-07, 0.84953594, 1.0], [0.60295, 1.5926109e-07, 0.79927176, 1.0], [0.70344996, 6.1173935e-08, 0.74896926, 1.0], [0.80394995, -3.2675118e-08, 0.6988388, 1.0], [0.9044, -1.2635233e-07, 0.6485172, 1.0], [1.0049, -2.2340859e-07, 0.5983485, 1.0], [1.10535, -3.2556198e-07, 0.54804605, 1.0], [1.20585, -4.3832975e-07, 0.49776268, 1.0], [1.30635, -5.69768e-07, 0.4476513, 1.0], [1.4067999, -7.1970504e-07, 0.39734882, 1.0], [1.5073, -8.8991624e-07, 0.34698907, 1.0], [1.6077499, -1.0825205e-06, 0.29668662, 1.0], [1.7082499, -1.2993553e-06, 0.24649878, 1.0], [1.8087, -1.5556518e-06, 0.1961008, 1.0], [1.9092, -1.8493804e-06, 0.1459321, 1.0], [2.0097, -2.1908543e-06, 0.09568695, 1.0], [2.1101499, -2.5915322e-06, 0.04548002, 1.0], [2.21065, -3.023531e-06, -0.0047842218, 1.0], [2.3111, -3.4648879e-06, -0.055105776, 1.0], [2.4115999, -3.88199e-06, -0.10525539, 1.0], [2.5121, -4.2503925e-06, -0.155405, 1.0], [2.61255, -4.5876645e-06, -0.20566924, 1.0], [2.71305, -4.902974e-06, -0.25600988, 1.0]] ("JVData 2")) -> (queue out=w359:refnum<queue>)  [unwired: 4 in, 2 out]
  }
  n146 = Obtain Queue(element data type=0) -> (queue out=w6:refnum<queue>)  [unwired: 4 in, 2 out]
  n147 = while {
    tunnel: w12 -> [w369]
    tunnel: w8 -> [w366]
    tunnel: "NoOfChannels" -> [w361]
    tunnel: [w364] -> w19
    tunnel: [w363] -> w20
    stop <- w367 stop-if-true
    n148 = for {
      N: w361 -> [_]
      tunnel: w369 -> [w410] mode=indexing
      tunnel: [w409] -> w368 mode=indexing
      tunnel: [w403] -> w362 mode=indexing
      workers-P: w361 -> [_]
      tunnel: w366 -> [w408] mode=indexing
      tunnel: [w406] -> w365 mode=indexing
      tunnel: [w405] -> w364 mode=indexing
      tunnel: [w404] -> w363 mode=indexing
      n149 = Dequeue Element(queue=w410, timeout in ms (-1)=100) -> (queue out=w404:refnum<queue>, element=w409:dbl[], timed out?=w403:bool)  [unwired: 1 in, 1 out]
      n150 = case shown="False" w403 {
        tunnel: w408 -> [w413 w414]
        tunnel: [w412 _] -> w406
        tunnel: [w411 w414] -> w405
        frame False {
          n151 = Dequeue Element(queue=w413) -> (queue out=w411:refnum<queue>, element=w412:sgl[][])  [unwired: 2 in, 2 out]
        }
        frame True {
        }
      }
    }
    n152 = for {
      N: w361 -> [_]
      tunnel: w368 -> [w371] mode=indexing
      tunnel: w362 -> [w373] mode=indexing
      tunnel: w365 -> [w370] mode=indexing
      i -> [w372]
      n153 = case shown="False" w373 {
        tunnel: w372 -> [w379 _]
        tunnel: w371 -> [w377 _]
        tunnel: w370 -> [w378 _]
        frame False {
          n154 = local read "ChannelData"() -> (w375:T2)
          n155 = Array Size(array=w377) -> (size(s)=w376:i32)
          n156 = case shown="0, Default" w376 {
            tunnel: w377 -> [w391 _]
            tunnel: w379 -> [w386 w400]
            tunnel: w378 -> [w381 _]
            tunnel: w375 -> [w385 w399]
            tunnel: [w384 w397] -> w374
            frame 0, Default {
              n157 = Index Array(array=w385, index=w386) -> (element=w388:cluster{"JV metrics":sgl[][], "JVData":sgl[][]})
              n158 = Array Size(array=w381) -> (size(s)=w383:i32[])
              n159 = Unbundle By Name(w388) -> ("JV metrics"=w390:sgl[][])
              n160 = Index Array(array=w383, index=0) -> (element=w380:i32)
              n161 = Build Array (concatenate)(w390, w391) -> (w389:dbl[][])
              n162 = Bundle By Name(cluster=w388, "JV metrics"=w389, "JVData"=w381) -> (w387:cluster{"JV metrics":sgl[][], "JVData":sgl[][]})
              n163 = case shown="1, Default" w380 {
                tunnel: w387 -> [_ w396]
                tunnel: w386 -> [_ w395]
                tunnel: w385 -> [w392 w394]
                tunnel: [w392 w393] -> w384
                frame 0 {
                }
                frame 1, Default {
                  n164 = Replace Array Subset(array=w394, new element=w396, index=w395) -> (w393:T2)
                }
              }
            }
            frame 1 {
              w402 = sgl[][] [] ("JV metrics")
              n165 = Index Array(array=w399, index=w400) -> (element=w401:cluster{"JV metrics":sgl[][], "JVData":sgl[][]})
              n166 = Bundle By Name(cluster=w401, "JV metrics"=w402, "JVData"=w402) -> (w398:cluster{"JV metrics":sgl[][], "JVData":sgl[][]})
              n167 = Replace Array Subset(array=w399, new element=w398, index=w400) -> (w397:T2)
            }
          }
          n168 = local write "ChannelData"(w374) -> ()
        }
        frame True {
        }
      }
    }
    n169 = local read "Exit"() -> (w367:bool)
  }
  n170 = while {
    tunnel: "NoOfChannels" -> [w416]
    tunnel: w11 -> [w415]
    stop <- w417 stop-if-true
    n171 = for {
      N: w416 -> [_]
      tunnel: w415 -> [w418] mode=indexing
      i -> [w420]
      n172 = Dequeue Element(queue=w418, timeout in ms (-1)=5) -> (element=w419:dbl[], timed out?=w421:bool)  [unwired: 1 in, 2 out]
      n173 = case shown="False" w421 {
        tunnel: w420 -> [w427 _]
        tunnel: w419 -> [w426 _]
        frame False {
          n174 = local read "ChannelAgingData"() -> (w424:cluster{"AgingData":sgl[][]}[])
          n175 = Array Size(array=w426) -> (size(s)=w425:i32)
          n176 = case shown="1" w425 {
            tunnel: w426 -> [w435 _]
            tunnel: w427 -> [w430 w436]
            tunnel: w424 -> [w429 w440]
            tunnel: [w428 w438] -> w423
            frame 0, Default {
              n177 = Index Array(array=w429, index=w430) -> (element=w432:cluster{"AgingData":sgl[][]})
              n178 = Unbundle By Name(w432) -> ("AgingData"=w434:sgl[][])
              n179 = Build Array (concatenate)(w434, w435) -> (w433:dbl[][])
              n180 = Bundle By Name(cluster=w432, "AgingData"=w433) -> (w431:cluster{"AgingData":sgl[][]})
              n181 = Replace Array Subset(array=w429, new element=w431, index=w430) -> (w428:cluster{"AgingData":sgl[][]}[])
            }
            frame 1 {
              n182 = Index Array(array=w440, index=w436) -> (element=w441:cluster{"AgingData":sgl[][]})
              n183 = Bundle By Name(cluster=w441, "AgingData"=dbl[][] [] ("appended array 2")) -> (w439:cluster{"AgingData":sgl[][]})
              n184 = Replace Array Subset(array=w440, new element=w439, index=w436) -> (w438:cluster{"AgingData":sgl[][]}[])
            }
          }
          n185 = local write "ChannelAgingData"(w423) -> ()
        }
        frame True {
        }
      }
    }
    n186 = local read "Exit"() -> (w417:bool)
  }
  n187 = while {
    tunnel: w21 -> [w446]
    tunnel: w7 -> [w445]
    tunnel: [w442] -> w18
    tunnel: w6 -> [w448]
    tunnel: [w447] -> w5
    tunnel: "NoOfChannels" -> [w444]
    tunnel: [w443] -> w3
    stop <- w449 stop-if-true
    n188 = stacked-sequence {
      tunnel: w448 -> [w455 _]
      tunnel: [w454 _] -> w447
      tunnel: w446 -> [w452 w552]
      tunnel: w445 -> [w453 w551]
      tunnel: w444 -> [_ w550]
      tunnel: [_ w549] -> w443
      tunnel: [_ w548] -> w442
      frame #0 {
        n189 = Dequeue Element(queue=w455, timeout in ms (-1)=1) -> (queue out=w454:refnum<queue>, element=w456:i32, timed out?=w450:bool)  [unwired: 1 in, 1 out]
        "Boolean" <- w450
        n190 = case shown="False" w450 {
          tunnel: w456 -> [w465 _]
          tunnel: w453 -> [w500 _]
          tunnel: w452 -> [w499 _]
          frame False {
            n191 = local read "ChannelData"() -> (w534:T2)
            n192 = local read "ResetJVLiveView"() -> (w517:bool[])
            n193 = local read "ConfigTable"() -> (w531:T4)
            n194 = Index Array(array=w534, index=w465) -> (element=w533:cluster{"JV metrics":sgl[][], "JVData":sgl[][]})
            n195 = Index Array(array=w531, index=w465) -> (element=w508:T14)
            n196 = Unbundle By Name(w508) -> ("ActiveArea cm2"=w472:dbl, "RunCont"=w473:bool)
            n197 = Replace Array Subset(array=w517, new element=TRUE ("new element/subarray"), index=w465) -> (w518:bool[])
            n198 = local read "Channel Names"() -> (w482:string[])
            n199 = local write "ResetJVLiveView"(w518) -> ()
            n200 = Unbundle By Name(w533) -> ("JVData"=w462:sgl[][], "JV metrics"=w530:sgl[][])
            n201 = Array Size(array=w530) -> (size(s)=w529:i32[])
            n202 = Index Array(array=w482, index=w465) -> (element=w481:string)
            n203 = global read "ActiveArray.vi" "Active"() -> (w464:bool[])
            n204 = case shown="False" w473 {
              selector: w473 -> [w546 _]
              tunnel: w465 -> [w547 _]
              tunnel: w464 -> [w544 _]
              frame False {
                n205 = Replace Array Subset(array=w544, new element=w546, index=w547) -> (w545:bool[])
                n206 = global write "ActiveArray.vi" "Active"(w545) -> ()
              }
              frame True {
              }
            }
            n207 = Index Array(array=w529) -> (element=w510:i32)  [unwired: 1 in]
            n208 = local read "ResetAgingLiveView"() -> (w514:bool[])
            n209 = Decrement(x=w510) -> (x-1=w509:i32)
            n210 = Index Array(array=w530, index (row)=w509) -> (element=w476:sgl[])  [unwired: 1 in]
            n211 = Array Subset(array=w476, index=1, length=4) -> (w523:sgl[])
            n212 = Array Subset(array=w476, index=7, length=4) -> (w478:sgl[])
            n213 = Index Array(array=w476, index=11) -> (element=w477:sgl)
            n214 = Array Subset(array=w476, index=14) -> (w479:sgl[])  [unwired: 1 in]
            n215 = Index Array(array=w476, index=4) -> (element=w520:sgl)
            n216 = Build Array (concatenate)(w523, w478, w477, w479) -> (w522:sgl[])
            n217 = Get Date/Time In Seconds() -> (seconds since 1Jan1904=w528:timestamp)
            n218 = Replace Array Subset(array=w514, new element=TRUE ("new element/subarray"), index=w465) -> (w513:bool[])
            n219 = local write "ResetAgingLiveView"(w513) -> ()
            n220 = Array Size(array=w462) -> (size(s)=w485:i32[])
            n221 = Index Array(array=w464, index=w465) -> (element=w458:bool)
            n222 = Index Array(array=w485, index=0) -> (element=w461:i32)
            n223 = Greater?(x=w461, y=1) -> (0:w459:bool)
            n224 = And(x=w459, y=w458) -> (x .and. y?=w457:bool)
            n225 = local read "DataForAnalysis"() -> (w507:T10)
            n226 = Array Subset(array=w507, index=0, length="Keep latest JV data") -> (w504:T10)
            n227 = local read "LiveViewData"() -> (w503:cluster{"JVData":sgl[][], "AgingData":sgl[][]}[])
            n228 = Index Array(array=w499, index=w465) -> (element=w498:refnum<queue>)
            n229 = Index Array(array=w500, index=w465) -> (element=w497:refnum<queue>)
            n230 = Flush Queue(queue=w498) -> (remaining elements=w496:cluster{"JVData 2":sgl[][]}[])  [unwired: 1 in, 2 out]
            n231 = Index Array(array=w503, index=w465) -> (element=w501:cluster{"JVData":sgl[][], "AgingData":sgl[][]})
            n232 = Unbundle By Name(w501) -> ("AgingData"=w494:sgl[][], "JVData"=w491:sgl[][])
            n233 = Flush Queue(queue=w497) -> (remaining elements=w489:cluster{"JVData 2":sgl[][]}[])  [unwired: 1 in, 2 out]
            n234 = for {
              tunnel: w496 -> [w543] mode=indexing
              shift-right: [w540] -> w493
              shift-left: sgl[][] [] -> [w542]
              n235 = Unbundle By Name(w543) -> ("JVData 2"=w541:sgl[][])
              n236 = Build Array (concatenate)(w542, w541) -> (w540:sgl[][])
            }
            n237 = for {
              tunnel: w489 -> [w539] mode=indexing
              shift-right: [w536] -> w487
              shift-left: sgl[][] [] -> [w538]
              n238 = Unbundle By Name(w539) -> ("JVData 2"=w537:sgl[][])
              n239 = Build Array (concatenate)(w538, w537) -> (w536:sgl[][])
            }
            n240 = Build Array (concatenate)(w494, w493) -> (w492:sgl[][])
            n241 = Build Array (concatenate)(w491, w487) -> (w490:sgl[][])
            n242 = Bundle By Name(cluster=w501, "AgingData"=w492, "JVData"=w490) -> (w502:cluster{"JVData":sgl[][], "AgingData":sgl[][]})
            n243 = Replace Array Subset(array=w503, new element=w502, index=w465) -> (w486:cluster{"JVData":sgl[][], "AgingData":sgl[][]}[])
            n244 = Index Array(array=w486, index=w465) -> (element=w532:cluster{"JVData":sgl[][], "AgingData":sgl[][]})
            n245 = Unbundle By Name(w532) -> ("AgingData"=w471:sgl[][])
            n246 = Index Array(array=w471, index (col)=2 ("disabled index (col)")) -> (element=w468:sgl[])  [unwired: 1 in]
            n247 = Multiply(x=1000, y=w468) -> (x*y=w474:sgl[])
            n248 = Divide(x=w474, y=w472) -> (x/y=w467:dbl[])
            n249 = Replace Array Subset(array=w471, new element=w467, index (col)=2 ("disabled index (col)")) -> (w463:sgl[][])  [unwired: 1 in]
            n250 = Bundle By Name(cluster="DataForAnalysisE", "JVData"=w462, "JVmetrics"=w522, "TransientData"=w463, "Name"=w481, "TimeMeasured"=w528, "Eff"=w520) -> (w512:T1)
            n251 = Insert Into Array(array=w504, index=0, new element=w512) -> (w483:T10)
            n252 = case shown="True" w457 {
              tunnel: w483 -> [_ w535]
              frame False {
              }
              frame True {
                n253 = local write "DataForAnalysis"(w535) -> ()
              }
            }
            n254 = local write "LiveViewData"(w486) -> ()
          }
          frame True {
          }
        }
      }
      frame #1 {
        n255 = for {
          N: w550 -> [_]
          tunnel: w552 -> [w556] mode=indexing
          tunnel: w551 -> [w555] mode=indexing
          tunnel: [w554] -> w549 mode=indexing
          tunnel: [w553] -> w548 mode=indexing
          i -> [w557]
          n256 = local read "LiveViewData"() -> (w558:cluster{"JVData":sgl[][], "AgingData":sgl[][]}[])
          n257 = Index Array(array=w558, index=w557) -> (element=w563:cluster{"JVData":sgl[][], "AgingData":sgl[][]})
          n258 = Dequeue Element(queue=w556, timeout in ms (-1)=5) -> (queue out=w554:refnum<queue>, element=w566:sgl[][], timed out?=w567:bool)  [unwired: 1 in, 1 out]
          n259 = Dequeue Element(queue=w555, timeout in ms (-1)=5) -> (queue out=w553:refnum<queue>, element=w560:sgl[][], timed out?=w564:bool)  [unwired: 1 in, 1 out]
          n260 = case shown="False" w567 {
            tunnel: w566 -> [w593 _]
            tunnel: w563 -> [w590 w619]
            tunnel: [w589 w619] -> w562
            tunnel: w557 -> [w586 _]
            frame False {
              n261 = local read "ResetAgingLiveView"() -> (w587:bool[])
              n262 = Unbundle By Name(w590) -> ("AgingData"=w591:sgl[][])
              n263 = Index Array(array=w587, index=w586) -> (element=w588:bool)
              n264 = case shown="False" w588 {
                tunnel: w593 -> [w597 w614]
                tunnel: [w599 w614] -> w592
                tunnel: w591 -> [w598 _]
                tunnel: w587 -> [_ w617]
                tunnel: w586 -> [_ w616]
                frame False {
                  n265 = Array Size(array=w597) -> (size(s)=w596:i32[])
                  n266 = Index Array(array=w596, index=0) -> (element=w594:i32)
                  n267 = case shown="0" w594 {
                    tunnel: [w600 w609] -> w599
                    tunnel: w598 -> [w600 w601]
                    tunnel: w597 -> [_ w602]
                    frame 0 {
                    }
                    frame 1, Default {
                      w608 = 0 ("disabled index (col)")
                      n268 = Index Array(array=w601, index (col)=0 ("disabled index (col)")) -> (element=w604:sgl[])  [unwired: 1 in]
                      n269 = Index Array(array=w602, index (row)=w608, index (col)=w608) -> (element=w607:sgl)
                      n270 = Array Max & Min(array=w604) -> (max value=w603:sgl)  [unwired: 3 out]
                      n271 = Greater Or Equal?(x=w607, y=w603) -> (x >= y?=w606:bool)
                      n272 = case shown="True" w606 {
                        tunnel: [w610 w613] -> w609
                        tunnel: w601 -> [_ w612]
                        tunnel: w602 -> [w610 w611]
                        frame False {
                        }
                        frame True {
                          n273 = Build Array (concatenate)(w612, w611) -> (w613:sgl[][])
                        }
                      }
                    }
                  }
                }
                frame True {
                  n274 = Replace Array Subset(array=w617, new element=FALSE ("new element/subarray"), index=w616) -> (w618:bool[])
                  n275 = local write "ResetAgingLiveView"(w618) -> ()
                }
              }
              n276 = Bundle By Name(cluster=w590, "AgingData"=w592) -> (w589:cluster{"JVData":sgl[][], "AgingData":sgl[][]})
            }
            frame True {
            }
          }
          n277 = case shown="False" w564 {
            tunnel: w562 -> [w576 w585]
            tunnel: [w575 w585] -> w559
            tunnel: w560 -> [w573 _]
            tunnel: w557 -> [w570 _]
            frame False {
              n278 = local read "ResetJVLiveView"() -> (w569:bool[])
              n279 = Unbundle By Name(w576) -> ("JVData"=w574:sgl[][])
              n280 = Index Array(array=w569, index=w570) -> (element=w571:bool)
              n281 = case shown="False" w571 {
                tunnel: w574 -> [w579 _]
                tunnel: w573 -> [w578 w584]
                tunnel: [w577 w584] -> w572
                tunnel: w570 -> [_ w582]
                tunnel: w569 -> [_ w581]
                frame False {
                  n282 = Build Array (concatenate)(w579, w578) -> (w577:sgl[][])
                }
                frame True {
                  n283 = Replace Array Subset(array=w581, new element=FALSE ("new element/subarray"), index=w582) -> (w583:bool[])
                  n284 = local write "ResetJVLiveView"(w583) -> ()
                }
              }
              n285 = Bundle By Name(cluster=w576, "JVData"=w572) -> (w575:cluster{"JVData":sgl[][], "AgingData":sgl[][]})
              "JVData 2" <- w573
            }
            frame True {
            }
          }
          n286 = Replace Array Subset(array=w558, new element=w559, index=w557) -> (w561:cluster{"JVData":sgl[][], "AgingData":sgl[][]}[])
          "output array" <- w561
          n287 = local write "LiveViewData"(w561) -> ()
        }
      }
    }
    n288 = local read "Exit"() -> (w449:bool)
  }
  n289 = Release Queue(queue=w5, force destroy? (F)=TRUE) -> ()  [unwired: 1 in, 3 out]
  n290 = call "PromptIP.vi"("IP"="IP adress") -> ("IP"=w9:string, "OK"=w25:bool, "error out"=w26:errorcluster)  [unwired: 16 in]
  n291 = case shown="False" w25 {
    frame False {
      n292 = local write "Exit"(TRUE ("Exit")) -> ()
    }
    frame True {
    }
  }
  n293 = local write "IP adress"(w9) -> ()
  n294 = call "connect.vi"("error in (no error)"=w26, "IP"=w9) -> ("error out"=w35:errorcluster, "Device Code"=w30:i32, "ID"=w1:i32)  [unwired: 6 in, 1 out]
  "Device Code" <- w30
  n295 = call "GetChannelplugged.vi"("error in (no error)"=w35, "ID"=w1) -> ("error out"=w33:errorcluster, "First channel"=w15:i32, "Disabled channels"=w14:i32[], "Plugged channels"=w34:i32[])  [unwired: 6 in]
  n296 = property on="First Channel" class="Ring (strict)"("Disabled Items []"=w14) -> ()  [unwired: 2 in, 2 out]
  n297 = Initialize Array(FALSE, 16 ("dimension size")) -> (w13:bool[])
  n298 = property on="Show Instance" class="Ring (strict)"("Disabled Items []"=w14) -> ()  [unwired: 2 in, 2 out]
  n299 = global write "ActiveArray.vi" "Active"(w13) -> ()
  n300 = local write "First Channel"(w15) -> ()
  n301 = local write "ResetJVLiveView"(w13) -> ()
  n302 = local write "ResetAgingLiveView"(w13) -> ()
  n303 = call "LoadFirmware.vi"("error in (no error)"=w33, "Channels"=w34, "ID"=w1) -> ("error out"=w32:errorcluster)  [unwired: 7 in, 1 out]
  n304 = for {
    N: "NoOfChannels" -> [_]
    tunnel: w20 -> [w627] mode=indexing
    tunnel: w19 -> [w625] mode=indexing
    tunnel: w3 -> [w623] mode=indexing
    tunnel: w18 -> [w621] mode=indexing
    n305 = Release Queue(queue=w627, force destroy? (F)=TRUE) -> ()  [unwired: 1 in, 3 out]
    n306 = Release Queue(queue=w625, force destroy? (F)=TRUE) -> ()  [unwired: 1 in, 3 out]
    n307 = Release Queue(queue=w623, force destroy? (F)=TRUE) -> ()  [unwired: 1 in, 3 out]
    n308 = Release Queue(queue=w621, force destroy? (F)=TRUE) -> ()  [unwired: 1 in, 3 out]
  }
  n309 = local write "Directory to save files"("Directory to save files") -> ()
  n310 = while {
    shift-right: [w644] -> w36
    shift-left: w32 -> [w642]
    tunnel: ["Exit"] -> w38
    tunnel: w1 -> [w637]
    tunnel: [w636] -> w31
    tunnel: w30 -> [w635]
    tunnel: w12 -> [w633]
    tunnel: w8 -> [w632]
    tunnel: w6 -> [w631]
    stop <- "Exit" stop-if-true
    n311 = call "GetChannelInfo.vi"("error in (no error)"=w642, "Channel"="First Channel", "ID"=w637) -> ("error out"=w641:errorcluster, "Channel information"=w638:T15)  [unwired: 7 in]
    n312 = local read "NoOfChannels"() -> (w629:i32)
    n313 = Cluster To Array(cluster=w638) -> (array=w640:i32[])
    n314 = Cluster To Array(cluster=w638) -> (array=w639:i32[])
    n315 = call "max_min_irange.vi"("resources"=w640) -> ()  [unwired: 1 out]
    n316 = call "max_bdwidth.vi"("resources"=w639) -> ()  [unwired: 1 out]
    n317 = for {
      N: w629 -> [_]
      tunnel: w637 -> [w651]
      tunnel: [w650] -> w636
      tunnel: w635 -> [w649]
      workers-P: w629 -> [_]
      tunnel: w641 -> [w652]
      tunnel: [w653] -> w644
      tunnel: w633 -> [w647] mode=indexing
      tunnel: w632 -> [w646] mode=indexing
      tunnel: w631 -> [w645]
      i -> [w648]
      n318 = while {
        tunnel: w651 -> [w667]
        tunnel: [w666] -> w650
        tunnel: w649 -> [w665]
        tunnel: w648 -> [w654]
        shift-right: [w669] -> w653
        shift-left: w652 -> [w668]
        tunnel: w647 -> [w657]
        tunnel: w646 -> [w656]
        tunnel: w645 -> [w655]
        stop <- w659 stop-if-true
        n319 = global read "ActiveArray.vi" "Active"() -> (w664:bool[])
        n320 = local read "ConfigTable"() -> (w662:T4)
        n321 = Index Array(array=w662, index=w654) -> (element=w661:T14)
        n322 = Unbundle By Name(w661) -> ("Channel"=w660:u8)
        n323 = Index Array(array=w664, index=w654) -> (element=w663:bool)
        n324 = case shown="True" w663 {
          tunnel: w660 -> [w675 w701]
          tunnel: [w676 w702] -> w669
          tunnel: w668 -> [w677 w703]
          tunnel: w667 -> [w671 w699]
          tunnel: [w670 w698] -> w666
          tunnel: w665 -> [w674 w700]
          tunnel: w657 -> [_ w697]
          tunnel: w656 -> [_ w696]
          tunnel: w655 -> [_ w692]
          tunnel: w654 -> [w673 w691]
          frame False {
            n325 = case shown="True" "Monitor OC of non active channels" {
              tunnel: w677 -> [w679 w689]
              tunnel: [w679 w688] -> w676
              tunnel: w675 -> [_ w687]
              tunnel: w671 -> [w678 w680]
              tunnel: w674 -> [_ w686]
              tunnel: w673 -> [_ w685]
              tunnel: [w678 w680] -> w670
              frame False {
              }
              frame True {
                n326 = Get Date/Time In Seconds() -> (seconds since 1Jan1904=w682:timestamp)
                n327 = call "VocAging.vi"("time at OC (min)"=sgl 0.01, "Device Code"=w686, "ID"=w680, "Channel"=w687, "instance"=w685, "Record_every_dT (s)"=sgl 2.0, "record every dE (V)"=sgl 2.0, "Save Data"=FALSE, "error in (no error)"=w689, "start time"=w682) -> ("error out"=w688:errorcluster)  [unwired: 4 in, 1 out]
              }
            }
          }
          frame True {
            n328 = while {
              tunnel: w701 -> [w719]
              tunnel: w699 -> [w750]
              tunnel: w700 -> [w749]
              shift-right: [w721] -> w702
              shift-left: w703 -> [w762]
              tunnel: [w737] -> w698
              tunnel: w697 -> [w729]
              tunnel: w696 -> [w727]
              tunnel: [w723] -> w695
              tunnel: [w712] -> w694
              tunnel: w692 -> [w720]
              tunnel: w691 -> [w712]
              stop <- w723 continue-if-true
              w733 = 3 ("index")
              n329 = local read "ConfigTable"() -> (w761:T4)
              n330 = Index Array(array=w761, index=w712) -> (element=w739:T14)
              n331 = Unbundle By Name(w739) -> ("AgingFile"=w738:path, "JVFile"=w724:path, "JVMetricsFile"=w742:path, "start time"=w740:timestamp, "RunCont"=w713:bool)
              n332 = Get Date/Time In Seconds() -> (seconds since 1Jan1904=w741:timestamp)
              n333 = global read "IntensityTemperature.vi" "IntTemp"() -> (w711:dbl[][])
              n334 = Subtract(x=w741, y=w740) -> (x-y=w732:dbl)
              n335 = Unbundle By Name(w739) -> ("ActiveArea cm2"=w725:dbl, "AgingMode"=w752:T16, "JVParameters"=w760:T17, "AgingParams"=w748:T18, "start time"=w743:timestamp)
              n336 = Unbundle By Name(w760) -> ("vsInitSt 3"=w717:bool, "vsInitEnd 2"=w716:bool, "Start"=w759:dbl, "End"=w758:dbl, "rate"=w718:dbl, "record dE"=w757:dbl, "equ t1"=w756:dbl, "equ t2"=w755:dbl, "Hyst"=w754:bool)
              n337 = Build Array(w717, w716) -> (w715:bool[])
              n338 = call "JV_curve.vi"("Start (V)"=w759, "End (V)"=w758, "vs init"=w715, "Equilibration time (s)"=w756, "Equilibration time back (s)"=w755, "error in (no error)"=w762, "Device Code"=w749, "Hysteresis"=w754, "instance"=w712, "VoltageRange abs and vs init"="VoltageRange abs and vs Voc", "ID"=w750, "Record every dE (mV)"=w757, "Channel"=w719, "Scan rate (mV/s)"=w718, "Device Area cm2"=w725) -> ("JVData"=w705:sgl[][], "JVParameters1st"=w736:dbl[], "JVParameters2nd"=w709:dbl[], "error out"=w751:errorcluster)  [unwired: 1 out]
              n339 = Index Array(array=w736, index=w733) -> (element=w735:dbl)
              n340 = Index Array(array=w709, index=w733) -> (element=w734:dbl)
              n341 = Divide(x=w735, y=w734) -> (x/y=w708:dbl)
              n342 = Divide(x=w732, y=3600.0) -> (x/y=w731:dbl)
              n343 = Index Array(array=w711, index (col)=w712) -> (element=w710:dbl[])  [unwired: 1 in]
              n344 = Build Array (concatenate)(w731, w736, w708, w709, w718, w710) -> (w728:dbl[])
              n345 = Enqueue Element(queue=w729, element=w728) -> ()  [unwired: 2 in, 3 out]
              n346 = Enqueue Element(queue=w727, element=w705) -> ()  [unwired: 2 in, 3 out]
              n347 = Array Size(array=w705) -> (size(s)=w707:i32[])
              n348 = Unbundle By Name(w748) -> ("Time"=w747:dbl, "StepV"=w746:dbl, "timetocheck"=w745:dbl, "average over"=w744:dbl)
              n349 = Index Array(array=w707, index=0) -> (element=w704:i32)
              n350 = case shown="1, Default" w704 {
                tunnel: w742 -> [_ w769]
                tunnel: w728 -> [_ w768]
                tunnel: w724 -> [_ w765]
                tunnel: w705 -> [_ w763]
                frame 0 {
                }
                frame 1, Default {
                  n351 = Transpose 2D Array(2D array=w763) -> (transposed array=w764:sgl[][])
                  n352 = call-poly <vilib>:"Write Delimited Spreadsheet.vi"("file path (dialog if empty)"=w765, "format (%.3f)"="%#g", "2D data"=w764, "append to file? (new file:F)"=TRUE ("append to file? (F)")) -> ()  [unwired: 10 in, 2 out]
                  n353 = call-poly <vilib>:"Write Delimited Spreadsheet.vi"("file path (dialog if empty)"=w769, "format (%.3f)"="%#g", "1D data"=w768, "append to file? (new file:F)"=TRUE ("append to file? (F)")) -> ()  [unwired: 10 in, 2 out]
                }
              }
              n354 = case shown="\"MPP\", Default" w752 {
                tunnel: w751 -> [w798 w814 w822 w840 w847]
                tunnel: w736 -> [w797 _ _ _ _]
                tunnel: w719 -> [w796 w811 w826 w843 _]
                tunnel: w750 -> [w787 w808 w825 w841 w846]
                tunnel: w749 -> [w795 w812 w828 w845 _]
                tunnel: [w794 w813 w819 w839 w847] -> w722
                tunnel: w747 -> [w793 w810 w823 w842 _]
                tunnel: w746 -> [w792 _ w824 w834 _]
                tunnel: w745 -> [w791 w802 w817 w831 _]
                tunnel: w744 -> [w790 w803 w816 w830 _]
                tunnel: w743 -> [w789 w806 w821 w838 _]
                tunnel: w738 -> [w788 w809 w820 w837 _]
                tunnel: [w787 w808 w825 w841 w846] -> w737
                tunnel: w725 -> [w786 w807 w818 w833 _]
                tunnel: w712 -> [w785 w805 w827 w844 _]
                frame "MPP", Default {
                  (unwired) TRUE
                  n355 = Index Array(array=w797, index=4) -> (element=w800:dbl)
                  n356 = call "MPPTracker.vi"("VMPP (V)"=w800, "Device Code"=w795, "ID"=w787, "Channel"=w796, "instance"=w785, "JV after\nevery (min)"=w793, "Step (V)"=w792, "device area (cm2)"=w786, "time to check (s)"=w791, "error in (no error)"=w798, "start time"=w789, "Average over"=w790, "AgingFile"=w788) -> ("error out"=w794:errorcluster)  [unwired: 2 in]
                }
                frame "Voc" {
                  n357 = Multiply(x=w802, y=w803) -> (x*y=w801:dbl)
                  n358 = call "VocAging.vi"("time at OC (min)"=w810, "Device Code"=w812, "ID"=w808, "Channel"=w811, "instance"=w805, "Record_every_dT (s)"=w801, "device area (cm2)"=w807, "Save Data"=TRUE, "error in (no error)"=w814, "start time"=w806, "AgingFile"=w809) -> ("error out"=w813:errorcluster)  [unwired: 3 in, 1 out]
                }
                frame "Fixed Voltage" {
                  n359 = Multiply(x=w817, y=w816) -> (x*y=w815:dbl)
                  n360 = call "FixedVoltageAging.vi"("VSet (V)"=w824, "Device Code"=w828, "ID"=w825, "Channel"=w826, "instance"=w827, "JV after\nevery (min)"=w823, "Record_every_dT"=w815, "device area (cm2)"=w818, "error in (no error)"=w822, "start time"=w821, "AgingFile"=w820) -> ("error out"=w819:errorcluster)  [unwired: 4 in]
                }
                frame "Fixed Current" {
                  n361 = Multiply(x=w831, y=w830) -> (x*y=w829:dbl)
                  n362 = Multiply(x=w833, y=w834) -> (x*y=w835:dbl)
                  n363 = Divide(x=w835, y=1000.0) -> (x/y=w832:dbl)
                  n364 = call "FixedCurrentAging.vi"("VSet (V)"=w832, "Device Code"=w845, "ID"=w841, "Channel"=w843, "instance"=w844, "JV after\nevery (min)"=w842, "Record_every_dT"=w829, "device area (cm2)"=w833, "error in (no error)"=w840, "start time"=w838, "AgingFile"=w837) -> ("error out"=w839:errorcluster)  [unwired: 4 in]
                }
                frame "none" {
                }
              }
              n365 = global read "ActiveArray.vi" "Active"() -> (w753:bool[])
              n366 = Index Array(array=w753, index=w712) -> (element=w726:bool)
              n367 = case shown="No Error" w722 {
                selector: w722 -> [w773 w784]
                tunnel: [w774 w784] -> w721
                tunnel: w720 -> [w777 _]
                tunnel: w712 -> [w776 _]
                tunnel: w713 -> [w775 _]
                frame No Error {
                  n368 = flat-sequence {
                    tunnel: w777 -> [w779]
                    tunnel: [w779] -> w772
                    tunnel: w776 -> [w780]
                    tunnel: w772 -> [w781]
                    frame #0 {
                      n369 = Wait (ms)(milliseconds to wait=u32 1) -> ()  [unwired: 1 out]
                    }
                    frame #1 {
                      n370 = Enqueue Element(queue=w781, element=w780) -> ()  [unwired: 2 in, 3 out]
                    }
                  }
                  n371 = case shown="False" w775 {
                    tunnel: [w782 w783] -> w774
                    tunnel: w773 -> [w782 w783]
                    frame False {
                    }
                    frame True {
                    }
                  }
                }
                frame Error {
                }
              }
              n372 = And(x=w713, y=w726) -> (x .and. y?=w723:bool)
            }
            n373 = global read "ActiveArray.vi" "Active"() -> (w693:bool[])
            n374 = Replace Array Subset(array=w693, new element=w695, index=w694) -> ()  [unwired: 1 out]
          }
        }
        n375 = Wait Until Next ms Multiple(millisecond multiple=u32 500) -> ()  [unwired: 1 out]
        n376 = local read "Exit"() -> (w659:bool)
      }
    }
    n377 = Wait Until Next ms Multiple(millisecond multiple=u32 100) -> ()  [unwired: 1 out]
  }
  "Exit 2" <- w38
  n378 = local write "Exit"(w37) -> ()
  n379 = while {
    tunnel: w37 -> [_]
    tunnel: w12 -> [w879]
    tunnel: w11 -> [w878]
    tunnel: w8 -> [w876]
    tunnel: w1 -> [w859]
    stop <- w948 stop-if-true
    w857 = FALSE
    # "I"
    # "Ewe"
    # "t"
    # "Ewe"
    # "I"
    # "t"
    n380 = local read "NoOfChannels"() -> (w853:i32)
    n381 = local read "ConfigTable"() -> (w855:T4)
    n382 = global read "ActiveArray.vi" "Active"() -> (w869:bool[])
    n383 = global read "StartStopPause.vi" "StartStopPauseArray1"() -> (w852:bool[][])
    n384 = global read "StartStopPause.vi" "StartStopPauseArray2"() -> (w851:bool[][])
    n385 = local write "WriteAll"(-1 ("WriteAll")) -> ()
    n386 = call "Display Message to User"("Enable"="stop") -> ("OK"=w848:bool)  [unwired: 9 in, 1 out]
    n387 = Index Array(array=w869, index="Show Instance") -> (element=→"Active":bool)
    n388 = global read "ActiveArray.vi" "Active"() -> (w884:bool[])
    n389 = local read "LiveViewData"() -> (w893:cluster{"JVData":sgl[][], "AgingData":sgl[][]}[])
    n390 = local read "Device Code"() -> (w938:i32)
    n391 = Stop(stop? (T)=w848) -> ()
    n392 = Insert Into Array(array=w852, new element=w851) -> (w850:bool[][])  [unwired: 2 in]
    n393 = case shown="True" "Activate Magic Control" {
      tunnel: [w950 w955] -> w854
      tunnel: w855 -> [w950 w956]
      tunnel: w853 -> [_ w958]
      tunnel: w850 -> [_ w957]
      frame False {
      }
      frame True {
        n394 = Index Array(array=w957, index (col) #1=0 ("disabled index (col)")) -> (element #1=w954:bool[], element #2=w953:bool[], element #3=w952:bool[])  [unwired: 5 in]
        n395 = for {
          N: w958 -> [_]
          tunnel: w956 -> [w968] mode=indexing
          tunnel: [w969] -> w955 mode=indexing
          tunnel: w954 -> [w962] mode=indexing
          tunnel: w953 -> [w963] mode=indexing
          tunnel: w952 -> [w964] mode=indexing
          n396 = Unbundle By Name(w968) -> ("StartCh"=w961:bool, "StopCh"=w960:bool, "PauseCh"=w959:bool)
          n397 = Or(x=w961, y=w962) -> (x .or. y?=w965:bool)
          n398 = Or(x=w960, y=w963) -> (x .or. y?=w966:bool)
          n399 = Or(x=w959, y=w964) -> (x .or. y?=w967:bool)
          n400 = Bundle By Name(cluster=w968, "StartCh"=w965, "StopCh"=w966, "PauseCh"=w967) -> (w969:T14)
        }
      }
    }
    n401 = for {
      N: w853 -> [_]
      tunnel: w854 -> [w1105] mode=indexing
      tunnel: [w1089] -> w875 mode=indexing
      tunnel: [w1102] -> w885 mode=indexing
      tunnel: w884 -> [w1098] mode=indexing
      tunnel: w879 -> [w1094] mode=indexing
      tunnel: w878 -> [w1093] mode=indexing
      tunnel: [w1080] -> w877
      tunnel: w876 -> [w1092] mode=indexing
      tunnel: [w1086] -> w872
      tunnel: w859 -> [w1084]
      tunnel: w857 -> [w1076]
      i -> [w1085]
      n402 = Unbundle By Name(w1105) -> ("StartCh"=w1109:bool, "PauseCh"=w1108:bool, "StopCh"=w1107:bool, "Status"=w1083:dbl, "CopyToAll"=w1088:bool)
      n403 = case shown="True" w1088 {
        tunnel: w1085 -> [_ w1111]
        tunnel: [w1110 w1111] -> w1087
        frame False {
          n404 = local read "WriteAll"() -> (w1110:i32)
        }
        frame True {
        }
      }
      n405 = Equal?(x=w1083, y=1.0) -> (x = y?=w1095:bool)
      n406 = local write "WriteAll"(w1087) -> ()
      n407 = case shown="True" w1109 {
        tunnel: w1105 -> [w1160 w1173]
        tunnel: [w1160 w1164] -> w1104
        tunnel: [w1159 w1166] -> w1097
        tunnel: w1098 -> [w1159 w1165]
        tunnel: w1094 -> [_ w1171]
        tunnel: w1093 -> [_ w1170]
        tunnel: w1092 -> [_ w1169]
        tunnel: w1085 -> [_ w1168]
        tunnel: w1084 -> [_ w1167]
        tunnel: [w1158 w1163] -> w1082
        tunnel: w1083 -> [w1158 w1162]
        tunnel: [w1157 w1161] -> w1077
        tunnel: w1076 -> [w1157 _]
        frame False {
        }
        frame True {
          w1161 = TRUE
          n408 = Unbundle By Name(w1173) -> ("Status"=w1172:dbl)
          n409 = case shown="0" w1172 {
            tunnel: w1173 -> [w1174 w1181 w1191]
            tunnel: [w1175 w1180 w1223] -> w1164
            tunnel: w1171 -> [_ _ w1208]
            tunnel: w1170 -> [_ _ w1205]
            tunnel: w1169 -> [_ _ w1201]
            tunnel: w1168 -> [_ _ w1199]
            tunnel: w1167 -> [_ w1187 w1196]
            tunnel: [w1178 TRUE ("new element/subarray") TRUE ("new element/subarray")] -> w1166
            tunnel: w1165 -> [w1178 _ _]
            tunnel: [w1177 w1179 w1188] -> w1163
            tunnel: w1162 -> [w1177 _ w1188]
            frame 1, Default {
              w1176 = FALSE ("StartCh")
              n410 = Bundle By Name(cluster=w1174, "StartCh"=w1176, "PauseCh"=w1176) -> (w1175:T14)
            }
            frame 2 {
              w1184 = FALSE ("StartCh")
              w1179 = u32 1 ("millisecond multiple")
              n411 = Unbundle By Name(w1181) -> ("Channel"=w1186:u8)
              n412 = call "StopChannel.vi"("Channel"=w1186, "ID"=w1187) -> ()  [unwired: 9 in, 1 out]
              n413 = Bundle By Name(cluster=w1181, "StatusStr"="running", "ColorInd"=TRUE, "Status"=w1179, "StartCh"=w1184, "PauseCh"=w1184) -> (w1180:T14)
            }
            frame 0 {
              w1195 = FALSE ("StartCh")
              n414 = Unbundle By Name(w1191) -> ("Channel"=w1197:u8, "name"=w1232:string)
              n415 = call "StopChannel.vi"("Channel"=w1197, "ID"=w1196) -> ()  [unwired: 9 in, 1 out]
              n416 = local read "Directory to save files"() -> (w1216:path)
              n417 = Add(x=u8 1, y=w1197) -> (x+y=w1198:u8)
              n418 = Get Date/Time In Seconds() -> (seconds since 1Jan1904=w1222:timestamp)
              n419 = Number To Decimal String(number=w1198) -> (decimal integer string=w1233:string)  [unwired: 1 in]
              n420 = Format Date/Time String(time format string (%c)="%y%m%d_%Hh_%Mm%Ss", seconds (now)=w1222) -> (date/time string=w1218:string)  [unwired: 1 in]
              n421 = Enqueue Element(queue=w1201, element=sgl[][] [[-1.0]]) -> ()  [unwired: 2 in, 3 out]
              n422 = Enqueue Element(queue=w1208, element=dbl[] [-100.0]) -> ()  [unwired: 2 in, 3 out]
              n423 = Enqueue Element(queue=w1205, element=dbl[] [-100.0]) -> ()  [unwired: 2 in, 3 out]
              n424 = Strip Path(path=w1216) -> ()  [unwired: 2 out]
              n425 = Concatenate Strings("Ch" ("string"), w1233, "_" ("string"), w1232) -> (w1203:string)
              n426 = Concatenate Strings(w1203, "_" ("string"), w1218) -> (w1220:string)
              n427 = local read "Channel Names"() -> (w1202:string[])
              n428 = Concatenate Strings(w1220, "_JVs.txt" ("string")) -> (w1225:string)
              n429 = Concatenate Strings(w1220, "_aging.txt" ("string")) -> (w1229:string)
              n430 = Concatenate Strings(w1220, "_JVmetrics.txt" ("string")) -> (w1226:string)
              n431 = Replace Array Subset(array=w1202, new element=w1203, index=w1199) -> (w1204:string[])
              n432 = Build Path(base path=w1216, name or relative path=w1226) -> (appended path=w1209:path)
              n433 = Build Path(base path=w1216, name or relative path=w1225) -> (appended path=w1224:path)
              n434 = Build Path(base path=w1216, name or relative path=w1229) -> (appended path=w1210:path)
              n435 = call-poly <vilib>:"Write Delimited Spreadsheet.vi"("file path (dialog if empty)"=w1210, "1D data"="HeaderAging", "append to file? (new file:F)"=FALSE ("append to file? (F)")) -> ()  [unwired: 11 in, 2 out]
              n436 = local write "Channel Names"(w1204) -> ()
              n437 = property on="Display Data for:" class="LstBox (strict)"("Item Names"=w1204) -> ()  [unwired: 2 in, 2 out]
              n438 = Bundle By Name(cluster=w1191, "StatusStr"="running", "ColorInd"=TRUE, "Status"=u32 1 ("millisecond multiple"), "StartCh"=w1195, "PauseCh"=w1195) -> (w1190:T14)
              n439 = Bundle By Name(cluster=w1190, "AgingFile"=w1210, "JVMetricsFile"=w1209, "JVFile"=w1224, "start time"=w1222) -> (w1223:T14)
              n440 = call-poly <vilib>:"Write Delimited Spreadsheet.vi"("file path (dialog if empty)"=w1209, "1D data"="HeaderJVMetrics", "append to file? (new file:F)"=FALSE ("append to file? (F)")) -> ()  [unwired: 11 in, 2 out]
            }
          }
          n441 = local write "WriteConfigTable"(w1161) -> ()
        }
      }
      n442 = Not(x=w1097) -> (.not. x?=w1099:bool)
      n443 = And(x=w1095, y=w1099) -> (x .and. y?=w1100:bool)
      n444 = Or(x=w1107, y=w1100) -> (x .or. y?=w1106:bool)
      n445 = case shown="True" w1108 {
        tunnel: w1104 -> [w1128 w1141]
        tunnel: w1082 -> [w1129 w1138]
        tunnel: [w1127 w1140] -> w1103
        tunnel: [w1126 w1142] -> w1101
        tunnel: w1097 -> [w1126 w1139]
        tunnel: [w1125 w1137] -> w1078
        tunnel: w1077 -> [w1124 w1136]
        frame False {
          n446 = case shown="0, Default" w1129 {
            tunnel: w1128 -> [w1131 w1134]
            tunnel: [w1131 w1133] -> w1127
            tunnel: [w1130 w1132] -> w1125
            tunnel: w1124 -> [w1130 _]
            frame 0, Default {
            }
            frame 2 {
              w1132 = TRUE
              n447 = Bundle By Name(cluster=w1134, "StartCh"=TRUE) -> (w1133:T14)
              n448 = local write "WriteConfigTable"(w1132) -> ()
            }
          }
        }
        frame True {
          n449 = case shown="0, Default" w1138 {
            tunnel: [w1147 FALSE ("new element/subarray") w1155] -> w1142
            tunnel: w1141 -> [w1145 w1150 w1156]
            tunnel: [w1144 w1149 w1156] -> w1140
            tunnel: w1139 -> [w1147 _ w1155]
            tunnel: [w1143 w1148 w1154] -> w1137
            tunnel: w1136 -> [_ _ w1154]
            frame 0, Default {
              w1143 = TRUE
              n450 = Bundle By Name(cluster=w1145, "PauseCh"=FALSE) -> (w1144:T14)
              n451 = local write "WriteConfigTable"(w1143) -> ()
            }
            frame 1 {
              w1148 = TRUE
              n452 = Bundle By Name(cluster=w1150, "Status"=u32 2 ("millisecond multiple"), "StatusStr"="halted") -> (w1149:T14)
              n453 = local write "WriteConfigTable"(w1148) -> ()
            }
            frame 2 {
            }
          }
        }
      }
      n454 = case shown="False" w1106 {
        tunnel: w1103 -> [w1114 w1119]
        tunnel: [w1114 w1118] -> w1090
        tunnel: [w1113 FALSE ("new element/subarray")] -> w1102
        tunnel: w1101 -> [w1113 _]
        tunnel: [w1112 TRUE ("new element/subarray")] -> w1079
        tunnel: w1078 -> [w1112 _]
        frame False {
        }
        frame True {
          w1120 = FALSE ("StartCh")
          n455 = Bundle By Name(cluster=w1119, "ColorInd"=FALSE, "Status"=u32 0 ("millisecond multiple"), "StopCh"=w1120, "StatusStr"="stopped", "PauseCh"=w1120) -> (w1118:T14)
          n456 = local write "WriteConfigTable"(TRUE) -> ()
        }
      }
      n457 = Bundle By Name(cluster=w1090, "CopyToAll"=FALSE) -> (w1089:T14)
      n458 = local read "WriteConfigTable"() -> (w1081:bool)
      n459 = local read "WriteAll"() -> (w1086:i32)
      n460 = Or(x=w1081, y=w1079) -> (x .or. y?=w1080:bool)
    }
    n461 = Index Array(array=w893, index="Show Instance") -> (element=w929:cluster{"JVData":sgl[][], "AgingData":sgl[][]})
    n462 = local read "ConfigTable"() -> (w901:T4)
    n463 = Unbundle By Name(w929) -> ("AgingData"=w902:sgl[][], "JVData"=w928:sgl[][])
    "ExchangeJVData" <- w928
    n464 = Index Array(array=w928, index (col)=3 ("Index")) -> (element=w941:sgl[])  [unwired: 1 in]
    n465 = Index Array(array=w928, index (col)=1 ("Index")) -> (element=w944:sgl[])  [unwired: 1 in]
    n466 = Index Array(array=w928, index (col)=2 ("Index")) -> (element=w942:sgl[])  [unwired: 1 in]
    n467 = Index Array(array=w928, index (col)=0 ("Index")) -> (element=w939:sgl[])  [unwired: 1 in]
    n468 = case shown="12, 16, 20, 21, 23, 27" w938 {
      tunnel: w944 -> [w1256 _]
      tunnel: w942 -> [w1255 w1259]
      tunnel: w941 -> [_ w1258]
      tunnel: w939 -> [w1257 w1260]
      tunnel: [w1257 w1260] -> w931
      tunnel: [w1256 w1259] -> w897
      tunnel: [w1255 w1258] -> w930
      frame 12, 16, 20, 21, 23, 27 {
      }
      frame Default {
      }
    }
    n469 = Array Size(array=w939) -> (size(s)=→"Number of points":i32)
    n470 = Index Array(array=w901, index="Show Instance") -> (element=w900:T14)
    n471 = Unbundle By Name(w900) -> ("Channel"=w870:u8, "ActiveArea cm2"=w888:dbl, "StatusStr"=→"Status":string)
    n472 = Increment(x=w870) -> (x+1=→"Channel":u8)
    n473 = Multiply(x=w897, y=1000) -> (x*y=w899:sgl[])
    n474 = Divide(x=w899, y=w888) -> (x/y=w896:dbl[])
    n475 = case shown="\"P(V)\"" "Draw 2" {
      tunnel: w931 -> [_ _ w1249 w1254]
      tunnel: w896 -> [w1235 w1240 _ w1253]
      tunnel: [w1234 w1239 w1245 w1250] -> w937
      tunnel: "Potential (V)" ("Y Scale.Name Label.Text") -> [w1238 w1243 w1248 _]
      tunnel: "Current density (mA/cm2)" ("Y Scale.Name Label.Text") -> [w1237 _ _ w1252]
      tunnel: [w1237 w1242 w1248 w1252] -> w935
      tunnel: [w1238 w1243 w1247 w1251] -> w934
      tunnel: "Time (s)" ("Y Scale.Name Label.Text") -> [_ _ w1247 w1251]
      tunnel: w930 -> [w1236 w1241 w1246 _]
      tunnel: "Power (W)" ("Y Scale.Name Label.Text") -> [_ w1242 _ _]
      frame "J(V)" {
        n476 = Bundle("JVData"=w1236, w1235) -> (w1234:cluster{"JVData":sgl[], dbl[]})  [unwired: 1 in]
      }
      frame "P(V)" {
        n477 = Multiply(x=w1240, y=w1241) -> (x*y=w1244:dbl[])
        n478 = Bundle("JVData"=w1241, w1244) -> (w1239:cluster{"JVData":sgl[], dbl[]})  [unwired: 1 in]
      }
      frame "V(t)", Default {
        n479 = Bundle("JVData"=w1249, "JVData"=w1246) -> (w1245:cluster{"JVData":sgl[], "JVData":sgl[]})  [unwired: 1 in]
      }
      frame "I(t)" {
        n480 = Bundle("JVData"=w1254, w1253) -> (w1250:cluster{"JVData":sgl[], dbl[]})  [unwired: 1 in]
      }
    }
    "XY Graph" <- w937
    n481 = property on="XY Graph" class="XYGraph (strict)"("Y Scale.Name Label.Text"=w935) -> ()  [unwired: 2 in, 2 out]
    n482 = property on="XY Graph" class="XYGraph (strict)"("X Scale.Name Label.Text"=w934) -> ()  [unwired: 2 in, 2 out]
    n483 = Index Array(array=w902, index (col)=2 ("indice désactivé (col)")) -> (element=w926:sgl[])  [unwired: 1 in]
    n484 = Multiply(x=w926, y=1000) -> (x*y=w924:sgl[])
    n485 = Index Array(array=w902, index (col)=1 ("Index")) -> (element=w918:sgl[])  [unwired: 1 in]
    n486 = Index Array(array=w902, index (col)=0 ("Index")) -> (element=w916:sgl[])  [unwired: 1 in]
    n487 = Divide(x=w924, y=w888) -> (x/y=w927:dbl[])
    n488 = Multiply(x=w918, y=w927) -> (x*y=w919:dbl[])
    n489 = Array Size(array=w916) -> (size(s)=w914:i32)
    "Number of points" <- w914
    n490 = case shown="\"V(t)\", Default" "Draw" {
      tunnel: w916 -> [w1065 w1066 w1073]
      tunnel: [w1062 w1067 w1071] -> w912
      tunnel: "Potential (V)" ("Y Scale.Name Label.Text") -> [w1064 _ _]
      tunnel: "Current density (mA/cm2)" ("Y Scale.Name Label.Text") -> [_ w1070 _]
      tunnel: [w1064 w1070 w1074] -> w908
      tunnel: [w1063 w1069 w1075] -> w909
      tunnel: "Time (s)" ("Y Scale.Name Label.Text") -> [w1063 w1069 w1075]
      tunnel: w918 -> [w1061 _ _]
      tunnel: w927 -> [_ w1068 _]
      tunnel: "Power (mW/cm2)" ("Y Scale.Name Label.Text") -> [_ _ w1074]
      tunnel: w919 -> [_ _ w1072]
      frame "V(t)", Default {
        n491 = Bundle("AgingData"=w1065, "AgingData"=w1061) -> (w1062:cluster{"AgingData":sgl[], "AgingData":sgl[]})  [unwired: 1 in]
      }
      frame "I(t)" {
        n492 = Bundle("AgingData"=w1066, w1068) -> (w1067:cluster{"AgingData":sgl[], dbl[]})  [unwired: 1 in]
      }
      frame "P(t)" {
        n493 = Bundle("AgingData"=w1073, w1072) -> (w1071:cluster{"AgingData":sgl[], dbl[]})  [unwired: 1 in]
      }
    }
    "XY Graph 2" <- w912
    n494 = Subtract(x=w914, y=1) -> (x-y=w917:i32)
    n495 = Index Array(array=w916, index=w917) -> (element=→"time (s)":sgl)
    n496 = Index Array(array=w918, index=w917) -> (element=→"V (V)":sgl)
    n497 = Index Array(array=w927, index=w917) -> (element=→"J (mA/cm2)":dbl)
    n498 = Index Array(array=w919, index=w917) -> (element=→"P (mW/cm2)":dbl)
    n499 = Wait Until Next ms Multiple(millisecond multiple=u32 500) -> ()  [unwired: 1 out]
    n500 = local read "Channel Names"() -> (w858:string[])
    n501 = property on="XY Graph 2" class="XYGraph (strict)"("X Scale.Name Label.Text"=w909) -> ()  [unwired: 2 in, 2 out]
    n502 = property on="XY Graph 2" class="XYGraph (strict)"("Y Scale.Name Label.Text"=w908) -> ()  [unwired: 2 in, 2 out]
    n503 = case shown="0, Default" w872 {
      tunnel: w875 -> [w990 w1001]
      tunnel: [w991 w1001] -> w874
      tunnel: w872 -> [w989 _]
      frame 0, Default {
        n504 = Index Array(array=w990, index=w989) -> (element=w988:T14)
        n505 = local write "WriteConfigTable"(TRUE) -> ()
        n506 = for {
          tunnel: w990 -> [w996] mode=indexing
          tunnel: [w994] -> w991 mode=indexing
          tunnel: w988 -> [w997]
          n507 = Unbundle By Name(w996) -> ("name"=w992:string, "Channel"=w993:u8, "Status"=w998:dbl)
          n508 = case shown="1, Default" w998 {
            tunnel: w997 -> [w999 _]
            tunnel: [w999 w1000] -> w995
            tunnel: w996 -> [_ w1000]
            frame 0 {
            }
            frame 1, Default {
            }
          }
          n509 = Bundle By Name(cluster=w995, "name"=w992, "Channel"=w993) -> (w994:T14)
        }
      }
      frame -1 {
      }
    }
    n510 = case shown="True" "StartCh" {
      tunnel: w853 -> [_ w1056]
      tunnel: w874 -> [w1052 w1055]
      tunnel: [w1052 w1054] -> w883
      frame False {
      }
      frame True {
        n511 = for {
          N: w1056 -> [_]
          tunnel: w1055 -> [w1059] mode=indexing
          tunnel: [w1058] -> w1054 mode=indexing
          n512 = Bundle By Name(cluster=w1059, "StartCh"=TRUE) -> (w1058:T14)
        }
        n513 = local write "WriteConfigTable"(TRUE) -> ()
        n514 = local write "StartCh"(FALSE ("StartCh")) -> ()
      }
    }
    n515 = case shown="True" "PauseCh" {
      tunnel: w853 -> [w1033 w1048]
      tunnel: w883 -> [w1032 w1046]
      tunnel: [w1031 w1045] -> w882
      frame False {
        n516 = local read "AllPaused"() -> (w1034:bool)
        n517 = case shown="True" w1034 {
          tunnel: w1033 -> [_ w1039]
          tunnel: w1032 -> [w1035 w1038]
          tunnel: [w1035 w1037] -> w1031
          frame False {
          }
          frame True {
            n518 = for {
              N: w1039 -> [_]
              tunnel: w1038 -> [w1042] mode=indexing
              tunnel: [w1041] -> w1037 mode=indexing
              n519 = Bundle By Name(cluster=w1042, "PauseCh"=FALSE ("StartCh")) -> (w1041:T14)
            }
            n520 = local write "WriteConfigTable"(TRUE) -> ()
            n521 = local write "AllPaused"(FALSE ("StartCh")) -> ()
          }
        }
      }
      frame True {
        n522 = for {
          N: w1048 -> [_]
          tunnel: w1046 -> [w1050] mode=indexing
          tunnel: [w1049] -> w1045 mode=indexing
          n523 = Bundle By Name(cluster=w1050, "PauseCh"=TRUE ("StartCh")) -> (w1049:T14)
        }
        n524 = local write "WriteConfigTable"(TRUE) -> ()
        n525 = local write "AllPaused"(TRUE ("StartCh")) -> ()
      }
    }
    n526 = case shown="True" "StopCh" {
      tunnel: w853 -> [_ w1026]
      tunnel: w882 -> [w1022 w1025]
      tunnel: [w1022 w1024] -> w864
      frame False {
      }
      frame True {
        n527 = for {
          N: w1026 -> [_]
          tunnel: w1025 -> [w1029] mode=indexing
          tunnel: [w1028] -> w1024 mode=indexing
          n528 = Bundle By Name(cluster=w1029, "StopCh"=TRUE ("StartCh")) -> (w1028:T14)
        }
        n529 = local write "StopCh"(FALSE ("StartCh")) -> ()
        n530 = local write "WriteConfigTable"(TRUE) -> ()
      }
    }
    n531 = case shown="True" "JVstandard" {
      tunnel: w853 -> [_ w1020]
      tunnel: [w1016 w1017] -> w880
      tunnel: w864 -> [w1016 _]
      frame False {
      }
      frame True {
        n532 = local write "WriteConfigTable"(TRUE) -> ()
        n533 = for {
          N: w1020 -> [_]
          tunnel: [w1021] -> w1017 mode=indexing
          tunnel: "JVStandard" -> [w1021] mode=indexing
        }
      }
    }
    n534 = case shown="True" "Agingstandard" {
      tunnel: w853 -> [_ w1014]
      tunnel: [w1010 w1011] -> w881
      tunnel: w880 -> [w1010 _]
      frame False {
      }
      frame True {
        n535 = local write "WriteConfigTable"(TRUE) -> ()
        n536 = for {
          N: w1014 -> [_]
          tunnel: [w1015] -> w1011 mode=indexing
          tunnel: "AgingStandard" -> [w1015] mode=indexing
        }
      }
    }
    n537 = case shown="True" "JVMPPst" {
      tunnel: w853 -> [_ w1008]
      tunnel: [w1004 w1006] -> w860
      tunnel: w881 -> [w1004 _]
      frame False {
      }
      frame True {
        n538 = for {
          N: w1008 -> [_]
          tunnel: [w1009] -> w1006 mode=indexing
          tunnel: "JV Stabilized MPP Standard" -> [w1009] mode=indexing
        }
        n539 = local write "WriteConfigTable"(TRUE) -> ()
      }
    }
    n540 = case shown="True" "Open Button" {
      tunnel: [w970 w972] -> w862
      tunnel: [w971 w976] -> w861
      tunnel: w860 -> [w971 w974]
      frame False {
        n541 = local read "WriteConfigTable"() -> (w970:bool)
      }
      frame True {
        n542 = Open/Create/Replace Datalog(5:w974) -> (0:w977:errorcluster, 1:w973:bool, 3:w975:refnum<k1>)  [unwired: 3 in, 2 out]
        n543 = Read Datalog(4:w977, 7:w975) -> (0:w979:errorcluster, 2:w976:T20, 3:w978:refnum<k1>)  [unwired: 1 in]
        n544 = Not(x=w973) -> (.not. x?=w972:bool)
        n545 = Close File(refnum=w978, error in=w979) -> ()  [unwired: 2 out]
      }
    }
    n546 = case shown="True" "Save As Button" {
      tunnel: w864 -> [_ w981]
      frame False {
      }
      frame True {
        n547 = Open/Create/Replace Datalog(5:w981, 10:T19."replace or create with confirmation" ("operation (0:open)")) -> (0:w986:errorcluster, 3:w983:refnum<k1>)  [unwired: 4 in, 1 out]
        n548 = Write Datalog(4:w986, 6:w981, 7:w983) -> (0:w985:errorcluster, 3:w984:refnum<k1>)
        n549 = Close File(refnum=w984, error in=w985) -> (error out=w980:errorcluster)  [unwired: 1 out]
        n550 = call <vilib>:"Simple Error Handler.vi"("error in (no error)"=w980) -> ()  [unwired: 4 in, 5 out]
      }
    }
    n551 = local read "Exit"() -> (w948:bool)
    n552 = case shown="True" w862 {
      tunnel: w861 -> [_ w1003]
      frame False {
      }
      frame True {
        n553 = local write "ConfigTable"(w1003) -> ()
      }
    }
    n554 = case shown="True" w877 {
      tunnel: w885 -> [_ w1002]
      frame False {
      }
      frame True {
        n555 = global write "ActiveArray.vi" "Active"(w1002) -> ()
      }
    }
    n556 = property on="Display Data for:" class="LstBox (strict)"("Item Names"=w858) -> ()  [unwired: 2 in, 2 out]
    "WriteConfigTable" <- w857
  }
  n557 = while {
    stop <- w1284 stop-if-true
    w1280 = T5 []
    n558 = Array Size(array="Display Data for:") -> (size(s)=w1282:i32)
    n559 = for {
      N: w1282 -> [_]
      tunnel: "Display Data for:" -> [w1355] mode=indexing
      shift-right: [w1411] -> w1264
      shift-left: w1280 -> [w1412]
      shift-right: [w1408] -> w1263
      shift-left: w1280 -> [w1409]
      shift-right: [w1406] -> w1265
      shift-left: w1280 -> [w1405]
      shift-right: [w1403] -> w1267
      shift-left: w1280 -> [w1402]
      shift-right: [w1401] -> w1269
      shift-left: w1280 -> [w1400]
      shift-right: [w1396] -> w1271
      shift-left: w1280 -> [w1395]
      shift-right: [w1382] -> w1279
      shift-left: w1280 -> [w1381]
      shift-right: [w1377] -> w1276
      shift-left: sgl[][] [] -> [w1368]
      i -> [w1347]
      # "Ewe"
      # "I"
      # "t"
      n560 = local read "ChannelData"() -> (w1421:T2)
      n561 = local read "Channel Names"() -> (w1393:string[])
      n562 = local read "ChannelAgingData"() -> (w1392:cluster{"AgingData":sgl[][]}[])
      n563 = Index Array(array=w1421, index=w1355) -> (element=w1420:cluster{"JV metrics":sgl[][], "JVData":sgl[][]})
      n564 = Index Array(array="Plot Color", index=w1355) -> (element=w1345:u32)
      n565 = Index Array(array="Point Style", index=w1355) -> (element=w1346:u8)
      n566 = Index Array(array=w1393, index=w1355) -> (element=w1354:string)
      n567 = Unbundle By Name(w1420) -> ("JV metrics"=w1378:sgl[][], "JVData"=w1383:sgl[][])
      n568 = Index Array(array=w1392, index=w1355) -> (element=w1417:cluster{"AgingData":sgl[][]})
      n569 = Index Array(array=w1383, index (col) #1=0 ("Index"), index (col) #2=1 ("Index"), index (col) #3=2 ("Index")) -> (element #1=w1360:sgl[], element #2=w1359:sgl[], element #3=w1358:sgl[])  [unwired: 3 in]
      n570 = property on="XY Graph 9" class="XYGraph (strict)"("Active Plot"=w1347, "Plot.Plot Name"=w1354, "Plot.Plot Color"=w1345, "Plot.Point Style"=w1346, "Plot.Fill/Pt. Color"=w1345) -> ()  [unwired: 2 in, 2 out]
      n571 = Array Size(array=w1378) -> (size(s)=w1379:i32[])
      n572 = Unbundle By Name(w1417) -> ("AgingData"=w1416:sgl[][])
      n573 = Index Array(array=w1379) -> (element=w1375:i32)  [unwired: 1 in]
      n574 = Index Array(array=w1378, index (col)=2) -> (element=w1422:sgl[])  [unwired: 1 in]
      n575 = Index Array(array=w1378, index (col)=0 ("index")) -> (element=w1399:sgl[])  [unwired: 1 in]
      n576 = Index Array(array=w1378, index (col)=1 ("disabled index (col)")) -> (element=w1428:sgl[])  [unwired: 1 in]
      n577 = Index Array(array=w1378, index (col)=3) -> (element=w1423:sgl[])  [unwired: 1 in]
      n578 = Index Array(array=w1378, index (col)=4) -> (element=w1424:sgl[])  [unwired: 1 in]
      n579 = Index Array(array=w1378, index (col)=7) -> (element=w1419:sgl[])  [unwired: 1 in]
      n580 = Index Array(array=w1416, index (col)=0 ("index")) -> (element=w1398:sgl[])  [unwired: 1 in]
      n581 = Index Array(array=w1416, index (col)="Draw 3") -> (element=w1414:sgl[])  [unwired: 1 in]
      n582 = Subtract(x=w1375, y=1) -> (x-y=w1376:i32)
      n583 = control-ref of="XY Graph 8"() -> (w1353:refnum<vi>)
      n584 = property class="XYGraph (strict)"(reference=w1353, "Active Plot"=w1347, "Plot.Plot Color"=w1345, "Plot.Point Style"=w1346, "Plot.Fill/Pt. Color"=w1345) -> ()  [unwired: 1 in, 2 out]
      n585 = control-ref of="XY Graph 7"() -> (w1350:refnum<vi>)
      n586 = property class="XYGraph (strict)"(reference=w1350, "Active Plot"=w1347, "Plot.Plot Color"=w1345, "Plot.Point Style"=w1346, "Plot.Fill/Pt. Color"=w1345) -> ()  [unwired: 1 in, 2 out]
      n587 = Bundle("JV metrics"=w1399, "JV metrics"=w1424) -> (w1410:cluster{"JV metrics":sgl[], "JV metrics":sgl[]})  [unwired: 1 in]
      n588 = Bundle("JV metrics"=w1399, "JV metrics"=w1419) -> (w1413:cluster{"JV metrics":sgl[], "JV metrics":sgl[]})  [unwired: 1 in]
      n589 = Bundle("JV metrics"=w1399, "JV metrics"=w1428) -> (w1394:cluster{"JV metrics":sgl[], "JV metrics":sgl[]})  [unwired: 1 in]
      n590 = Bundle("JV metrics"=w1399, "JV metrics"=w1422) -> (w1404:cluster{"JV metrics":sgl[], "JV metrics":sgl[]})  [unwired: 1 in]
      n591 = Bundle("JV metrics"=w1399, "JV metrics"=w1423) -> (w1407:cluster{"JV metrics":sgl[], "JV metrics":sgl[]})  [unwired: 1 in]
      n592 = Index Array(array=w1378, index (row)=w1376) -> (element=w1367:sgl[])  [unwired: 1 in]
      n593 = Build Array (concatenate)(w1402, w1404) -> (w1403:T5)
      n594 = Bundle("AgingData"=w1398, "AgingData"=w1414) -> (w1397:cluster{"AgingData":sgl[], "AgingData":sgl[]})  [unwired: 1 in]
      n595 = Build Array (concatenate)(w1405, w1407) -> (w1406:T5)
      n596 = Build Array (concatenate)(w1409, w1410) -> (w1408:T5)
      n597 = Array Subset(array=w1367, index=0, length=5) -> (w1366:sgl[])
      n598 = Build Array (concatenate)(w1412, w1413) -> (w1411:T5)
      n599 = Build Array (concatenate)(w1400, w1394) -> (w1401:T5)
      n600 = Build Array (concatenate)(w1395, w1397) -> (w1396:cluster{"AgingData":sgl[], "AgingData":sgl[]}[])
      n601 = Array Subset(array=w1367, index=7, length=4) -> (w1365:sgl[])
      n602 = control-ref of="XY Graph 6"() -> (w1352:refnum<vi>)
      n603 = property class="XYGraph (strict)"(reference=w1352, "Active Plot"=w1347, "Plot.Plot Color"=w1345, "Plot.Point Style"=w1346, "Plot.Fill/Pt. Color"=w1345) -> ()  [unwired: 1 in, 2 out]
      n604 = control-ref of="XY Graph 5"() -> (w1351:refnum<vi>)
      n605 = property class="XYGraph (strict)"(reference=w1351, "Active Plot"=w1347, "Plot.Plot Color"=w1345, "Plot.Point Style"=w1346, "Plot.Fill/Pt. Color"=w1345) -> ()  [unwired: 1 in, 2 out]
      n606 = case shown="\"J(V)\"" "Selected to draw" {
        tunnel: w1360 -> [_ _ _ _ _ w1465 w1470]
        tunnel: w1358 -> [w1432 w1440 w1443 w1449 w1457 _ w1469]
        tunnel: [w1431 w1441 w1447 w1448 w1456 w1461 w1466] -> w1380
        tunnel: "Potential (V)" ("Y Scale.Name Label.Text") -> [w1435 w1436 w1444 w1452 w1460 w1464 _]
        tunnel: "Current density (mA/cm2)" ("Y Scale.Name Label.Text") -> [w1434 w1437 w1445 _ _ _ w1468]
        tunnel: [w1434 w1437 w1445 w1451 w1459 w1464 w1468] -> w1389
        tunnel: [w1435 w1436 w1444 w1452 w1460 w1463 w1467] -> w1388
        tunnel: "Time (s)" ("Y Scale.Name Label.Text") -> [_ _ _ _ _ w1463 w1467]
        tunnel: w1359 -> [w1433 w1438 w1446 w1450 w1458 w1462 _]
        tunnel: "Power (mW/cm2)" ("Y Scale.Name Label.Text") -> [_ _ _ w1451 w1459 _ _]
        frame "J(V)" {
          n607 = Bundle("JVData"=w1433, "JVData"=w1432) -> (w1431:cluster{"JVData":sgl[], "JVData":sgl[]})  [unwired: 1 in]
        }
        frame "-J(V)" {
          n608 = Negate(x=w1440) -> (-x=w1439:sgl[])
          n609 = Bundle("JVData"=w1438, w1439) -> (w1441:cluster{"JVData":sgl[], sgl[]})  [unwired: 1 in]
        }
        frame "abs J(V)" {
          n610 = Absolute Value(x=w1443) -> (abs(x)=w1442:sgl[])
          n611 = Bundle("JVData"=w1446, w1442) -> (w1447:cluster{"JVData":sgl[], sgl[]})  [unwired: 1 in]
        }
        frame "P(V)" {
          n612 = Multiply(x=w1449, y=w1450) -> (x*y=w1453:sgl[])
          n613 = Bundle("JVData"=w1450, w1453) -> (w1448:cluster{"JVData":sgl[], sgl[]})  [unwired: 1 in]
        }
        frame "-P(V)" {
          n614 = Multiply(x=w1457, y=w1458) -> (x*y=w1455:sgl[])
          n615 = Negate(x=w1455) -> (-x=w1454:sgl[])
          n616 = Bundle("JVData"=w1458, w1454) -> (w1456:cluster{"JVData":sgl[], sgl[]})  [unwired: 1 in]
        }
        frame "V(t)", Default {
          n617 = Bundle("JVData"=w1465, "JVData"=w1462) -> (w1461:cluster{"JVData":sgl[], "JVData":sgl[]})  [unwired: 1 in]
        }
        frame "I(t)" {
          n618 = Bundle("JVData"=w1470, "JVData"=w1469) -> (w1466:cluster{"JVData":sgl[], "JVData":sgl[]})  [unwired: 1 in]
        }
      }
      n619 = Index Array(array=w1367, index=11) -> (element=w1364:sgl)
      n620 = Build Array (concatenate)(w1366, w1365, w1364) -> (w1363:sgl[])
      n621 = control-ref of="XY Graph 4"() -> (w1349:refnum<vi>)
      n622 = property class="XYGraph (strict)"(reference=w1349, "Active Plot"=w1347, "Plot.Plot Color"=w1345, "Plot.Point Style"=w1346, "Plot.Fill/Pt. Color"=w1345) -> ()  [unwired: 1 in, 2 out]
      n623 = control-ref of="XY Graph 3"() -> (w1348:refnum<vi>)
      n624 = property class="XYGraph (strict)"(reference=w1348, "Active Plot"=w1347, "Plot.Plot Color"=w1345, "Plot.Point Style"=w1346, "Plot.Fill/Pt. Color"=w1345) -> ()  [unwired: 1 in, 2 out]
      n625 = property on="XY Graph 9" class="XYGraph (strict)"("Y Scale.Name Label.Text"=w1389) -> ()  [unwired: 2 in, 2 out]
      n626 = property on="XY Graph 9" class="XYGraph (strict)"("X Scale.Name Label.Text"=w1388) -> ()  [unwired: 2 in, 2 out]
      n627 = Build Array (concatenate)(w1368, w1363) -> (w1377:sgl[][])
      n628 = Build Array (concatenate)(w1381, w1380) -> (w1382:cluster{"JVData":sgl[], "JVData":sgl[]}[])
    }
    "XY Graph 3" <- w1269
    "XY Graph 4" <- w1267
    "XY Graph 5" <- w1265
    "XY Graph 6" <- w1263
    "XY Graph 7" <- w1264
    "XY Graph 8" <- w1271
    "XY Graph 9" <- w1279
    "JVParametersLastJV" <- w1276
    n629 = Array Size(array=w1279) -> (size(s)=w1278:i32)
    n630 = Array Size(array=w1276) -> (size(s)=w1275:i32[])
    n631 = Index Array(array=w1275) -> (element=w1274:i32)  [unwired: 1 in]
    n632 = case shown="True" "FitCurves" {
      tunnel: w1271 -> [_ w1290]
      frame False {
      }
      frame True {
        n633 = call "EasyFitTransients.vi"("InputData"=w1290) -> ()  [unwired: 11 in]
      }
    }
    n634 = property on="XY Graph 9" class="XYGraph (strict)"("LegNumRows"=w1278) -> ()  [unwired: 2 in, 2 out]
    n635 = case shown="True" "FitCurves 6" {
      tunnel: w1264 -> [_ w1285]
      frame False {
      }
      frame True {
        n636 = call "EasyFitTransients.vi"("InputData"=w1285) -> ()  [unwired: 11 in]
      }
    }
    n637 = property on="JVParametersLastJV" class="Arr (strict)"("Number of Rows"=w1274) -> ()  [unwired: 2 in, 2 out]
    n638 = case shown="True" "FitCurves 2" {
      tunnel: w1269 -> [_ w1289]
      frame False {
      }
      frame True {
        n639 = call "EasyFitTransients.vi"("InputData"=w1289) -> ()  [unwired: 11 in]
      }
    }
    n640 = case shown="True" "FitCurves 5" {
      tunnel: w1263 -> [_ w1286]
      frame False {
      }
      frame True {
        n641 = call "EasyFitTransients.vi"("InputData"=w1286) -> ()  [unwired: 11 in]
      }
    }
    n642 = case shown="True" "FitCurves 4" {
      tunnel: w1265 -> [_ w1287]
      frame False {
      }
      frame True {
        n643 = call "EasyFitTransients.vi"("InputData"=w1287) -> ()  [unwired: 11 in]
      }
    }
    n644 = case shown="True" "FitCurves 3" {
      tunnel: w1267 -> [_ w1288]
      frame False {
      }
      frame True {
        n645 = call "EasyFitTransients.vi"("InputData"=w1288) -> ()  [unwired: 11 in]
      }
    }
    n646 = case shown="True" "ExportAgingToExcel" {
      tunnel: w1271 -> [_ w1309]
      tunnel: w1263 -> [_ w1303]
      tunnel: w1269 -> [_ w1302]
      tunnel: w1267 -> [_ w1301]
      tunnel: w1265 -> [_ w1300]
      tunnel: w1264 -> [_ w1299]
      frame False {
      }
      frame True {
        n647 = for {
          tunnel: w1309 -> [w1343] mode=indexing
          shift-right: [w1336] -> w1305
          shift-left: string[] [] -> [w1340]
          shift-right: [w1337] -> w1306
          shift-left: string[][] [] -> [w1338]
          tunnel: w1303 -> [w1331] mode=indexing
          tunnel: w1302 -> [w1329] mode=indexing
          tunnel: w1301 -> [w1328] mode=indexing
          tunnel: w1300 -> [w1326] mode=indexing
          tunnel: w1299 -> [w1327] mode=indexing
          shift-right: [w1323] -> w1297
          shift-left: string[][] [] -> [w1322]
          i -> [w1342]
          n648 = Unbundle(w1327) -> ("JV metrics"=w1325:sgl[])  [unwired: 1 out]
          n649 = Unbundle(w1343) -> ("JV metrics"=w1333:sgl[], "JV metrics"=w1335:sgl[])
          n650 = Unbundle(w1328) -> ("JV metrics"=w1318:sgl[])  [unwired: 1 out]
          n651 = Unbundle(w1331) -> ("JV metrics"=w1330:sgl[], "JV metrics"=w1316:sgl[])
          n652 = Unbundle(w1329) -> ("JV metrics"=w1319:sgl[])  [unwired: 1 out]
          n653 = Unbundle(w1326) -> ("JV metrics"=w1317:sgl[])  [unwired: 1 out]
          n654 = property on="XY Graph 9" class="XYGraph (strict)"("Active Plot"=w1342) -> ("Plot.Plot Name"=w1341:string)  [unwired: 2 in, 2 out]
          n655 = Number To Exponential String(number=w1333) -> (E-format string=w1332:string[])  [unwired: 3 in]
          n656 = Number To Exponential String(number=w1335) -> (E-format string=w1334:string[])  [unwired: 3 in]
          n657 = Build Array(w1330, w1319, w1318, w1317, w1316, w1325) -> (w1324:sgl[][])
          n658 = Number To Exponential String(number=w1324) -> (E-format string=w1321:string[][])  [unwired: 3 in]
          n659 = Build Array (concatenate)(w1338, w1332, w1334, string[] [] ("element")) -> (w1337:string[][])
          n660 = Build Array (concatenate)(w1340, w1341) -> (w1336:string[])
          n661 = Insert Into Array(array=w1322, new element #1=w1321, new element #2=string[] [] ("element")) -> (w1323:string[][])  [unwired: 2 in]
        }
        n662 = local read "Draw 3"() -> (w1291:T7)
        n663 = Transpose 2D Array(2D array=w1306) -> (transposed array=w1304:string[][])
        n664 = case shown="\"Temp C\"" w1291 {
          tunnel: ["P (mW/cm2)" "V (V)" "Int (suns)" "J mA/cm2" "Temp (C)" "time (h)"] -> w1294
          frame "P mW/cm2", Default {
          }
          frame "V V" {
          }
          frame "Int suns" {
          }
          frame "J mA/cm2" {
          }
          frame "Temp C" {
          }
          frame "t h" {
          }
        }
        n665 = Transpose 2D Array(2D array=w1297) -> (transposed array=w1296:string[][])
        n666 = Build Array("time (h)", w1294, " ") -> (w1292:string[])
        n667 = call "ExportAgingDataToExcel.vi"("AgingData"=w1304, "HeaderAging"=w1292, "DeviceNames"=w1305, "JVMetricsData"=w1296) -> ()  [unwired: 1 in]
      }
    }
    n668 = local read "Exit"() -> (w1284:bool)
    n669 = Wait Until Next ms Multiple(millisecond multiple=u32 1000) -> ()  [unwired: 1 out]
  }
  n670 = call "disconnect.vi"("error in (no error)"=w36, "ID"=w31) -> ()  [unwired: 9 in, 1 out]
  n671 = while {
    stop <- w1472 stop-if-true
    n672 = case shown="True" "RestoreLastAutoSave" {
      frame False {
      }
      frame True {
        n673 = flat-sequence {
          frame #0 {
            n674 = control-ref of="This VI"() -> (w1484:refnum<vi>)
            n675 = property class="VI"(reference=w1484) -> ("Panel"=w1483:refnum<vi>)  [unwired: 1 in, 2 out]
            n676 = property on="Tab Control" class="TabCtl (strict)"() -> ("Pages"=w1478:refnum<vi>[])  [unwired: 2 in, 2 out]
            n677 = property class="Pnl"(reference=w1483) -> ("Controls[]"=w1477:refnum<vi>[])  [unwired: 1 in, 2 out]
            n678 = for {
              tunnel: [w1488] -> _ mode=indexing
              tunnel: w1478 -> [w1488] mode=indexing
              shift-right: [w1485] -> w1476
              shift-left: w1477 -> [w1487]
              n679 = property class="Page"(reference=w1488) -> ("Controls on Page[]"=w1486:refnum<vi>[])  [unwired: 1 in, 2 out]
              n680 = Insert Into Array(array=w1487, new element=w1486) -> (w1485:refnum<vi>[])  [unwired: 1 in]
            }
            n681 = for {
              tunnel: w1476 -> [w1497] mode=indexing
              tunnel: [w1496] -> w1480 mode=indexing
              tunnel: [w1495] -> w1481
              tunnel: [w1493] -> w1475 mode=indexing
              i -> [w1495]
              n682 = property class="Ctl"(reference=w1497) -> ("Label.Text"=w1493:string)  [unwired: 1 in, 2 out]
              n683 = property class="Ctl"(reference=w1497) -> ("Value"=w1494:variant)  [unwired: 1 in, 2 out]
              n684 = Variant To Flattened String(Variant=w1494) -> (1:w1496:i16[])  [unwired: 1 out]
            }
            "Array 2" <- w1475
            n685 = local read "autosave file"() -> (w1479:path)
            n686 = Read from Text File(file (use dialog)=w1479, count=w1481) -> (text=w1482:string[])  [unwired: 2 in, 3 out]
            n687 = for {
              tunnel: w1476 -> [w1492] mode=indexing
              tunnel: w1480 -> [w1491] mode=indexing
              tunnel: w1482 -> [w1489] mode=indexing
              n688 = Flattened String To Variant(6:w1489, 7:w1491) -> (3:w1490:variant)  [unwired: 1 in, 1 out]
              n689 = property class="Ctl"(reference=w1492, "Value"=w1490) -> ()  [unwired: 1 in, 2 out]
            }
            n690 = Wait (ms)(milliseconds to wait=u32 5000) -> ()  [unwired: 1 out]
          }
          frame #1 {
            n691 = for {
              N: 5 -> [_]
              n692 = local read "ConfigTable"() -> (w1503:T4)
              n693 = for {
                tunnel: w1503 -> [w1505] mode=indexing
                tunnel: [w1504] -> w1502 mode=indexing
                n694 = Unbundle By Name(w1505) -> ("ColorInd"=w1504:bool)
              }
              n695 = global write "ActiveArray.vi" "Active"(w1502) -> ()
              n696 = Wait Until Next ms Multiple(millisecond multiple=u32 20) -> ()  [unwired: 1 out]
            }
            n697 = local read "Channel Names"() -> (w1500:string[])
            n698 = property on="Display Data for:" class="LstBox (strict)"("Item Names"=w1500) -> ()  [unwired: 2 in, 2 out]
            n699 = local write "RestoreLastAutoSave"(FALSE) -> ()
          }
        }
      }
    }
    n700 = local read "Exit"() -> (w1472:bool)
    n701 = Wait Until Next ms Multiple(millisecond multiple=u32 1000) -> ()  [unwired: 1 out]
  }
  n702 = while {
    stop <- w1510 stop-if-true
    n703 = case shown="True" "Autosave" {
      frame False {
      }
      frame True {
        n704 = control-ref of="This VI"() -> (w1517:refnum<vi>)
        n705 = property class="VI"(reference=w1517) -> ("Panel"=w1518:refnum<vi>)  [unwired: 1 in, 2 out]
        n706 = property on="Tab Control" class="TabCtl (strict)"() -> ("Pages"=w1515:refnum<vi>[])  [unwired: 2 in, 2 out]
        n707 = property class="Pnl"(reference=w1518) -> ("Controls[]"=w1514:refnum<vi>[])  [unwired: 1 in, 2 out]
        n708 = for {
          tunnel: [w1522] -> _ mode=indexing
          tunnel: w1515 -> [w1522] mode=indexing
          shift-right: [w1519] -> w1513
          shift-left: w1514 -> [w1521]
          n709 = property class="Page"(reference=w1522) -> ("Controls on Page[]"=w1520:refnum<vi>[])  [unwired: 1 in, 2 out]
          n710 = Insert Into Array(array=w1521, new element=w1520) -> (w1519:refnum<vi>[])  [unwired: 1 in]
        }
        n711 = for {
          tunnel: w1513 -> [w1526] mode=indexing
          tunnel: [w1525] -> w1512 mode=indexing
          tunnel: [w1523] -> w1511 mode=indexing
          n712 = property class="Ctl"(reference=w1526) -> ("Label.Text"=w1523:string)  [unwired: 1 in, 2 out]
          n713 = property class="Ctl"(reference=w1526) -> ("Value"=w1524:variant)  [unwired: 1 in, 2 out]
          n714 = Variant To Flattened String(Variant=w1524) -> (data string=w1525:string)  [unwired: 1 out]
        }
        "Array" <- w1511
        n715 = Write to Text File(file (use dialog)="autosave file", text=w1512) -> ()  [unwired: 2 in, 3 out]
      }
    }
    n716 = local read "Exit"() -> (w1510:bool)
    n717 = Multiply(x="Autosave every minutes", y=u32 60000) -> (x*y=w1509:u32)
    n718 = Wait Until Next ms Multiple(millisecond multiple=w1509) -> ()  [unwired: 1 out]
  }
